vi "Main_MnE.vi"() -> ()   [LabVIEW 2019]
uses:
  Devices/NI Board/cDAQ-9269 AO/Set_AO_Wave-config.ctl
  _ctrl/DL950_config.ctl
  _ctrl/BP4610_config.ctl
  _ctrl/DSP_config.ctl
  _ctrl/Error list.ctl
  _ctrl/cDAQ-9269 Config.ctl
  Devices/NI Board/cDAQ-9221 AI/Set_NIAI.ctl
  Durability/sequence_single.ctl
  Durability/Tap_main2.ctl
  Durability/Capacitor/error_rc.ctl
  Durability/Capacitor/measure_rc.ctl
  Durability/Capacitor/cap_config.ctl
  Durability/Breakdown-Spec.ctl
  Durability/Capacitor/Judge_RC.ctl
  Durability/common/Test Mode.ctl
  Durability/Register/data_contR.ctl
  Durability/Register/measure_reg.ctl
  Durability/common/result.ctl
  _ctrl/init-r-stop.ctl
  _ctrl/create-rw-close.ctl
  SubVIs/common/cmd_tablecnt.ctl
  Durability/common/cmd_ch act.ctl
  Durability/common/def_chact.ctl
  _ctrl/rw.ctl
  Durability/common/ref_all.ctl
  SubVIs/common/ref.ctl
  Durability/common/ui_dev-operator.ctl
  SubVIs/common/_ctrl/system-status.ctl
  _ctrl/init-r-w.ctl
  Durability/common/infor_testcycle.ctl
  Durability/common/cmd_TestParaSave.ctl
  Durability/common/UI dev-operator.ctl
  SubVIs/Log-in/cmd_logInfor.ctl
  _ctrl/start.ctl
  _ctrl/DSP_action.ctl
  _ctrl/BP4610_cmd.ctl
  _ctrl/init-w-close.ctl
  Devices/NI Board/cDAQ-9476 DO/cnt_do.ctl
  Devices/NI Board/cDAQ-9476 DO/cnt_Relay.ctl
  SubVIs/common/hw-control.ctl
  Durability/common/hwsetting.ctl
  SubVIs/cmd_timer.ctl
  _ctrl/fgv_DL950.ctl
  Durability/common/log save type.ctl
  Devices/NI Board/cDAQ-9269 AO/type_signal.ctl
  _ctrl/fgv_Main_q.ctl
  SubVIs/common/Glob_Ref.vi
  SubVIs/common/Glob_setting.vi
  Durability/common/Global 1.vi
  Durability/common/Global_params.vi
panel:
  in  "\"시험모드\" 파일이름 생성 무시(Ignore)":bool
  in  "ES 규격시험 선택":T1=enum."6.3.2 저온 작동/방치 시험"
  in  "paste":bool
  in  "copy":bool
  in  "Button":bool
  in  "Disabled":T2(ring)
  out "Label.Text":string
  in  "index":i32=1
  out "사이클 회수(현재)":u32
  out "사이클 회수(세팅)":u32
  out "종료시간":string
  out "경과시간":string
  out "시작시간":string
  out "HW error":T3
  out "H/W Status":string
  in  "debug":bool caption="."
  out "캡충전전압[V]":dbl(slide)=-0.07053543199999908 scale=0.0..800.0
  in  "Status":string
  out "반복 회수(세팅)":u32=1
  in  "PinR 4":bool
  in  "PinR 5":bool
  in  "PinR 6":bool
  in  "PoutR 4":bool
  in  "PoutR 5":bool
  in  "PoutR 6":bool
  out "ch 6":bool
  out "ch 5":bool
  out "ch 4":bool
  in  "Shutdown":bool
  in  "RC setting":bool
  in  "BP4610 off":bool
  in  "AO 0v":bool
  in  "BP4610 on":bool
  in  "AO 12v":bool
  in  "relay all off":bool
  in  "Graph":bool
  in  "set_DLM5058":bool
  in  "HW config":bool
  out "Waveform":cluster{"l":dbl, "dt":dbl, "Y":dbl[][]}(graph)
  out "채널":u8=1
  out "Operation stutus 0":bool
  in  "시험 모드":T4
  in  "저항부하":bool
  in  "캐패시터부하":bool
  in  "B-수명 1":bool
  in  "B-수명 2":bool
  in  "B-수명 3":bool
  out "dt(ms)_finish":u32
  out "dt(ms)_hw":u32
  in  "file renew[Hr]":i32
  in  "Main":bool
  in  "Stop_RC":bool
  in  "RCstart":bool
  in  "Oscilloscope_Res":cluster{"Record Len":i32, "Time Div":u16}={"Record Len"=4, "Time Div"=20} {"Time Div" items=["10m"=10, "20ms"=20, "50ms"=50, "100ms"=100, "200ms"=200, "500ms"=500, "1s"=1000, "2s"=2000]; "Record Len" items=["10k", "25k", "50k", "100k", "250k", "500k", "1M", "2.5M", "5M", "10M", "25M", "50M", "100M", "250M", "500M", "1G", "2G", "4G", "5G", "10G", "20G", "50G"]}
  in  "Control Signal_Res":T5={"Freq"=1.0, "level[V]"=12.0, "duty"=10.0, "On time[ms]"=300.0}
  in  "Oscilloscope_b1":cluster{"Record Len":i32, "Time Div":u16}={"Record Len"=4, "Time Div"=20} {"Time Div" items=["10m"=10, "20ms"=20, "50ms"=50, "100ms"=100, "200ms"=200, "500ms"=500, "1s"=1000, "2s"=2000]; "Record Len" items=["10k", "25k", "50k", "100k", "250k", "500k", "1M", "2.5M", "5M", "10M", "25M", "50M", "100M", "250M", "500M", "1G", "2G", "4G", "5G", "10G", "20G", "50G"]}
  in  "Control Signal_b1":T5={"Freq"=50.0, "level[V]"=12.0, "duty"=50.0, "On time[ms]"=50.0}
  in  "Control Signal_B2":T5={"Freq"=50.0, "level[V]"=12.0, "duty"=50.0, "On time[ms]"=50.0}
  in  "Oscilloscope_B2":cluster{"Record Len":i32, "Time Div":u16}={"Record Len"=4, "Time Div"=20} {"Time Div" items=["10m"=10, "20ms"=20, "50ms"=50, "100ms"=100, "200ms"=200, "500ms"=500, "1s"=1000, "2s"=2000]; "Record Len" items=["10k", "25k", "50k", "100k", "250k", "500k", "1M", "2.5M", "5M", "10M", "25M", "50M", "100M", "250M", "500M", "1G", "2G", "4G", "5G", "10G", "20G", "50G"]}
  in  "Control Signal_B3":T5={"Freq"=50.0, "level[V]"=12.0, "duty"=50.0, "On time[ms]"=50.0}
  in  "Oscilloscope_B3":cluster{"Record Len":i32, "Time Div":u16}={"Record Len"=4, "Time Div"=20} {"Time Div" items=["10m"=10, "20ms"=20, "50ms"=50, "100ms"=100, "200ms"=200, "500ms"=500, "1s"=1000, "2s"=2000]; "Record Len" items=["10k", "25k", "50k", "100k", "250k", "500k", "1M", "2.5M", "5M", "10M", "25M", "50M", "100M", "250M", "500M", "1G", "2G", "4G", "5G", "10G", "20G", "50G"]}
  in  "exit":bool
  in  "stop":bool
  in  "B3start":bool
  in  "B2start":bool
  in  "B1start":bool
  in  "Rloadstart":bool
  in  "single start":bool
  in  "Single sequence":T6
  in  "HW check":bool
  in  "Setting":bool
  in  "Tab_menu-select":T7=enum."Test"
  in  "Tab Control_manual":T8(tab)=enum."NI AI"
  in  "Output_LV":bool
  in  "led red":bool
  in  "led yellow":bool
  in  "led green":bool
  in  "led buz":bool
  in  "led purple":bool
  out "Voltage_Charge":dbl(slide)=-0.07053543199999908 scale=0.0..800.0
  in  "AO_Level":dbl caption="Level"
  in  "AO":bool
  in  "PinR 1":bool
  in  "PinR 2":bool
  in  "PinR 3":bool
  in  "PoutR 1":bool
  in  "PoutR 2":bool
  in  "PoutR 3":bool
  in  "Input Pwr":bool
  in  "Output_HV":bool
  in  "Discharge R":bool
  in  "Clear scope graph":bool
  in  "Trigger_single":bool
  in  "ReadItem_DLM5058":bool
  in  "ResetItem_DLM5058":bool
  in  "TabControl_DLM":enum32{" TEST DL950", " SET DL950", "Test_cmd"}(tab)=enum." SET DL950"
  out "DL950 items":dbl[][](array[numeric]) format="%.2f"
  out "DL950 wfm":waveform(dbl)[](graph)
  in  "DL950_config":T9={"Timeout"=0, "Time Div"=18, "Acq Mode"=0, "Record Len"=4, "Record Num"=0, "Start Point"=0, "End Poin"=60000, "Visa"="TCPIP0::192.168.0.101::inst0::INSTR", "Config Voltage"=[{"Enable"=TRUE, "Ch"=1, "V Div"=15, "Coupling"=1, "Probe"=35, "Act.Items"=FALSE, "items"=[]}, {"Enable"=TRUE, "Ch"=2, "V Div"=23, "Coupling"=1, "Probe"=35, "Act.Items"=FALSE, "items"=[]}, {"Enable"=TRUE, "Ch"=3, "V Div"=23, "Coupling"=1, "Probe"=35, "Act.Items"=FALSE, "items"=[]}, {"Enable"=TRUE, "Ch"=4, "V Div"=23, "Coupling"=1, "Probe"=35, "Act.Items"=FALSE, "items"=[]}, {"Enable"=TRUE, "Ch"=5, "V Div"=6, "Coupling"=1, "Probe"=3, "Act.Items"=FALSE, "items"=[]}, {"Enable"=TRUE, "Ch"=6, "V Div"=15, "Coupling"=1, "Probe"=21, "Act.Items"=FALSE, "items"=[]}], "Trigger on"=TRUE, "Trigger Level"=5.0, "Reset"=FALSE, "Config Temp"=[{"Channel"=9, "Burn Out"=FALSE, " Type "=0}, {"Channel"=10, "Burn Out"=FALSE, " Type "=0}, {"Channel"=11, "Burn Out"=FALSE, " Type "=0}, {"Channel"=12, "Burn Out"=FALSE, " Type "=0}, {"Channel"=13, "Burn Out"=FALSE, " Type "=0}, {"Channel"=14, "Burn Out"=FALSE, " Type "=0}], "Trig Mode"=0, "Trig Pos"=10.0, "Trigger Slope"=0, "Trigger Source "=1, "Trig Start -5"=-5.0, "End 5"=5.0} {"End 5" format="%.2g"; "Trig Start -5" format="%.2f"; "Trigger Source" items=["", "CH1", "CH2", "CH3", "CH4", "CH5", "CH6", "CH7", "CH8", "CH9", "CH10", "CH11", "CH12", "CH13", "CH14", "CH15", "CH16", "RMATH1", "RMATH2", "RMATH3", "RMATH4", "RMATH5", "RMATH6", "RMATH7", "RMATH8", "RMATH9", "RMATH10", "RMATH11", "RMATH12", "RMATH13", "RMATH14", "RMATH15", "RMATH16"]; "Trigger Slope" items=["Rising", "Falling", "Both"]; "Trig Pos" format="%.1f"; "Trig Mode" items=["Normal", "Auto", "Auto Level", "Single", "Single(N)", "On Start", "No Set"]; "Config Temp"."Type" items=["K", "E", "J", "T", "L", "U", "N", "R", "S", "B", "W", "Au7fe"]; "Config Temp"."Channel" items=["", "CH1", "CH2", "CH3", "CH4", "CH5", "CH6", "CH7", "CH8", "CH9", "CH10", "CH11", "CH12", "CH13", "CH14", "CH15", "CH16"]; "Trigger Level" format="%.3p"; "Config Voltage"."items" items=["Peak to Peak", "Amplitude", "Max", "Min", "High", "Low", "Average", "Middle", "Rms", "Standard Deviation", "+Overshoot", "-Overshoot", "Rise", "Fall", "Frequency", "Period", "+Width", "-Width", "Duty Cycle", "Pulse Count", "Burst1 Width", "Burst2 Width", "Average Frequency", "Average Period", "Int1TY", "Int2TY"]; "Config Voltage"."Probe" items=["1:1", "2:1", "5:1", "10:1", "20:1", "50:1", "100:1", "200:1", "500:1", "1000:1", "2000:1", "5000:1", "10k:1", "20k:1", "50k:1", "0.1A:1V", "0.2A:1V", "0.5A:1V", "1A:1V", "2A:1V", "5A:1V", "10A:1V", "20A:1V", "50A:1V", "100A:1V", "200A:1V", "250A:1V", "400A:1V", "500A:1V", "1kA:1V", "2kA:1V", "5kA:1V", "10kA:1V", "20kA:1V", "50kA:1V", "NoSet"]; "Config Voltage"."Ch" items=["None", "CH1", "CH2", "CH3", "CH4", "CH5", "CH6", "CH7", "CH8", "CH9", "CH10", "CH11", "CH12", "CH13", "CH14", "CH15", "CH16", "MATH1", "MATH2", "MATH3", "MATH4", "MATH5", "MATH6", "MATH7", "MATH8", "EVENT"]; "Config Voltage"."Coupling" items=["AC", "DC", "Ground", "AC-RMS", "DC-RMS"]; "Config Voltage"."V Div" items=["0.1m", "0.2m", "0.5m", "1m", "2m", "5m", "10m", "20m", "50m", "100m", "200m", "500m", "1", "2", "4", "5", "8", "10", "20", "40", "50", "80", "100", "200", "400", "500", "800", "1k", "2k", "4k", "5k", "8k", "10k", "20k", "25k", "50k", "100k", "250k", "500k", "1000k"]; "Record Len" items=["10k", "25k", "50k", "100k", "250k", "500k", "1M", "2.5M", "5M", "10M", "25M", "50M", "100M", "250M", "500M", "1G", "2G", "4G", "5G", "10G", "20G", "50G"]; "Acq Mode" items=["Normal", "Average", "Envelope"]; "Time Div" items=["100ns", "200ns", "500ns", "1us", "2us", "5us", "10us", "20us", "50us", "100us", "200us", "500us", "1ms", "2ms", "5ms", "10ms", "20ms", "50ms", "100ms", "200ms", "500ms", "1s", "2s", "3s", "4s", "5s", "6s", "10s", "20s", "30s", "1min", "2min", "3min", "4min", "5min", "6min", "10min", "12min", "30min", "1hour", "2hour", "3hour", "4hour", "5hour", "6hour", "8hour", "10hour", "12hour", "1day", "2day", "3day", "4day", "5day"]}
  out "Array_temp":T10(array[cluster])
  in  "Query_DLM5058":bool
  out "String_dl950":string
  in  "String":string
  out "DL950 read":dbl[](array[numeric])
  in  "Read":bool
  out "Time":dbl
  in  "con_DLM5058":bool
  in  "M_Start_DLM5058":bool
  in  "M_Stop_DLM5058":bool
  in  "Read_DLM5058":bool
  in  "discon_DLM5058":bool
  in  "Apply_DLM5058":bool
  in  "Apply BP4610":bool
  in  "Close BP4610":bool
  in  "Open BP4610":bool
  in  "BP4610 Config":T11={"VISA"="USB0::0x0D4A::0x0040::9426270::INSTR", "Limit-BP"={"Set"=enum."Voltage", "Voltage+[V]"=20.0, "Current+[A]"=5.0, "Voltage-[V]"=-20.0, "Current-[A]"=-5.0}, "SET BP"={"Set"=enum."Voltage", "Operation mode"=1, "Voltage[Vp-p]"=20.0, "Current[Ap-p]"=5.0, "Voltage[V]"=12.0, "Current[A]"=5.0, "Frequency[Hz]"=100.0, "Waveform"=enum."Square"}} {"SET BP"."Frequency[Hz]" min=1.0 max=100000.0 step=0.1; "SET BP"."Current[A]" min=-20.0 max=20.0 step=0.001; "SET BP"."Voltage[V]" min=-115.0 max=115.0 step=0.01; "SET BP"."Current[Ap-p]" min=0.0 max=60.0 step=0.01; "SET BP"."Voltage[Vp-p]" min=0.0 max=120.0 step=0.1; "SET BP"."Operation mode" items=["CV-INT", "CV-EXT", "CV-ADD", "CC-INT", "CC-EXT", "CC-ADD"]; "Limit-BP"."Current-[A]" min=-20.0 max=20.0 step=0.001; "Limit-BP"."Voltage-[V]" min=-115.0 max=115.0 step=0.01; "Limit-BP"."Current+[A]" min=0.0 max=60.0 step=0.01; "Limit-BP"."Voltage+[V]" min=0.0 max=120.0 step=0.1}
  in  "DSP Selection":enum32{"DSP HV", "DSP LV"}(radio)
  in  "DSP Config LV":T12={"Port"="TCPIP0::192.168.0.102::HISLIP0::INSTR", "OVP Level"=1000.0, "OCP Level"=25.0, "Current"=10.0, "Voltage"=200.0} {"OCP Level" format="%#_13g"; "OVP Level" format="%#_13g"}
  in  "read_dsp":bool
  in  "Close DSP":bool
  in  "Open DSP":bool
  in  "Set_idrc":bool
  out "Current":dbl
  out "Volt":dbl
  in  "DSP1500 Config":T12={"Port"="TCPIP0::192.168.0.102::HISLIP0::INSTR", "OVP Level"=1000.0, "OCP Level"=25.0, "Current"=10.0, "Voltage"=200.0} {"OCP Level" format="%#_13g"; "OVP Level" format="%#_13g"}
  in  "cDAQ 9269 AO config":T13={"Ch"="cDAQ9185-213AA55Mod2/ao0", "Max V"=5.0, "Min V"=-5.0, " Rate"=10000.0, "N pts"=2000, "sample mode"=10178} {"sample mode" items=["유한 샘플"=10178, "연속 샘플"=10123, "하드웨어 타이밍에 의한 단일 포인트"=12522]}
  in  "Ouptut_NIAO":bool
  in  "Apply AO":bool
  in  "AO_Wave-config":T14={"offset"=6.0, "Samples"=10000, "duty"=50.0, "Rate"=10000.0, "wfm"={"Freq"=50.0, "Amp"=6.0, "Type"=enum."Square Wave"}}
  out "Means":dbl[](array[numeric])=[-0.07053543199999908, -0.28297513060000157, -0.30258228640000107, -0.12714499130000104, -0.3520088408000025, -0.6333380023000008, -0.2967813385000024, 0.16819898919999848] format="%.3f"
  out "AI Graph":waveform(dbl)[](graph)=[{"t0"=timestamp(3812621198.0337114 s since 1904-01-01), "dt"=9.999999999999999e-05, "Y"=array[1000 elements], "attributes"=variant("NI_ChannelName"=variant(string "cDAQ9185-213AA55Mod3/ai0"), "NI_UnitDescription"=variant(string "Volts"))}, {"t0"=timestamp(3812621198.033723 s since 1904-01-01), "dt"=9.999999999999999e-05, "Y"=array[1000 elements], "attributes"=variant("NI_ChannelName"=variant(string "cDAQ9185-213AA55Mod3/ai1"), "NI_UnitDescription"=variant(string "Volts"))}, {"t0"=timestamp(3812621198.0337343 s since 1904-01-01), "dt"=9.999999999999999e-05, "Y"=array[1000 elements], "attributes"=variant("NI_ChannelName"=variant(string "cDAQ9185-213AA55Mod3/ai2"), "NI_UnitDescription"=variant(string "Volts"))}, {"t0"=timestamp(3812621198.0337453 s since 1904-01-01), "dt"=9.999999999999999e-05, "Y"=array[1000 elements], "attributes"=variant("NI_ChannelName"=variant(string "cDAQ9185-213AA55Mod3/ai3"), "NI_UnitDescription"=variant(string "Volts"))}, {"t0"=timestamp(3812621198.0337567 s since 1904-01-01), "dt"=9.999999999999999e-05, "Y"=array[1000 elements], "attributes"=variant("NI_ChannelName"=variant(string "cDAQ9185-213AA55Mod3/ai4"), "NI_UnitDescription"=variant(string "Volts"))}, {"t0"=timestamp(3812621198.0337677 s since 1904-01-01), "dt"=9.999999999999999e-05, "Y"=array[1000 elements], "attributes"=variant("NI_ChannelName"=variant(string "cDAQ9185-213AA55Mod3/ai5"), "NI_UnitDescription"=variant(string "Volts"))}, {"t0"=timestamp(3812621198.033779 s since 1904-01-01), "dt"=9.999999999999999e-05, "Y"=array[1000 elements], "attributes"=variant("NI_ChannelName"=variant(string "cDAQ9185-213AA55Mod3/ai6"), "NI_UnitDescription"=variant(string "Volts"))}, {"t0"=timestamp(3812621198.0337906 s since 1904-01-01), "dt"=9.999999999999999e-05, "Y"=array[1000 elements], "attributes"=variant("NI_ChannelName"=variant(string "cDAQ9185-213AA55Mod3/ai7"), "NI_UnitDescription"=variant(string "Volts"))}]
  in  "Stop_AI":bool
  in  "Read_AI":bool
  in  "cDAQ 9221 Config":T15={"input terminal"=10083, "minimum value"=-60.0, "maximum value"=60.0, "number of samples"=1000, "rate"=10000.0, "sample mode"=10123, "physical channels"="cDAQ9185-213AA55Mod3/ai0:7"} {"sample mode" items=["Finite Samples"=10178, "Continuous Samples"=10123, "Hardware Timed Single Point"=12522]; "rate" format="%0.2f"; "maximum value" format="%^.2e"; "minimum value" format="%^.2e"; "input terminal" items=["default"=-1, "RSE"=10083, "NRSE"=10078, "Differential"=10106, "Pseudodifferential"=12529]}
  in  "DO Initialize":bool
  in  "cDAQ-9467 Config":tag="cDAQ9185-213AA55Mod1/port0/line0:31"
  in  "Tab Control":T16(tab)
  out "DL950_config load":T9={"Timeout"=10000, "Time Div"=17, "Acq Mode"=0, "Record Len"=4, "Record Num"=0, "Start Point"=0, "End Poin"=1000, "Visa"="", "Config Voltage"=[{"Enable"=TRUE, "Ch"=1, "V Div"=26, "Coupling"=1, "Probe"=3, "Act.Items"=FALSE, "items"=[]}, {"Enable"=TRUE, "Ch"=2, "V Div"=20, "Coupling"=1, "Probe"=3, "Act.Items"=FALSE, "items"=[]}, {"Enable"=TRUE, "Ch"=3, "V Div"=20, "Coupling"=1, "Probe"=3, "Act.Items"=FALSE, "items"=[]}, {"Enable"=TRUE, "Ch"=4, "V Div"=20, "Coupling"=1, "Probe"=3, "Act.Items"=FALSE, "items"=[]}, {"Enable"=TRUE, "Ch"=5, "V Div"=20, "Coupling"=1, "Probe"=3, "Act.Items"=FALSE, "items"=[]}, {"Enable"=TRUE, "Ch"=6, "V Div"=20, "Coupling"=1, "Probe"=3, "Act.Items"=FALSE, "items"=[]}], "Trigger on"=FALSE, "Trigger Level"=0.0, "Reset"=FALSE, "Config Temp"=[{"Channel"=1, "Burn Out"=TRUE, " Type "=0}, {"Channel"=2, "Burn Out"=TRUE, " Type "=0}, {"Channel"=3, "Burn Out"=TRUE, " Type "=0}, {"Channel"=4, "Burn Out"=TRUE, " Type "=0}, {"Channel"=5, "Burn Out"=TRUE, " Type "=0}, {"Channel"=6, "Burn Out"=TRUE, " Type "=0}], "Trig Mode"=1, "Trig Pos"=50.0, "Trigger Slope"=0, "Trigger Source "=1, "Trig Start -5"=-5.0, "End 5"=5.0} {"End 5" format="%.2g"; "Trig Start -5" format="%.2f"; "Trigger Source" items=["", "CH1", "CH2", "CH3", "CH4", "CH5", "CH6", "CH7", "CH8", "CH9", "CH10", "CH11", "CH12", "CH13", "CH14", "CH15", "CH16", "RMATH1", "RMATH2", "RMATH3", "RMATH4", "RMATH5", "RMATH6", "RMATH7", "RMATH8", "RMATH9", "RMATH10", "RMATH11", "RMATH12", "RMATH13", "RMATH14", "RMATH15", "RMATH16"]; "Trigger Slope" items=["Rising", "Falling", "Both"]; "Trig Pos" format="%.1f"; "Trig Mode" items=["Normal", "Auto", "Auto Level", "Single", "Single(N)", "On Start", "No Set"]; "Config Temp"."Type" items=["K", "E", "J", "T", "L", "U", "N", "R", "S", "B", "W", "Au7fe"]; "Config Temp"."Channel" items=["", "CH1", "CH2", "CH3", "CH4", "CH5", "CH6", "CH7", "CH8", "CH9", "CH10", "CH11", "CH12", "CH13", "CH14", "CH15", "CH16"]; "Trigger Level" format="%.3p"; "Config Voltage"."items" items=["Peak to Peak", "Amplitude", "Max", "Min", "High", "Low", "Average", "Middle", "Rms", "Standard Deviation", "+Overshoot", "-Overshoot", "Rise", "Fall", "Frequency", "Period", "+Width", "-Width", "Duty Cycle", "Pulse Count", "Burst1 Width", "Burst2 Width", "Average Frequency", "Average Period", "Int1TY", "Int2TY"]; "Config Voltage"."Probe" items=["1:1", "2:1", "5:1", "10:1", "20:1", "50:1", "100:1", "200:1", "500:1", "1000:1", "2000:1", "5000:1", "10k:1", "20k:1", "50k:1", "0.1A:1V", "0.2A:1V", "0.5A:1V", "1A:1V", "2A:1V", "5A:1V", "10A:1V", "20A:1V", "50A:1V", "100A:1V", "200A:1V", "250A:1V", "400A:1V", "500A:1V", "1kA:1V", "2kA:1V", "5kA:1V", "10kA:1V", "20kA:1V", "50kA:1V", "NoSet"]; "Config Voltage"."Ch" items=["None", "CH1", "CH2", "CH3", "CH4", "CH5", "CH6", "CH7", "CH8", "CH9", "CH10", "CH11", "CH12", "CH13", "CH14", "CH15", "CH16", "MATH1", "MATH2", "MATH3", "MATH4", "MATH5", "MATH6", "MATH7", "MATH8", "EVENT"]; "Config Voltage"."Coupling" items=["AC", "DC", "Ground", "AC-RMS", "DC-RMS"]; "Config Voltage"."V Div" items=["0.1m", "0.2m", "0.5m", "1m", "2m", "5m", "10m", "20m", "50m", "100m", "200m", "500m", "1", "2", "4", "5", "8", "10", "20", "40", "50", "80", "100", "200", "400", "500", "800", "1k", "2k", "4k", "5k", "8k", "10k", "20k", "25k", "50k", "100k", "250k", "500k", "1000k"]; "Record Len" items=["10k", "25k", "50k", "100k", "250k", "500k", "1M", "2.5M", "5M", "10M", "25M", "50M", "100M", "250M", "500M", "1G", "2G", "4G", "5G", "10G", "20G", "50G"]; "Acq Mode" items=["Normal", "Average", "Envelope"]; "Time Div" items=["100ns", "200ns", "500ns", "1us", "2us", "5us", "10us", "20us", "50us", "100us", "200us", "500us", "1ms", "2ms", "5ms", "10ms", "20ms", "50ms", "100ms", "200ms", "500ms", "1s", "2s", "3s", "4s", "5s", "6s", "10s", "20s", "30s", "1min", "2min", "3min", "4min", "5min", "6min", "10min", "12min", "30min", "1hour", "2hour", "3hour", "4hour", "5hour", "6hour", "8hour", "10hour", "12hour", "1day", "2day", "3day", "4day", "5day"]}
  out "BP4610 Config load":T11={"VISA"="", "Limit-BP"={"Set"=enum."Current", "Voltage+[V]"=20.0, "Current+[A]"=5.0, "Voltage-[V]"=-20.0, "Current-[A]"=-5.0}, "SET BP"={"Set"=enum."FREQ/WAVE", "Operation mode"=0, "Voltage[Vp-p]"=0.0, "Current[Ap-p]"=0.0, "Voltage[V]"=0.0, "Current[A]"=0.0, "Frequency[Hz]"=1.0, "Waveform"=enum."Sine"}} {"SET BP"."Frequency[Hz]" min=1.0 max=100000.0 step=0.1; "SET BP"."Current[A]" min=-20.0 max=20.0 step=0.001; "SET BP"."Voltage[V]" min=-115.0 max=115.0 step=0.01; "SET BP"."Current[Ap-p]" min=0.0 max=60.0 step=0.01; "SET BP"."Voltage[Vp-p]" min=0.0 max=120.0 step=0.1; "SET BP"."Operation mode" items=["CV-INT", "CV-EXT", "CV-ADD", "CC-INT", "CC-EXT", "CC-ADD"]; "Limit-BP"."Current-[A]" min=-20.0 max=20.0 step=0.001; "Limit-BP"."Voltage-[V]" min=-115.0 max=115.0 step=0.01; "Limit-BP"."Current+[A]" min=0.0 max=60.0 step=0.01; "Limit-BP"."Voltage+[V]" min=0.0 max=120.0 step=0.1}
  out "DSP1950 Config load":T12={"Port"="TCPIP0::192.168.0.14::HISLIP0::INSTR", "OVP Level"=0.0, "OCP Level"=0.0, "Current"=0.0, "Voltage"=0.0} {"OCP Level" format="%#_13g"; "OVP Level" format="%#_13g"}
  out "DSP1950 Config LV":T12={"Port"="TCPIP0::192.168.0.14::HISLIP0::INSTR", "OVP Level"=0.0, "OCP Level"=0.0, "Current"=0.0, "Voltage"=0.0} {"OCP Level" format="%#_13g"; "OVP Level" format="%#_13g"}
  out "cDAQ-9221 Config":T15={"input terminal"=10083, "minimum value"=-60.0, "maximum value"=60.0, "number of samples"=1000, "rate"=10000.0, "sample mode"=10123, "physical channels"=""} {"sample mode" items=["Finite Samples"=10178, "Continuous Samples"=10123, "Hardware Timed Single Point"=12522]; "rate" format="%0.2f"; "maximum value" format="%^.2e"; "minimum value" format="%^.2e"; "input terminal" items=["default"=-1, "RSE"=10083, "NRSE"=10078, "Differential"=10106, "Pseudodifferential"=12529]}
  out "cDAQ-9467 Config load":tag
  out "cDAQ-9269 AO Config":T13={"Ch"="cDAQ1Mod1/ao0", "Max V"=5.0, "Min V"=-5.0, " Rate"=1000.0, "N pts"=100, "sample mode"=10178} {"sample mode" items=["유한 샘플"=10178, "연속 샘플"=10123, "하드웨어 타이밍에 의한 단일 포인트"=12522]}
  out "config 2":T13={"Ch"="cDAQ1Mod1/ao0", "Max V"=5.0, "Min V"=-5.0, " Rate"=1000.0, "N pts"=100, "sample mode"=10178} {"sample mode" items=["유한 샘플"=10178, "연속 샘플"=10123, "하드웨어 타이밍에 의한 단일 포인트"=12522]}
  out "AO_Wave-config load":T14
  in  "Tab Control_debug":enum32{"Main", "debug"}(tab)
  out "Operation Status 2":string
  out "스위칭 경과 시간(초)":dbl
  out "미작동 경과시간(초)":dbl format="%<%H:%M:%S%1u>t"
  out "스위칭 채널 개 수[N]":i32=1
  out "전체 사이클(%)":u8(slide)=255 scale=0.0..100.0
  out "작동시간(초)":dbl format="%<%H:%M:%S%1u>t"
  out "ch 1":bool
  out "ch 2":bool
  out "ch 3":bool
  in  "Multicolumn Listbox":i32(listbox)
  out "Operation Status":string
  out "1사이클 진행률(%)":u8(slide)=255 scale=0.0..100.0
  in  "Tab Control 2":T17(tab)
  out "read_dl950":string
  out "T2":dbl
  out "T1":dbl
  out "OCP Level":dbl
  out "OVP Level":dbl
  out "출력전류[A]":dbl
  out "출력전압[V]":dbl
  out "TestType":T6
  out "N pts":i32
  out "Min V":dbl
  out "Max V":dbl
  out "sample mode":i32(ring)=10178 caption="샘플 모드" items=["유한 샘플"=10178, "연속 샘플"=10123, "하드웨어 타이밍에 의한 단일 포인트"=12522]
  out "Rate":dbl
  out "Ch":tag
  out "DSP Selection 2":enum32{"DSP HV", "DSP LV"}(radio)
  out "da950_array":dbl[](array[numeric])
  out "result":T18=enum."Completion"
  out "950Trigger":i32 format="%.0x"
  out "OFF Time out":u32
  out "OFF Time in":u32
  out "NumData_OLV":dbl
  out "Control Signal_LV":T5={"Freq"=50.0, "level[V]"=12.0, "duty"=50.0, "On time[ms]"=50.0}
  out "Time Div_Init":u16
  out "Time Div_set":u16
  out "Time Div":u32
  out "trig delay":u32=3000
  out "trig delay_ready":u32=3000
  out "Testconfig out":T19={"Test Mode"=enum."6.3.2 저온 작동/방치 시험", "ON time[ms]"=500.0, "OFF time[ms]"=10000.0, "1. 작동시간[분]"=10000.0, "2. 미작동시간[분]"=10000.0, "3. 작동시간[분]"=10000.0, "level[V]"=12.0, "duty"=20.0, "Freq"=1.0, "Voltage+[V]"=20.0, "Voltage-[V]"=-20.0, "Current+[A]"=5.0, "Current-[A]"=-5.0, "출력전압[V]"=0.0, "출력전류[A]"=0.0, "OVP Level"=0.0, "OCP Level"=0.0, "Time Div"=0, "Record Len"=4, "방전 기준[V]"=0.0, "Repeate (Each Ch)"=1, "Cycle[N]"=1, "작동간격[분]"=10000.0, "TrigPos[%]"=0.0, "시험시간[분]"=10000.0} {"시험시간[분]" min=1.0; "작동간격[분]" min=1.0; "3. 작동시간[분]" min=1.0; "2. 미작동시간[분]" min=1.0; "1. 작동시간[분]" min=1.0; "Time Div" items=["10m", "20ms", "50ms", "100ms", "200ms", "500ms", "1s", "2s", "5s", "10s", "20s", "30s", "1min", "2min", "5min"]; "OFF time[ms]" min=10000.0 max=1000000.0; "Current-[A]" min=-20.0 max=20.0 step=0.001; "Voltage-[V]" min=-115.0 max=115.0 step=0.01; "Current+[A]" min=0.0 max=60.0 step=0.01; "Voltage+[V]" min=0.0 max=120.0 step=0.1; "OCP Level" format="%#_13g"; "OVP Level" format="%#_13g"; "Record Len" items=["10k", "25k", "50k", "100k", "250k", "500k", "1M", "2.5M", "5M", "10M", "25M", "50M", "100M", "250M", "500M", "1G", "2G", "4G", "5G", "10G", "20G", "50G"]; "ON time[ms]" min=50.0 max=2000000.0}
  out "measure_LV 동작":T20
  out "measure_rc 동작":T21 {"부하전압(고장)" format="%.3f"; "출력전류 평균 63%" format="%.3f"; "출력전압 - 평균 63%" format="%.3f"; "Failing Time 37%" format="%.3f"; "Rising Time 98%" format="%.3f"; "Rising Time 63%" format="%.3f"; "접촉저항" format="%.1f"; "출력전류 RMS" format="%.3f"; "출력전압 + 평균 63%" format="%.3f"; "입력전류 RMS" format="%.3f"; "온도" format="%.3f"; "방전전압" format="%.3f"; "충전전류 37초" format="%.3f"; "충전전압 63초" format="%.3f"; "충전전압 98초" format="%.3f"; "출력카운트" format="%.3f"; "입력카운트" format="%.3f"}
  out "measure_ContR Out":T22
  out "Error":T23
  out "AO Waveform Graph":waveform(dbl)(graph)
  out "error out":errorcluster
  out "error out wait Ao":errorcluster
  out "error out task stop":errorcluster
  out "data_relay":bool[](array[boolean])
  in  "시험환경세팅":bool
  in  "시험규격":bool
  in  "Apply":bool
  in  "Password":string
  in  "logout":bool
  in  "login":bool
  in  "Log path":path=path "C:/test_cfg"
  in  "시험명":string="relay"
  in  "Breakdown-Spec":T24={"제어단 단선 Irms[mA](이하)"=5.0, "제어단 특성 전류 Irms[mA] Max"=50.0, "제어단 특성 전류 Irms[mA] Min"=10.0, "출력단 단선 Irms[mA](이하)"=5.0, "출력단 특성 전류 Irms[mA]  Max"=3700.0, "출력단 특성전류 Irms[mA]  Min"=1000.0, "온도[degree]"=0.0} {"출력단 특성전류 Irms[mA]  Min" format="%#.2f"; "출력단 특성 전류 Irms[mA]  Max" format="%#.2f"; "출력단 단선 Irms[mA](이하)" format="%#.2f"; "제어단 특성 전류 Irms[mA] Min" format="%#.2f"; "제어단 특성 전류 Irms[mA] Max" format="%#.2f"; "제어단 단선 Irms[mA](이하)" format="%#.2f"}
  in  "Testconfig":T19={"Test Mode"=enum."6.3.2 저온 작동/방치 시험", "ON time[ms]"=200.0, "OFF time[ms]"=500.0, "1. 작동시간[분]"=10000.0, "2. 미작동시간[분]"=10000.0, "3. 작동시간[분]"=10000.0, "level[V]"=12.0, "duty"=20.0, "Freq"=1.0, "Voltage+[V]"=20.0, "Voltage-[V]"=-20.0, "Current+[A]"=5.0, "Current-[A]"=-5.0, "출력전압[V]"=200.0, "출력전류[A]"=10.0, "OVP Level"=0.0, "OCP Level"=0.0, "Time Div"=2, "Record Len"=5, "방전 기준[V]"=0.0, "Repeate (Each Ch)"=3, "Cycle[N]"=1, "작동간격[분]"=10000.0, "TrigPos[%]"=0.0, "시험시간[분]"=1.0} {"시험시간[분]" min=1.0; "작동간격[분]" min=1.0; "3. 작동시간[분]" min=1.0; "2. 미작동시간[분]" min=1.0; "1. 작동시간[분]" min=1.0; "Time Div" items=["10m", "20ms", "50ms", "100ms", "200ms", "500ms", "1s", "2s", "5s", "10s", "20s", "30s", "1min", "2min", "5min"]; "OFF time[ms]" min=10000.0 max=1000000.0; "Current-[A]" min=-20.0 max=20.0 step=0.001; "Voltage-[V]" min=-115.0 max=115.0 step=0.01; "Current+[A]" min=0.0 max=60.0 step=0.01; "Voltage+[V]" min=0.0 max=120.0 step=0.1; "OCP Level" format="%#_13g"; "OVP Level" format="%#_13g"; "Record Len" items=["10k", "25k", "50k", "100k", "250k", "500k", "1M", "2.5M", "5M", "10M", "25M", "50M", "100M", "250M", "500M", "1G", "2G", "4G", "5G", "10G", "20G", "50G"]; "ON time[ms]" min=50.0 max=2000000.0}
  in  "Test Judgement":T25={"전압 63%[mS] Min"=25.5, "전압 98%[mS] Min"=140.0, "전류 37%[mS] Min"=25.5, "접촉저항[mOhm] Min"=1.0, "출력전류 Irms[mA] Min"=1500.0, "전압 63%[mS] Max"=5.0, "전압 98%[mS] Max"=5.0, "전류 37%[mS] Max"=5.0, "접촉저항[mOhm] Max"=0.5, "출력전류 Irms[mA] Max"=500.0}
  in  "채널선택":T26={"Ch 1"=TRUE, "Ch 2"=TRUE, "Ch 3"=TRUE, "Ch 4"=TRUE, "Ch 5"=TRUE, "Ch 6"=TRUE}
  in  "Manual":bool
  # "운영 상태"
  # "Pre Charge Relay 메카환경 신뢰성"
  # "ver.02"
  # "캡 충전 상태"
  # "시스템 로그"
  # "시간 정보"
  # "ES 규격 시험 정보"
  # "Relay4"
  # "Relay5"
  # "Relay6"
  # "디바이스 상태"
  # "C 전압1"
  # "C 전압2"
  # "출력전압(+)"
  # "출력전압(-)"
  # "입력전류"
  # "출력전류"
  # "Limit-BP\nV+ 20 C 5\nV- -20 C- -5\n\nSET BP\nVp 20, C 5, Square\nV 12, C5, 100"
  # "102::HISLIP0::INSTR\n\nOVP 1000, OCP 25\nV 400, C 20"
  # "102::HISLIP0::INSTR\n\nOVP 1000, OCP 25\nV 400, C 20"
  # "a0\n5\n-5\n10000\n5000\n유한샘플"
  # "10000, W freq 50\n10000, Amp 6\n6, Square\n50"
  # "RSE\n-60\n60\n1000\n10000\nCont"
  # "C 전압1"
  # "C 전압2"
  # "출력전압(+)"
  # "출력전압(-)"
  # "입력전류"
  # "출력전류"
  # "채널 스위칭 정보"
  # "작동/미작동 시간(초)"
  # "시험 진행률"
  # "제어단 전압"
  # "출력단 전원"
  # "DL950"
  # "Discharge"
  # "Test Cycle"
  # "작동 설정"
  # "R Laoad"
  # "R out1"
  # "R out2"
  # "R out3"
  # "R out4"
  # "R out5"
  # "R out6"
  # "R in1"
  # "R in2"
  # "R in3"
  # "R in4"
  # "R in5"
  # "R in6"
  # "Red"
  # "Yellow"
  # "Green"
  # "Buz"
  # "Purple"
  # "관리자 기능"
  # "데이터 저장"
  # "고장진단 기준"
  # "테스트 환경"
  # "테스트 체널"
  # "테스트 기준"
  # "제어단"
  # "출력단"
  # "온도기준"
  # "제어단 전압"
  # "출력단 전원"
  # "DL950"
  # "Discharge"
  # "Test Cycle"
  # "작동 설정"
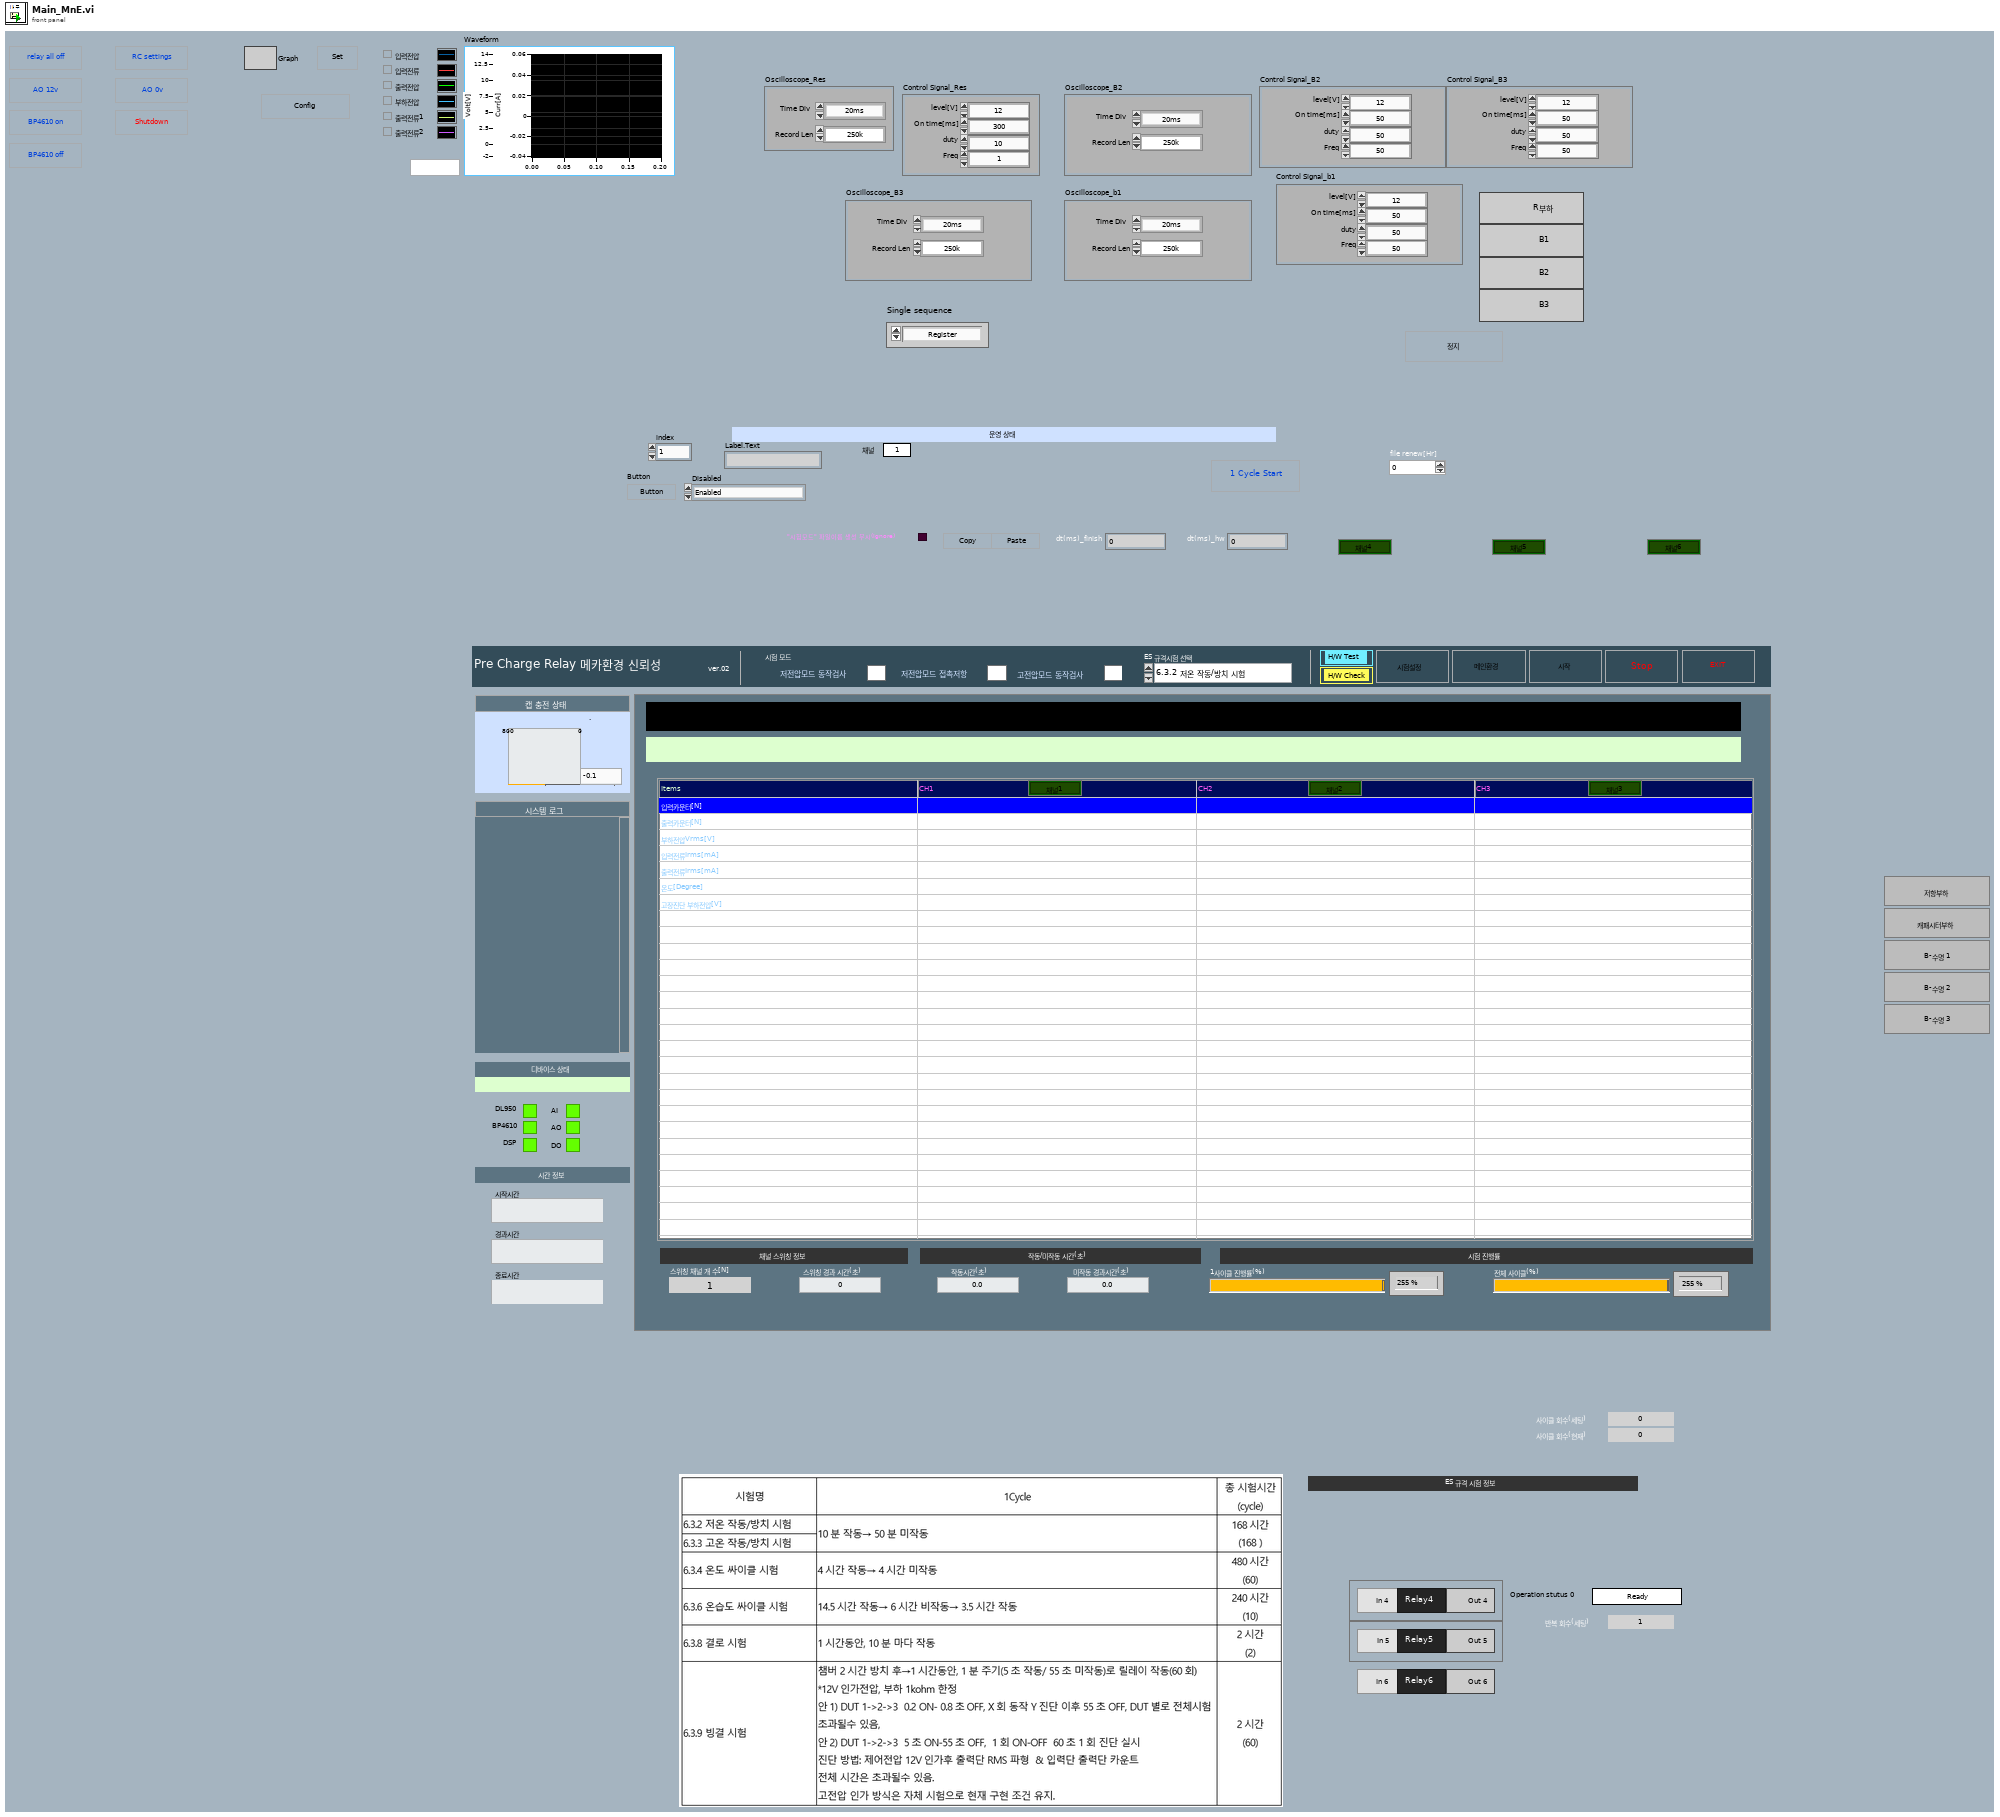
[diagram p1: front panel]
types:
  T1 = typedef "시험모드선택.ctl" = enum16{"6.3.1 온도방치 시험", "6.3.2 저온 작동/방치 시험", "6.3.3 고온 작동/방치 시험", "6.3.4 온도 싸이클 시험", "6.3.6 온습도 싸이클 시험", "6.3.7 고온고습 방치", "6.3.8 결로 시험", "6.3.9 빙결시험", "6.3.10 공진", "6.3.11.1 작동가진", "6.3.11.2 비작동 가진 ", "6.3.12 충격시험"}
  T2 = enum8{"Enabled", "Disabled", "Disabled and Grayed Out"}
  T3 = typedef "Error list.ctl" = cluster{"DL950":bool, "BP4610":bool, "DSP":bool, "AI":bool, "AO":bool, "DO":bool}
  T4 = typedef "Test Mode.ctl" = enum32{"저항부하", "캐패시터부하", "B수명 - 1", "B수명 - 2", "B수명 - 3", "저전압모드 동작검사", "저전압모드 접촉저항", "고전압모드 동작검사"}
  T5 = cluster{"Freq":dbl, "level[V]":dbl, "duty":dbl, "On time[ms]":dbl}
  T6 = typedef "sequence_single.ctl" = enum16{"Register", "RC", "B1", "B2", "B3", "Oper_LV", "Oper_HV", "ContR_LV"}
  T7 = typedef "Tap_main2.ctl" = enum32{"Manual", "Test", "Setting"}
  T8 = enum32{"System Config", "OSCILL", "INPUT", "OUTPUT", "NI AO ", "NI AI", "NI DO", "Load Config"}
  T9 = typedef "DL950_config.ctl" = cluster{"Timeout":u32, "Time Div":i32, "Acq Mode":i32, "Record Len":i32, "Record Num":i32, "Start Point":i64, "End Poin":i64, "Visa":refnum<visa-resource-name>, "Config Voltage":cluster{"Enable":bool, "Ch":u16, "V Div":i32, "Coupling":i32, "Probe":i32, "Act.Items":bool, "items":i32[]}[], "Trigger on":bool, "Trigger Level":dbl, "Reset":bool, "Config Temp":cluster{"Channel":u16, "Burn Out":bool, " Type ":i32}[], "Trig Mode":i32, "Trig Pos":dbl, "Trigger Slope":i32, "Trigger Source ":i32, "Trig Start -5":dbl, "End 5":dbl}
  T10 = cluster{"Channel":u16, "Burn Out":bool, " Type ":i32}[]
  T11 = typedef "BP4610_config.ctl" = cluster{"VISA":refnum<visa-resource-name>, "Limit-BP":cluster{"Set":enum16{"Current", "Voltage"}, "Voltage+[V]":dbl, "Current+[A]":dbl, "Voltage-[V]":dbl, "Current-[A]":dbl}, "SET BP":cluster{"Set":enum16{"Current", "Voltage", "FREQ/WAVE"}, "Operation mode":u16, "Voltage[Vp-p]":dbl, "Current[Ap-p]":dbl, "Voltage[V]":dbl, "Current[A]":dbl, "Frequency[Hz]":dbl, "Waveform":enum16{"Sine", "Square", "ARB 1", "ARB 2", "ARB 3", "ARB 4", "ARB 5", "ARB 6", "ARB 7", "ARB 8", "ARB 9", "ARB 10", "ARB 11", "ARB 12", "ARB 13", "ARB 14", "ARB 15", "ARB 16"}}}
  T12 = typedef "DSP_config.ctl" = cluster{"Port":refnum<visa-resource-name>, "OVP Level":dbl, "OCP Level":dbl, "Current":dbl, "Voltage":dbl}
  T13 = typedef "cDAQ-9269 Config.ctl" = cluster{"Ch":tag, "Max V":dbl, "Min V":dbl, " Rate":dbl, "N pts":i32, "sample mode":i32}
  T14 = typedef "Set_AO_Wave-config.ctl" = cluster{"offset":dbl, "Samples":i32, "duty":dbl, "Rate":dbl, "wfm":cluster{"Freq":dbl, "Amp":dbl, "Type":enum16{"Sine Wave", "Triangle Wave", "Square Wave", "Sawtooth Wave"}}}
  T15 = typedef "Set_NIAI.ctl" = cluster{"input terminal":i32, "minimum value":dbl, "maximum value":dbl, "number of samples":i32, "rate":dbl, "sample mode":i32, "physical channels":tag}
  T16 = enum32{"dl950", "BP4610", "DSP", "cDAQ-9221 ", "cDAQ-9467", "cDAQ-9269", "AO_Wave-config"}
  T17 = enum32{"debug", "conditions", "data gethering", "NI "}
  T18 = typedef "result.ctl" = enum16{"Init", "OK", "NG", "Shutdown", "Testing", "Completion", "Device Error", "Start", "작동", "미작동", "작동 대기", "작동 1"}
  T19 = typedef "cap_config.ctl" = cluster{"Test Mode":T1, "ON time[ms]":dbl, "OFF time[ms]":dbl, "1. 작동시간[분]":dbl, "2. 미작동시간[분]":dbl, "3. 작동시간[분]":dbl, "level[V]":dbl, "duty":dbl, "Freq":dbl, "Voltage+[V]":dbl, "Voltage-[V]":dbl, "Current+[A]":dbl, "Current-[A]":dbl, "출력전압[V]":dbl, "출력전류[A]":dbl, "OVP Level":dbl, "OCP Level":dbl, "Time Div":u16, "Record Len":i32, "방전 기준[V]":dbl, "Repeate (Each Ch)":u32, "Cycle[N]":u32, "작동간격[분]":dbl, "TrigPos[%]":dbl, "시험시간[분]":dbl}
  T20 = typedef "measure_reg.ctl" = cluster{"입력카운트":dbl, "출력카운트":dbl, "부하전압 RMS":dbl, "입력전류 RMS":dbl, "출력전류 RMS":dbl, "온도":dbl, "부하전압(고장)":dbl}
  T21 = typedef "measure_rc.ctl" = cluster{"입력카운트":dbl, "출력카운트":dbl, "Rising Time 63%":dbl, "Rising Time 98%":dbl, "Failing Time 37%":dbl, "입력전류 RMS":dbl, "출력전류 RMS":dbl, "출력전압 + 평균 63%":dbl, "출력전압 - 평균 63%":dbl, "출력전류 평균 63%":dbl, "접촉저항":dbl, "온도":dbl, "방전전압":dbl, "부하전압(고장)":dbl, "충전전압 63초":dbl, "충전전압 98초":dbl, "충전전류 37초":dbl, "전압강하":dbl}
  T22 = typedef "data_contR.ctl" = cluster{"입력카운트":dbl, "출력카운트":dbl, "입력전류 RMS":dbl, "출력전류 RMS":dbl, "출력전압(+)_Avg":dbl, "출력전압(-)_Avg":dbl, "출력전류_Avg":dbl, "접촉저항":dbl, "온도":dbl, "부하전압":dbl}
  T23 = typedef "error_rc.ctl" = cluster{"제어단 단선":bool, "제어단 단락":bool, "제어단 특성변화":bool, "출력단 단선":bool, "출력단 단락":bool, "출력단 특성변화":bool, "출력전압":bool, "카운트 일치":bool, "전압 98%":bool, "전압 63%":bool, "전류 37%":bool, "방전전압":bool, "온도":bool}
  T24 = typedef "Breakdown-Spec.ctl" = cluster{"제어단 단선 Irms[mA](이하)":dbl, "제어단 특성 전류 Irms[mA] Max":dbl, "제어단 특성 전류 Irms[mA] Min":dbl, "출력단 단선 Irms[mA](이하)":dbl, "출력단 특성 전류 Irms[mA]  Max":dbl, "출력단 특성전류 Irms[mA]  Min":dbl, "온도[degree]":dbl}
  T25 = typedef "Judge_RC.ctl" = cluster{"전압 63%[mS] Min":dbl, "전압 98%[mS] Min":dbl, "전류 37%[mS] Min":dbl, "접촉저항[mOhm] Min":dbl, "출력전류 Irms[mA] Min":dbl, "전압 63%[mS] Max":dbl, "전압 98%[mS] Max":dbl, "전류 37%[mS] Max":dbl, "접촉저항[mOhm] Max":dbl, "출력전류 Irms[mA] Max":dbl}
  T26 = cluster{"Ch 1":bool, "Ch 2":bool, "Ch 3":bool, "Ch 4":bool, "Ch 5":bool, "Ch 6":bool}
  T27 = typedef "create-rw-close.ctl" = enum16{"create", "write", "read", "delete", "close"}
  T28 = enum16{"yellow", "red", "green", "buzz1", "buzz2"}
  T29 = typedef "init-r-stop.ctl" = enum16{"ini", "read", "stop"}
  T30 = typedef "cmd_tablecnt.ctl" = enum16{"Create", "Inital", "Write", "Default"}
  T31 = typedef "cmd_ch act.ctl" = enum16{"open", "initial", "update"}
  T32 = typedef "def_chact.ctl" = cluster{"ch 1":refnum<vi>, "ch 2":refnum<vi>, "ch 3":refnum<vi>, "ch 4":refnum<vi>, "ch 5":refnum<vi>, "ch 6":refnum<vi>}
  T33 = typedef "ref_all.ctl" = cluster{"BP4610 Config":refnum<vi>, "DSP1950 Config":refnum<vi>, "2470-config":refnum<vi>, "cDAQ 9269 AO config":refnum<vi>, "cDAQ 9221 Config":refnum<vi>, "cDAQ-9467 Config":refnum<vi>, "Waveform":refnum<vi>, "DL950 wfm":refnum<vi>, "AI Graph":refnum<vi>, "AO_Wave-config":refnum<vi>, "DL950 items":refnum<vi>, "Volt":refnum<vi>, "Current":refnum<vi>, "AO_Level":refnum<vi>, "RC-Test Judgement ":refnum<vi>, "Log path":refnum<vi>, "시험명":refnum<vi>, "file renew[Hr]":refnum<vi>, "Breakdown-Spec":refnum<vi>, "paste":refnum<vi>, "copy":refnum<vi>, "DL950_config":refnum<vi>, "종료시간":refnum<vi>, "경과시간":refnum<vi>, "Apply":refnum<vi>, "DSP Config LV ":refnum<vi>, "Testconfig":refnum<vi>}
  T34 = typedef "rw.ctl" = enum16{"read", "write"}
  T35 = typedef "ref.ctl" = cluster{"relay 1":refnum<vi>, "relay 2":refnum<vi>, "relay 3":refnum<vi>, "relay 4":refnum<vi>, "relay 5":refnum<vi>, "relay 6":refnum<vi>, "PoutR 1":refnum<vi>, "PoutR 2":refnum<vi>, "PoutR 3":refnum<vi>, "PoutR 4":refnum<vi>, "PoutR 5":refnum<vi>, "PoutR 6":refnum<vi>, "Discharge":refnum<vi>, "Input Pwr":refnum<vi>, "Output_HV":refnum<vi>, "AO onoff":refnum<vi>}
  T36 = typedef "ui_dev-operator.ctl" = cluster{"Operation stutus":refnum<vi>, "Test Status":refnum<vi>, "Setting":refnum<vi>, "Manual":refnum<vi>, "Main":refnum<vi>, "RCstart":refnum<vi>, "채널선택":refnum<vi>, "시험명":refnum<vi>, "Tab Control_manual":refnum<vi>, "시험 모드":refnum<vi>, "HW check":refnum<vi>, "login":refnum<vi>, "logout":refnum<vi>}
  T37 = enum16{"Config Save", "Config Load", "LastRUN Save", "LastRUN Load"}
  T38 = typedef "system-status.ctl" = enum16{"Initial", "Update", "Clear", "Read"}
  T39 = typedef "init-r-w.ctl" = enum16{"init", "read", "write"}
  T40 = typedef "cmd_TestParaSave.ctl" = enum16{"Save", "Read", "Idle"}
  T41 = typedef "infor_testcycle.ctl" = cluster{"Channel selection":cluster{"1ch":bool, "2ch":bool, "3ch":bool, "4ch":bool, "5ch":bool, "6ch":bool}, "Test Cycle":u32, "Repeate":u32}
  T42 = typedef "cmd_logInfor.ctl" = enum16{"ADMIN", "OPER", "DEFAULT"}
  T43 = typedef "UI dev-operator.ctl" = enum16{"Testing", "Admin", "Operator", "Finish", "Ready"}
  T44 = typedef "start.ctl" = enum16{"init", "open", "set", "start", "stop", "read", "read_items", "query", "close", "T_single", "reset", "exit"}
  T45 = typedef "DSP_action.ctl" = enum16{"False", "cont", "on", "off", "discont", "protection", "protection_seq", "preread", "level_seq", "level_m", "read", "stop", "exit"}
  T46 = typedef "BP4610_cmd.ctl" = enum16{"open", "read", "set", "set_seq", "limit", "limit_seq", "output on", "output off", "close"}
  T47 = typedef "init-w-close.ctl" = enum16{"open", "init", "write", "close"}
  T48 = typedef "cnt_do.ctl" = enum16{"open", "initial", "update", "run", "close"}
  T49 = typedef "cnt_Relay.ctl" = enum32{"R_Load", "R_out1", "R_out2", "R_out3", "R_out4", "R_out5", "R_out6", "R8", "R9", "R10", "R11", "R12", "R13", "R14", "R15", "R16", "R_in1", "R_in2", "R_in3", "R_in4", "R_in5", "R_in6", "R23", "R24", "R25", "R26", "R27", "R_red", "R_yellow", "R_green", "R_buz", "R_purple"}
  T50 = typedef "hw-control.ctl" = enum16{"DL950 ready", "DL950 clear", "DL950 trigger", "DL950 read", "DL950 read seq", "DL950 Tsingle query", "AO 12v", "AO wave", "AO 0v", "relay all-off", "Discharge check", "Discharge", "Relay1", "Relay2", "Relay3", "Relay4", "Relay5", "Relay6", "BP4610 onoff", "BP4610 set", "DSP1500 set", "DSP1500 onoff"}
  T51 = typedef "hwsetting.ctl" = enum16{"BP4610 RC", "DSP1500 RC", "AO"}
  T52 = typedef "cmd_timer.ctl" = enum16{"init", "init_update", "run", "default", "update"}
  T53 = enum32{"6.3.2 저온 작동/방치 시험", "6.3.3 고온 작동/방치 시험", "6.3.4 온도 싸이클 시험", "6.3.6 온습도 싸이클 시험", "6.3.8 결로 시험", "6.3.9 빙결 시험"}
  T54 = typedef "fgv_DL950.ctl" = enum16{"init", "config", "Set-NCh", "setapply", "trigger", "history_clear", "read", "time-div", "wave-aquis", "start", "query", "abort", "set_items", "reset_items", "read_items", "percent_rise", "trigger_single", "stop", "offset cancel", "close"}
  T55 = typedef "log save type.ctl" = enum16{"header", "data"}
  T56 = typedef "type_signal.ctl" = enum16{"wave", "level"}
  T57 = typedef "fgv_Main_q.ctl" = enum16{"init", "wait", "R", "RC", "RC_M", "B1", "B2", "B3", "exit"}
  T58 = enum32{"Invalid", "Standard", "Closed", "Hidden", "Minimized", "Maximized"}
  T59 = typedef "Tpye_ParaAll.ctl" = cluster{"DL950_config":T9, "BP4610 Config":T11, "DSP1950 Config":T12, "DMM 2470 Config":cluster{"Source Mode":enum16{"Voltage", "Current"}, "Source Limit Level":dbl, "Source Level":dbl, "Output_2470":bool}, "cDAQ-9221 Config":T15, "cDAQ-9467 Config":tag, "cDAQ-9269 AO Config":T13, "AO_Wave-config":T14, "DSP1950 Config LV":T12}
  T60 = typedef "config_aging.ctl" = cluster{"Setting":T61, "TestName":string, "Result path":path, "파일 생성 주기[N]":u8, "Test Specs":T24}
  T61 = typedef "Setting_reg.ctl" = cluster{"제어 전압[V]":dbl, "출력전압[V]":dbl, "전류[A]":dbl, "출력전류[A]":dbl, "ON[초]":dbl, "OFF[초]":dbl, "Irms 허용치 from ":dbl, "Irms 허용치 to":dbl, "AO Delay ms":u32, "Log":path, "result":path}
  T62 = typedef "Testing-info.ctl" = cluster{"전체채널수":u8, "현재채널번호":u8, "Irms":dbl, "입력전압":dbl, "입력전류":dbl, "출력전압":dbl, "출력전류":dbl, "온도":dbl, "제어단 단선":bool, "제어단 단락":bool, "제어단 특성변화":bool, "출력단 단선":bool, "출력단 단락":bool, "출력단 특성변화":bool, "출력단 전압":bool, "카운트 일치":bool, "Irms 판정":bool, "온도":bool, "테스트 회수":u32, "TestType":T6, "현재회수":u32, "Ch selection":cluster{"1ch":bool, "2ch":bool, "3ch":bool, "4ch":bool, "5ch":bool, "6ch":bool}, "반복":u32, "Path":path, "파일생성주기":u32, "start time":dbl, "stop time":dbl, "현재반복회수":u32, "NG":cluster{"입출력 카운트":bool, "출력전류RMS":bool}}
  T63 = cluster{"1ch":bool, "2ch":bool, "3ch":bool, "4ch":bool, "5ch":bool, "6ch":bool}
  T64 = enum32{"Bad", "Idle", "Run top level", "Running"}
  T65 = typedef "DL950_wfms.ctl" = cluster{"wfms":waveform(dbl)[], "Waveform_2":cluster{"t0":dbl, "dt":dbl, "Y":dbl[][]}, "items":dbl[][], "da950_array":dbl[]}
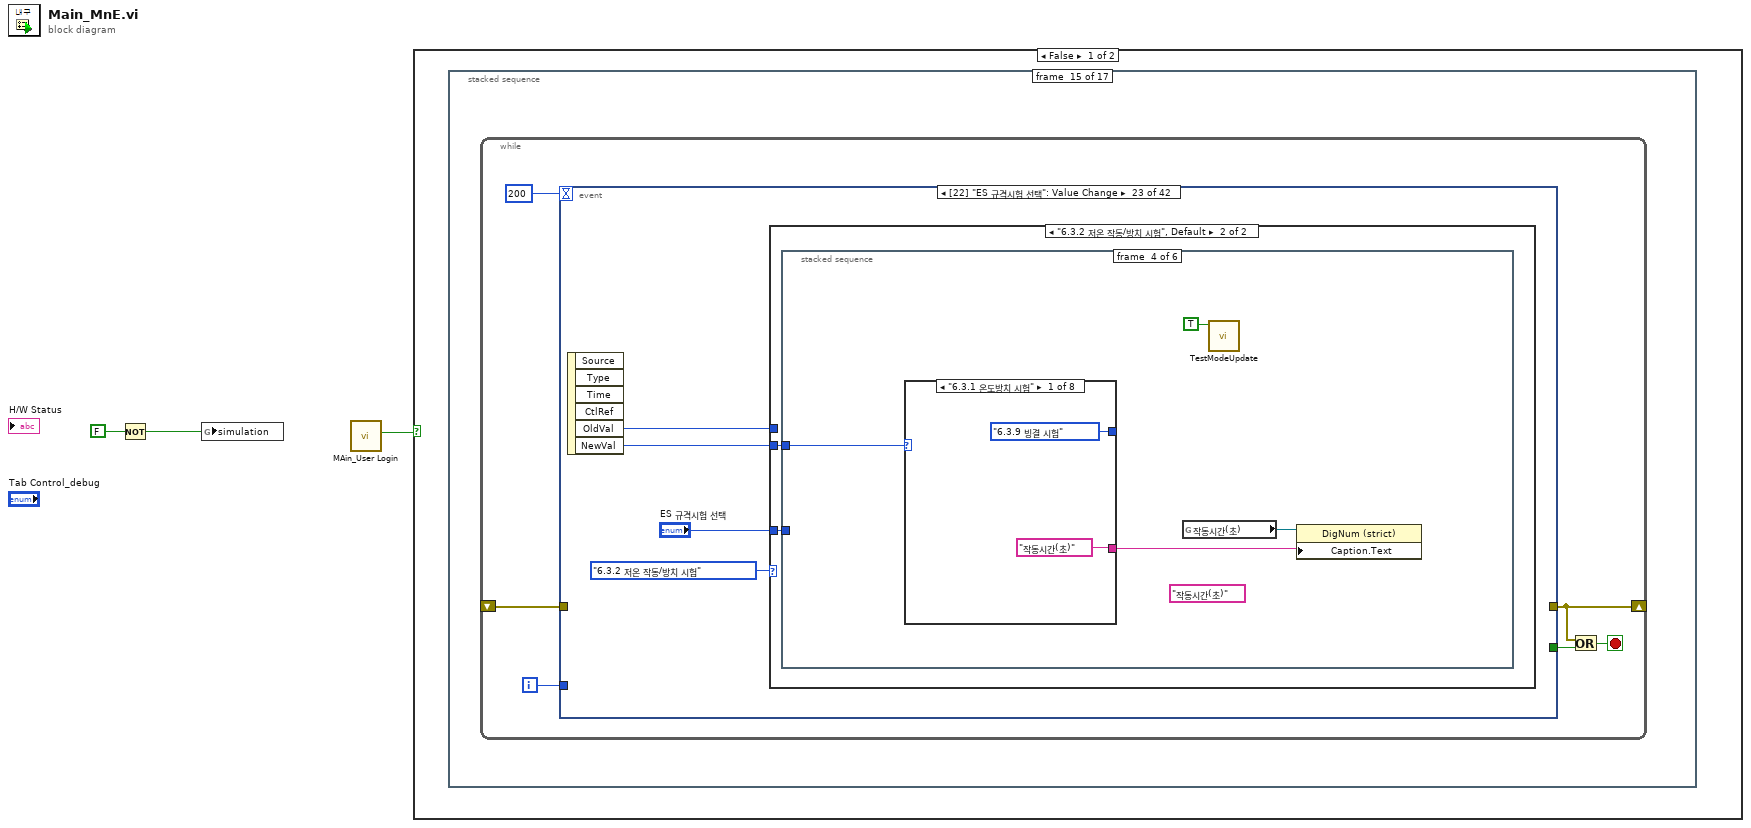
[diagram p0: block diagram]
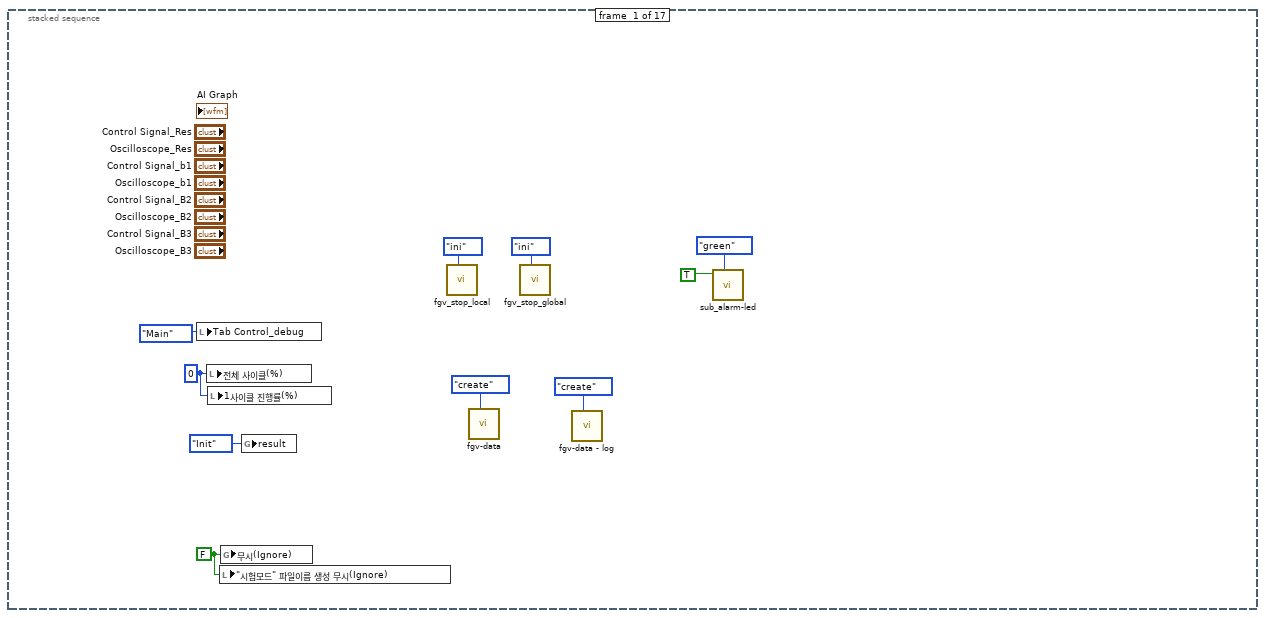
[diagram p2: hidden frame]
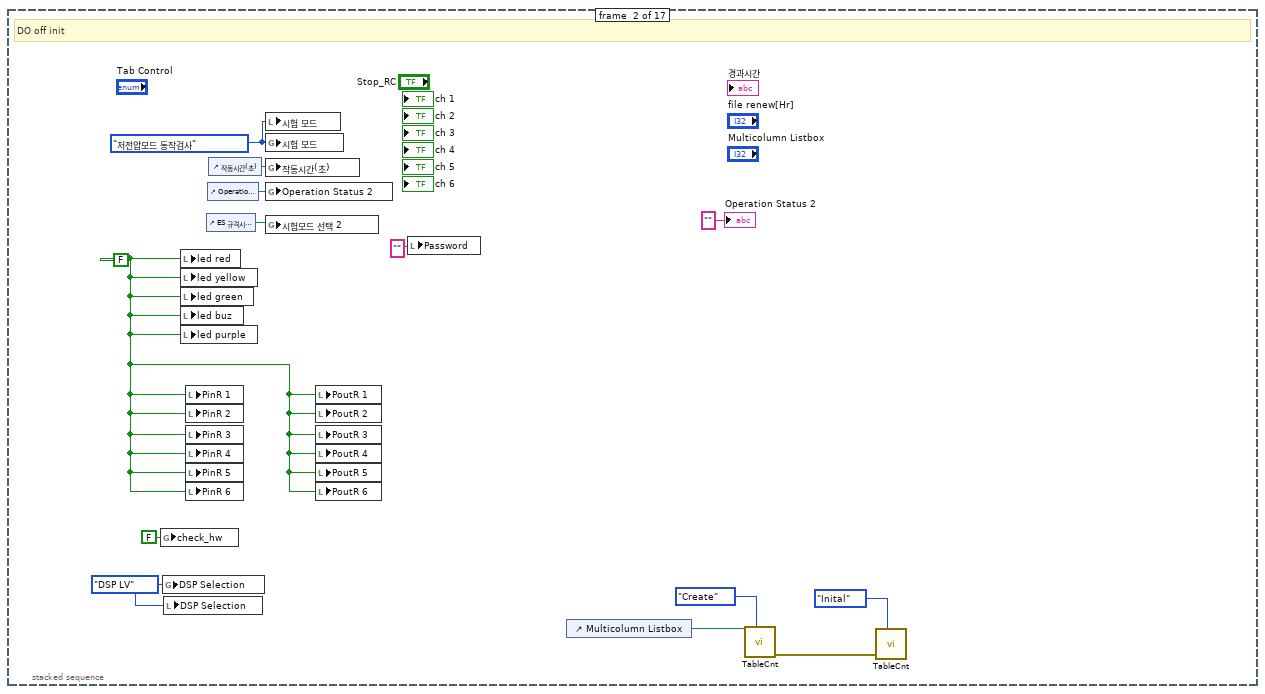
[diagram p3: hidden frame]
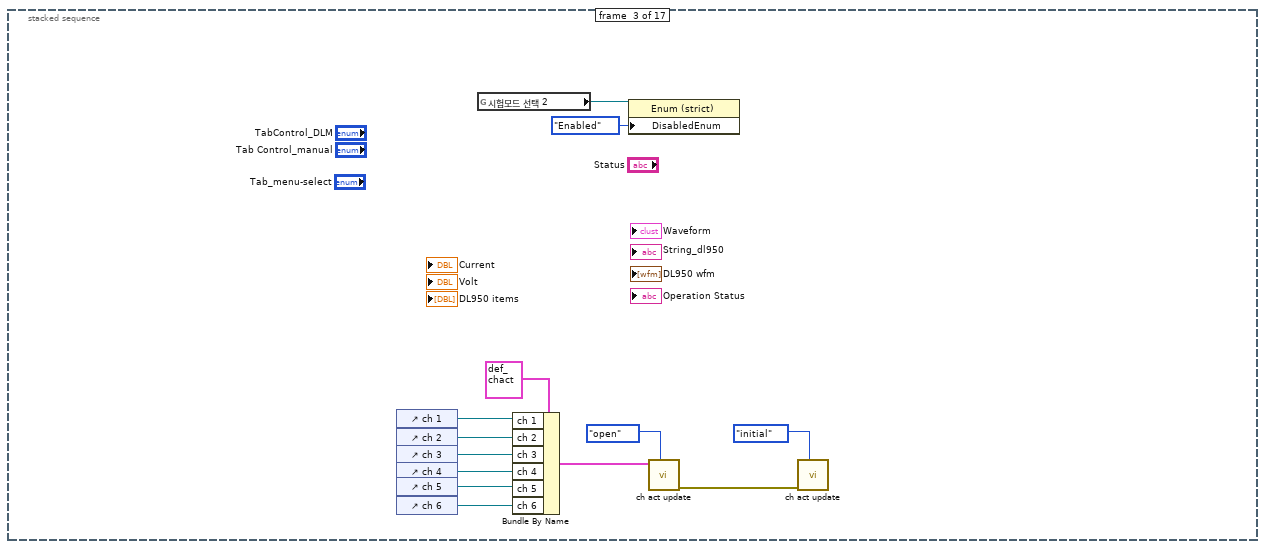
[diagram p4: hidden frame]
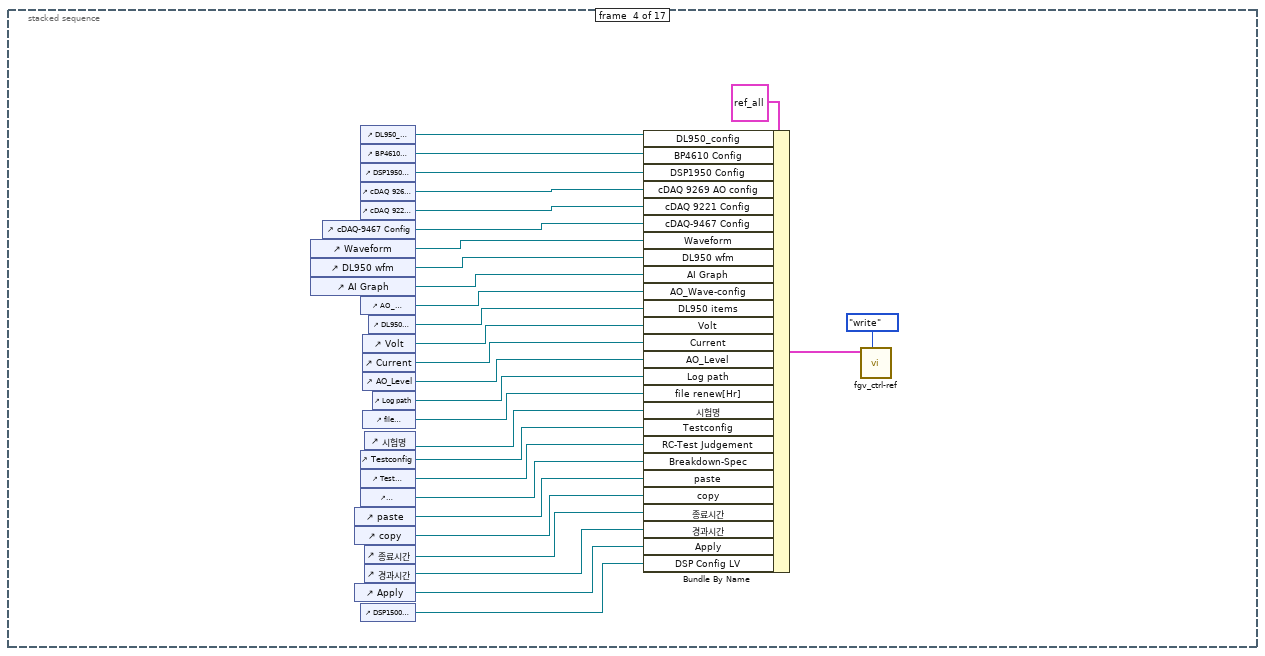
[diagram p5: hidden frame]
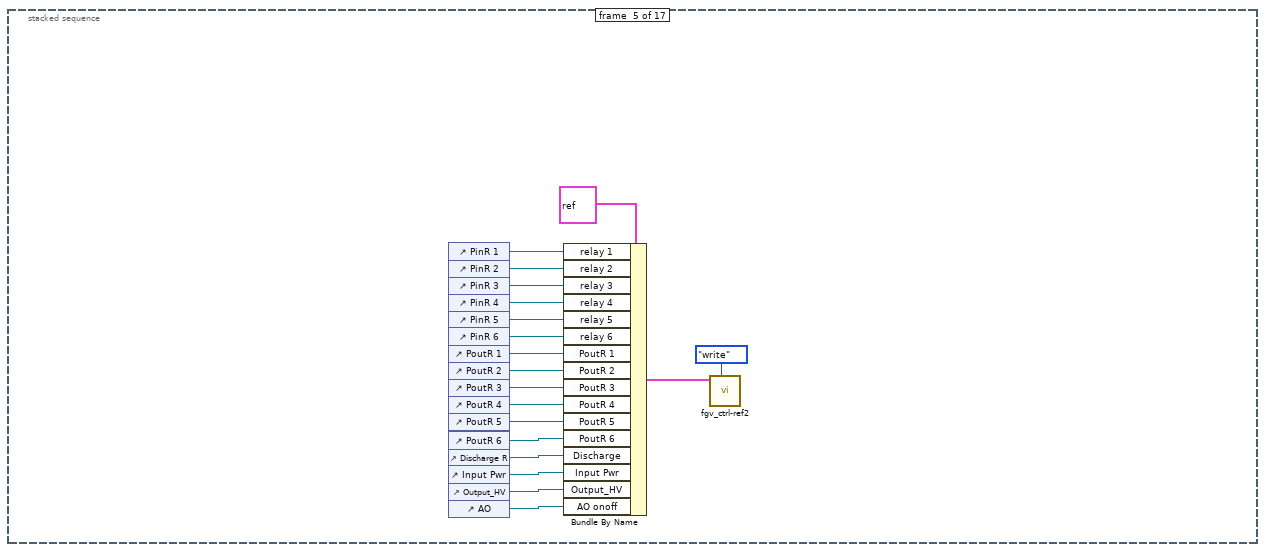
[diagram p6: hidden frame]
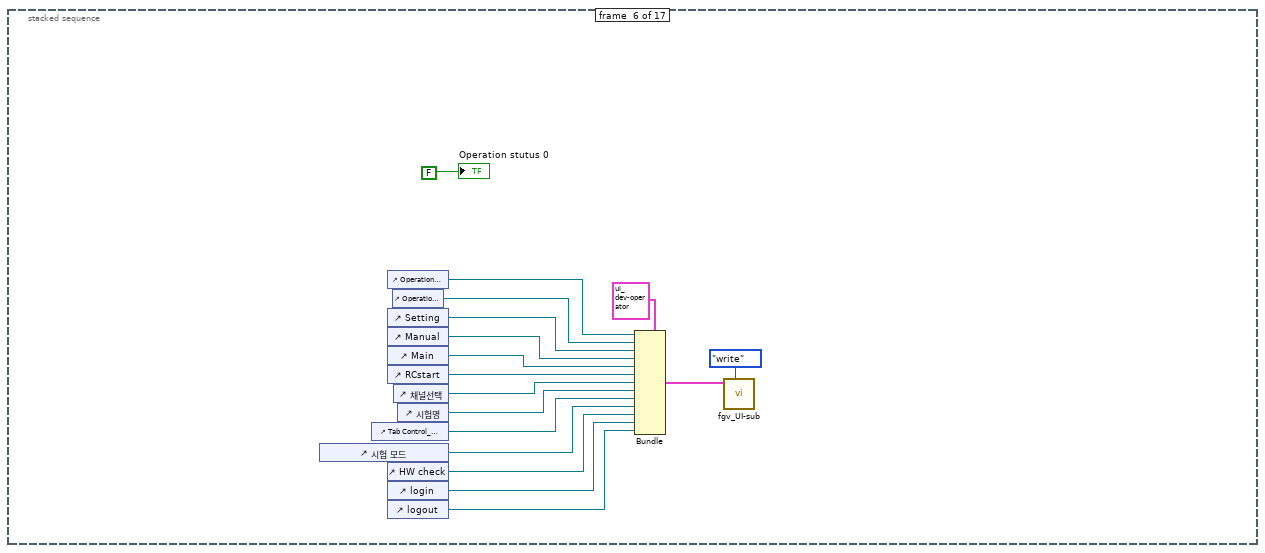
[diagram p7: hidden frame]
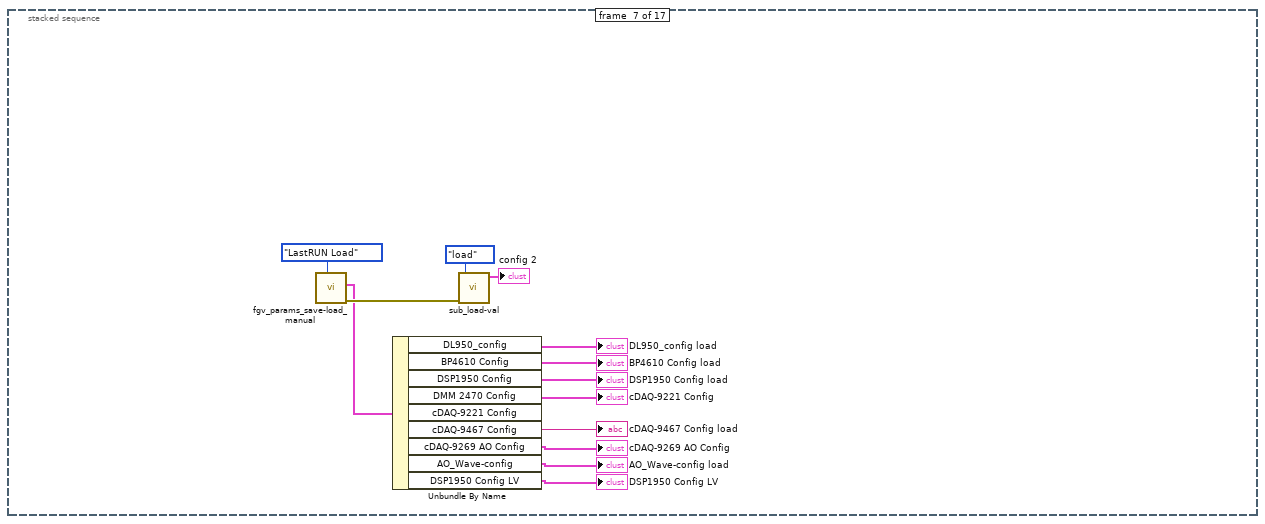
[diagram p8: hidden frame]
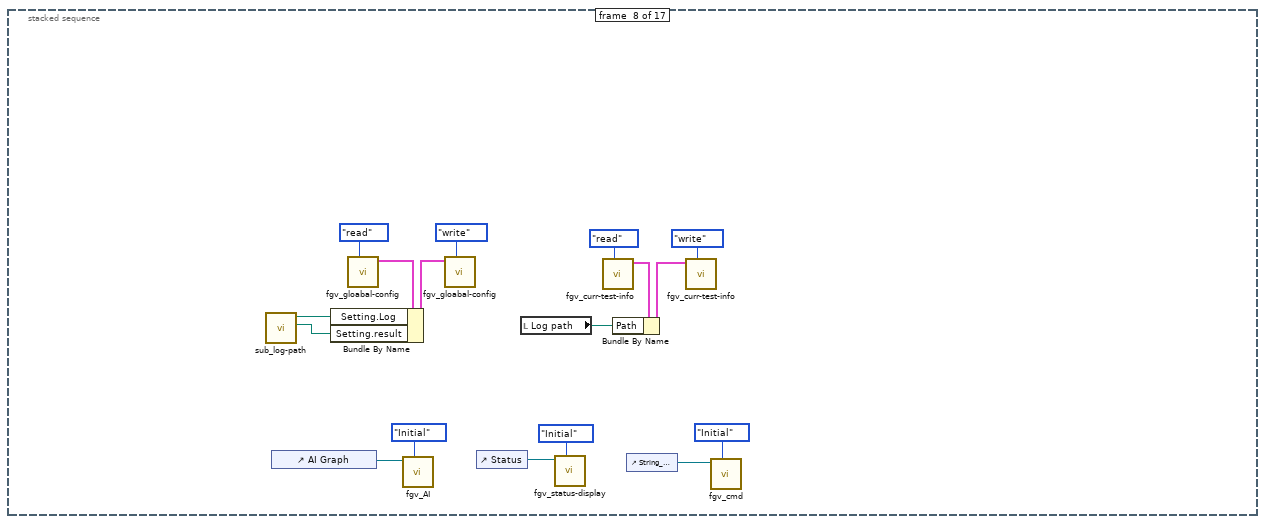
[diagram p9: hidden frame]
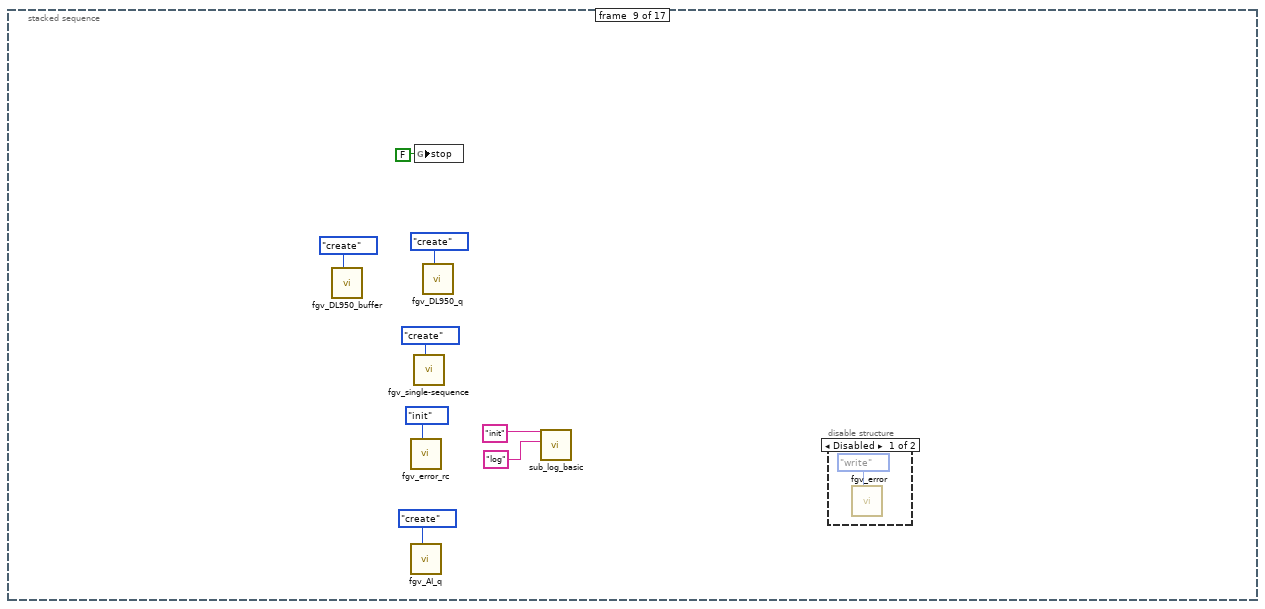
[diagram p10: hidden frame]
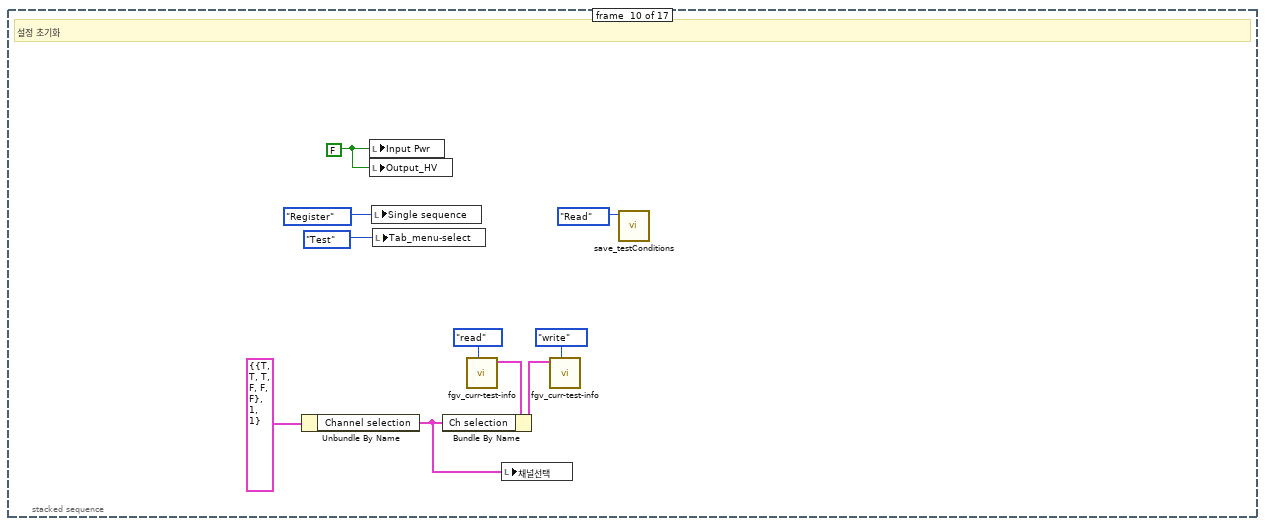
[diagram p12: hidden frame]
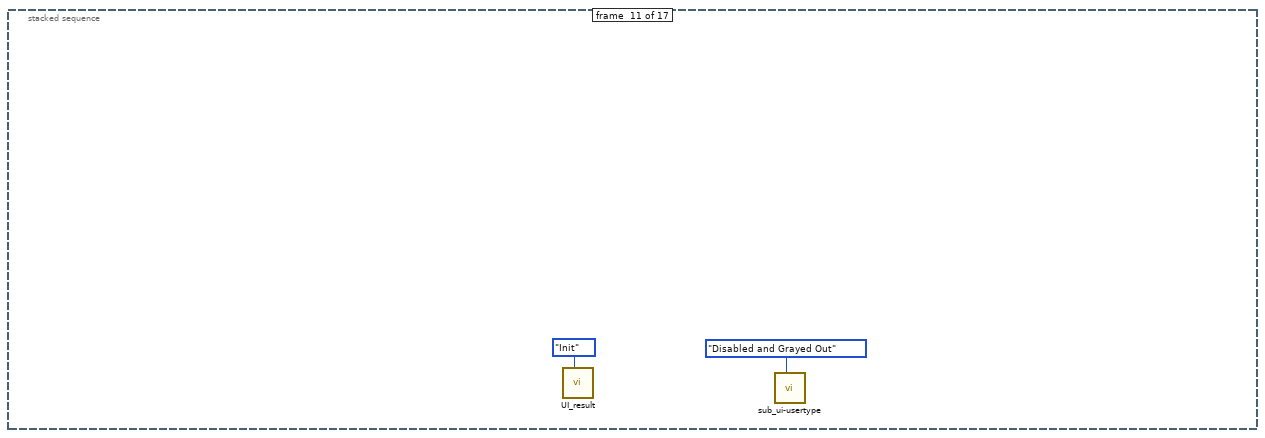
[diagram p13: hidden frame]
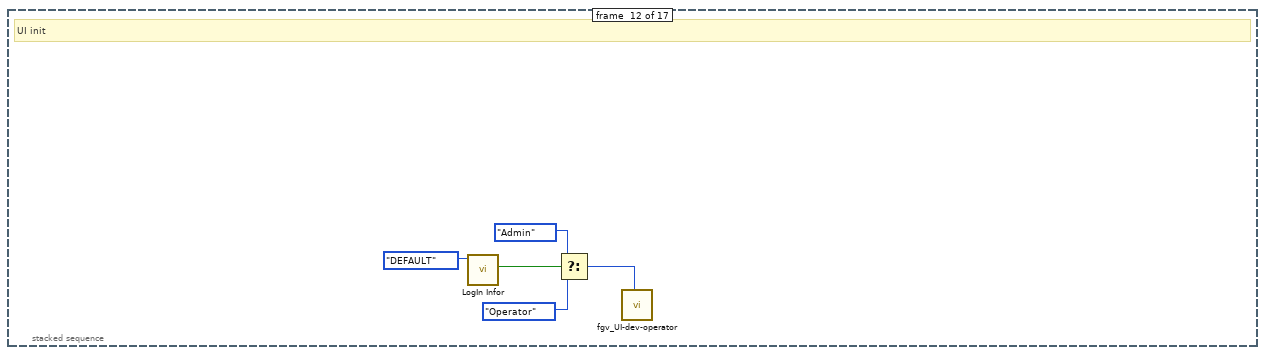
[diagram p14: hidden frame]
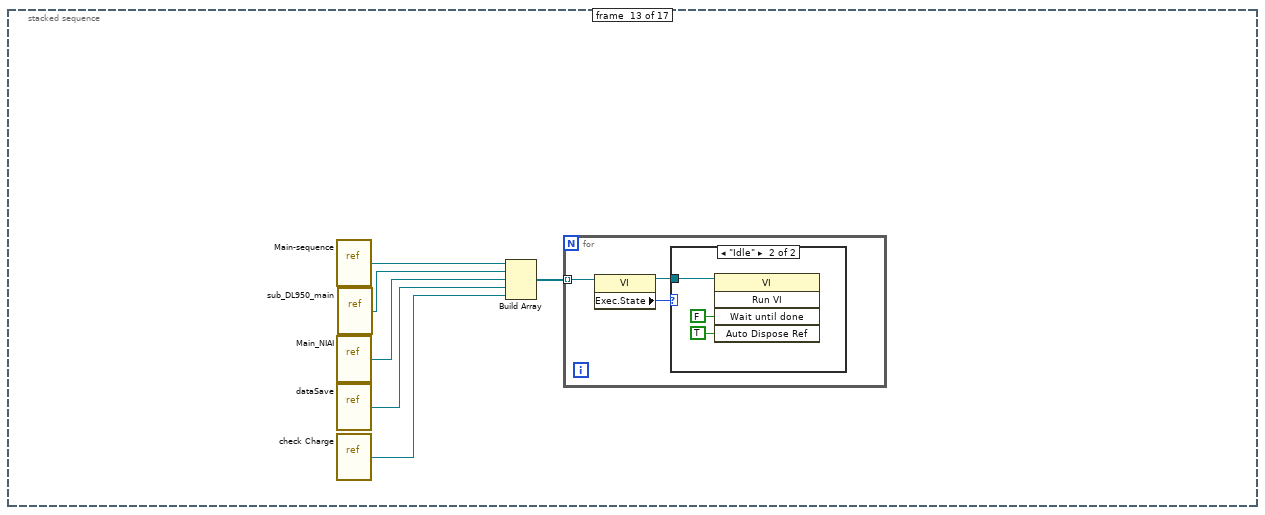
[diagram p15: hidden frame]
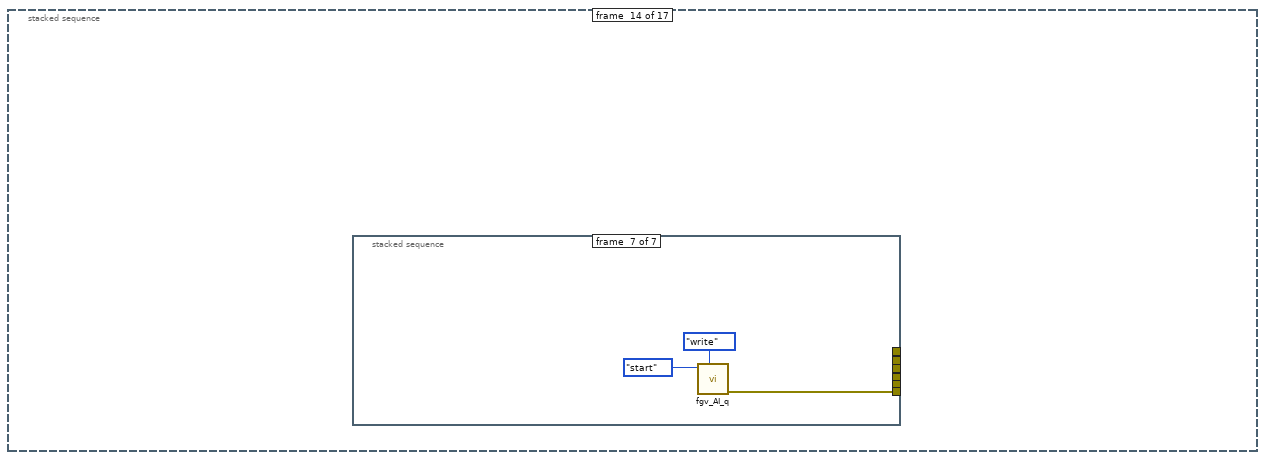
[diagram p17: hidden frame]
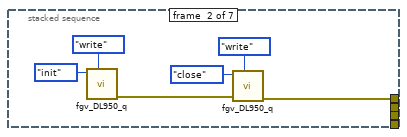
[diagram p19: hidden frame]
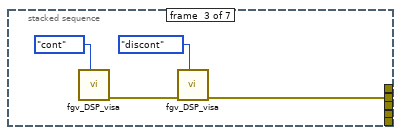
[diagram p20: hidden frame]
diagram:
  n1 = Not(x=FALSE ("simulation")) -> (.not. x?=w1:bool)
  n2 = global write "Glob_Ref.vi" "simulation"(w1) -> ()
  n3 = call "MAin_User Login.vi"() -> ("취소"=w3:bool)  [unwired: 7 in, 3 out]
  n4 = case shown="False" w3 {
    frame False {
      n5 = stacked-sequence {
        frame #0 {
          w4 = FALSE ("무시(Ignore)")
          w6 = u8 0 ("전체 사이클(%)")
          n6 = local write "Tab Control_debug"(enum32{"Main", "debug"}."Main" ("Tab Control_debug")) -> ()
          n7 = local write "전체 사이클(%)"(w6) -> ()
          n8 = local write "1사이클 진행률(%)"(w6) -> ()
          n9 = local write "\"시험모드\" 파일이름 생성 무시(Ignore)"(w4) -> ()
          n10 = global write "Glob_setting.vi" "무시(Ignore)"(w4) -> ()
          n11 = global write "Glob_setting.vi" "result"(result."Init" ("result")) -> ()
          n12 = call "fgv_stop_local.vi"("cmd"=init-r-stop."ini") -> ()  [unwired: 9 in, 2 out]
          n13 = call "fgv-data.vi"("cmd"=create-rw-close."create") -> ()  [unwired: 9 in, 2 out]
          n14 = call "fgv_stop_global.vi"("cmd"=init-r-stop."ini") -> ()  [unwired: 10 in, 1 out]
          n15 = call "fgv-data - log.vi"("cmd"=create-rw-close."create") -> ()  [unwired: 9 in, 2 out]
          n16 = call "sub_alarm-led.vi"("alarm"=T28."green", "onoff"=TRUE) -> ()  [unwired: 9 in, 1 out]
        }
        frame #1 {
          w18 = enum32{"DSP HV", "DSP LV"}."DSP LV" ("DSP Selection")
          w19 = Test_Mode."저전압모드 동작검사" ("시험 모드")
          w26 = FALSE ("led red")
          # "DO off init"
          n17 = global write "Glob_Ref.vi" "check_hw"(FALSE ("check_hw")) -> ()
          n18 = global write "Glob_Ref.vi" "DSP Selection"(w18) -> ()
          n19 = local write "DSP Selection"(w18) -> ()
          n20 = local write "led red"(w26) -> ()
          n21 = local write "led yellow"(w26) -> ()
          n22 = local write "led green"(w26) -> ()
          n23 = local write "led buz"(w26) -> ()
          n24 = local write "led purple"(w26) -> ()
          n25 = local write "PinR 1"(w26) -> ()
          n26 = local write "PinR 2"(w26) -> ()
          n27 = local write "PinR 3"(w26) -> ()
          n28 = local write "PinR 4"(w26) -> ()
          n29 = local write "PinR 5"(w26) -> ()
          n30 = local write "PinR 6"(w26) -> ()
          n31 = control-ref of="ES 규격시험 선택"() -> (w14:refnum<vi>)
          n32 = control-ref of="Operation Status 2"() -> (w16:refnum<vi>)
          n33 = control-ref of="작동시간(초)"() -> (w17:refnum<vi>)
          n34 = local write "시험 모드"(w19) -> ()
          n35 = global write "Global 1.vi" "시험 모드"(w19) -> ()
          n36 = global write "Global 1.vi" "작동시간(초)"(w17) -> ()
          n37 = global write "Global 1.vi" "Operation Status 2"(w16) -> ()
          n38 = global write "Global 1.vi" "시험모드 선택 2"(w14) -> ()
          n39 = local write "PoutR 1"(w26) -> ()
          n40 = local write "PoutR 2"(w26) -> ()
          n41 = local write "PoutR 3"(w26) -> ()
          n42 = local write "PoutR 4"(w26) -> ()
          n43 = local write "PoutR 5"(w26) -> ()
          n44 = local write "PoutR 6"(w26) -> ()
          n45 = local write "Password"("" ("PW")) -> ()
          n46 = control-ref of="Multicolumn Listbox"() -> (w24:refnum<vi>)
          n47 = call "TableCnt.vi"("cnt"=cmd_tablecnt."Create", "table_result"=w24) -> ("error out"=w22:errorcluster)  [unwired: 8 in, 1 out]
          n48 = call "TableCnt.vi"("cnt"=cmd_tablecnt."Inital", "error in"=w22) -> ()  [unwired: 8 in, 2 out]
          "Operation Status 2" <- "" ("Operation Status 2")
        }
        frame #2 {
          n49 = control-ref of="ch 1"() -> (w37:refnum<vi>)
          n50 = control-ref of="ch 2"() -> (w36:refnum<vi>)
          n51 = control-ref of="ch 3"() -> (w32:refnum<vi>)
          n52 = control-ref of="ch 4"() -> (w31:refnum<vi>)
          n53 = control-ref of="ch 5"() -> (w30:refnum<vi>)
          n54 = control-ref of="ch 6"() -> (w29:refnum<vi>)
          n55 = global read "Global 1.vi" "시험모드 선택 2"() -> (w28:refnum<vi>)
          n56 = Bundle By Name(cluster=T32 {"ch 1"=refnum, "ch 2"=refnum, "ch 3"=refnum, "ch 4"=refnum, "ch 5"=refnum, "ch 6"=refnum} ("Cluster"), "ch 1"=w37, "ch 2"=w36, "ch 3"=w32, "ch 4"=w31, "ch 5"=w30, "ch 6"=w29) -> (w35:T32)
          n57 = property class="Enum (strict)"(reference=w28, "DisabledEnum"=T2."Enabled" ("Disabled")) -> ()  [unwired: 1 in, 2 out]
          n58 = call "ch act update.vi"("cmd"=cmd_ch_act."open", "Cluster"=w35) -> ("error out"=w33:errorcluster)  [unwired: 9 in]
          n59 = call "ch act update.vi"("cmd"=cmd_ch_act."initial", "error in (no error)"=w33) -> ()  [unwired: 9 in, 1 out]
        }
        frame #3 {
          n60 = control-ref of="Waveform"() -> (w62:refnum<vi>)
          n61 = control-ref of="DL950 wfm"() -> (w61:refnum<vi>)
          n62 = control-ref of="AI Graph"() -> (w60:refnum<vi>)
          n63 = control-ref of="cDAQ-9467 Config"() -> (w63:refnum<vi>)
          n64 = control-ref of="paste"() -> (w47:refnum<vi>)
          n65 = control-ref of="copy"() -> (w46:refnum<vi>)
          n66 = control-ref of="Apply"() -> (w42:refnum<vi>)
          n67 = control-ref of="DL950_config"() -> (w45:refnum<vi>)
          n68 = control-ref of="BP4610 Config"() -> (w67:refnum<vi>)
          n69 = control-ref of="DSP1950 Config"() -> (w66:refnum<vi>)
          n70 = control-ref of="cDAQ 9269 AO config"() -> (w65:refnum<vi>)
          n71 = control-ref of="cDAQ 9221 Config"() -> (w64:refnum<vi>)
          n72 = control-ref of="AO_Wave-config"() -> (w59:refnum<vi>)
          n73 = control-ref of="Testconfig"() -> (w40:refnum<vi>)
          n74 = control-ref of="Test Judgement"() -> (w49:refnum<vi>)
          n75 = control-ref of="Breakdown-Spec"() -> (w48:refnum<vi>)
          n76 = control-ref of="DSP1500 Config LV"() -> (w41:refnum<vi>)
          n77 = control-ref of="Volt"() -> (w57:refnum<vi>)
          n78 = control-ref of="Current"() -> (w56:refnum<vi>)
          n79 = control-ref of="AO_Level"() -> (w55:refnum<vi>)
          n80 = control-ref of="file renew[Hr]"() -> (w51:refnum<vi>)
          n81 = control-ref of="시험명"() -> (w50:refnum<vi>)
          n82 = control-ref of="종료시간"() -> (w44:refnum<vi>)
          n83 = control-ref of="경과시간"() -> (w43:refnum<vi>)
          n84 = control-ref of="DL950 items"() -> (w58:refnum<vi>)
          n85 = control-ref of="Log path"() -> (w52:refnum<vi>)
          n86 = Bundle By Name(cluster=T33 {"BP4610 Config"=refnum, "DSP1950 Config"=refnum, "2470-config"=refnum, "cDAQ 9269 AO config"=refnum, "cDAQ 9221 Config"=refnum, "cDAQ-9467 Config"=refnum, "Waveform"=refnum, "DL950 wfm"=refnum, "AI Graph"=refnum, "AO_Wave-config"=refnum, "DL950 items"=refnum, "Volt"=refnum, "Current"=refnum, "AO_Level"=refnum, "RC-Test Judgement "=refnum, "Log path"=refnum, "시험명"=refnum, "file renew[Hr]"=refnum, "Breakdown-Spec"=refnum, "paste"=refnum, "copy"=refnum, "DL950_config"=refnum, "종료시간"=refnum, "경과시간"=refnum, "Apply"=refnum, "DSP Config LV "=refnum, "Testconfig"=refnum} ("output cluster"), "DL950_config"=w45, "BP4610 Config"=w67, "DSP1950 Config"=w66, "cDAQ 9269 AO config"=w65, "cDAQ 9221 Config"=w64, "cDAQ-9467 Config"=w63, "Waveform"=w62, "DL950 wfm"=w61, "AI Graph"=w60, "AO_Wave-config"=w59, "DL950 items"=w58, "Volt"=w57, "Current"=w56, "AO_Level"=w55, "Log path"=w52, "file renew[Hr]"=w51, "시험명"=w50, "Testconfig"=w40, "RC-Test Judgement"=w49, "Breakdown-Spec"=w48, "paste"=w47, "copy"=w46, "종료시간"=w44, "경과시간"=w43, "Apply"=w42, "DSP Config LV"=w41) -> (w53:T33)
          n87 = call "fgv_ctrl-ref.vi"("cmd"=rw."write", "output cluster"=w53) -> ()  [unwired: 8 in, 2 out]
        }
        frame #4 {
          n88 = control-ref of="PinR 1"() -> (w86:refnum<vi>)
          n89 = control-ref of="PinR 2"() -> (w85:refnum<vi>)
          n90 = control-ref of="PinR 3"() -> (w83:refnum<vi>)
          n91 = control-ref of="PinR 4"() -> (w82:refnum<vi>)
          n92 = control-ref of="PinR 5"() -> (w81:refnum<vi>)
          n93 = control-ref of="PinR 6"() -> (w80:refnum<vi>)
          n94 = control-ref of="PoutR 1"() -> (w79:refnum<vi>)
          n95 = control-ref of="PoutR 2"() -> (w78:refnum<vi>)
          n96 = control-ref of="PoutR 3"() -> (w77:refnum<vi>)
          n97 = control-ref of="PoutR 4"() -> (w76:refnum<vi>)
          n98 = control-ref of="PoutR 5"() -> (w75:refnum<vi>)
          n99 = control-ref of="PoutR 6"() -> (w74:refnum<vi>)
          n100 = control-ref of="Discharge R"() -> (w84:refnum<vi>)
          n101 = control-ref of="Input Pwr"() -> (w73:refnum<vi>)
          n102 = control-ref of="Output_HV"() -> (w72:refnum<vi>)
          n103 = control-ref of="AO"() -> (w71:refnum<vi>)
          n104 = Bundle By Name(cluster=T35 {"relay 1"=refnum, "relay 2"=refnum, "relay 3"=refnum, "relay 4"=refnum, "relay 5"=refnum, "relay 6"=refnum, "PoutR 1"=refnum, "PoutR 2"=refnum, "PoutR 3"=refnum, "PoutR 4"=refnum, "PoutR 5"=refnum, "PoutR 6"=refnum, "Discharge"=refnum, "Input Pwr"=refnum, "Output_HV"=refnum, "AO onoff"=refnum} ("input cluster"), "relay 1"=w86, "relay 2"=w85, "relay 3"=w83, "relay 4"=w82, "relay 5"=w81, "relay 6"=w80, "PoutR 1"=w79, "PoutR 2"=w78, "PoutR 3"=w77, "PoutR 4"=w76, "PoutR 5"=w75, "PoutR 6"=w74, "Discharge"=w84, "Input Pwr"=w73, "Output_HV"=w72, "AO onoff"=w71) -> (w69:T35)
          n105 = call "fgv_ctrl-ref2.vi"("cmd"=rw."write", "input cluster"=w69) -> ()  [unwired: 9 in, 1 out]
        }
        frame #5 {
          n106 = control-ref of="시험 모드"() -> (w94:refnum<vi>)
          n107 = control-ref of="Tab Control_manual"() -> (w93:refnum<vi>)
          n108 = control-ref of="Operation stutus 0"() -> (w103:refnum<vi>)
          n109 = control-ref of="Setting"() -> (w100:refnum<vi>)
          n110 = control-ref of="Manual"() -> (w99:refnum<vi>)
          n111 = control-ref of="Main"() -> (w98:refnum<vi>)
          n112 = control-ref of="RCstart"() -> (w97:refnum<vi>)
          n113 = control-ref of="HW check"() -> (w90:refnum<vi>)
          n114 = control-ref of="login"() -> (w89:refnum<vi>)
          n115 = control-ref of="logout"() -> (w88:refnum<vi>)
          n116 = control-ref of="Operation Status"() -> (w102:refnum<vi>)
          n117 = control-ref of="채널선택"() -> (w96:refnum<vi>)
          n118 = control-ref of="시험명"() -> (w95:refnum<vi>)
          n119 = Bundle(cluster=T36 {"Operation stutus"=refnum, "Test Status"=refnum, "Setting"=refnum, "Manual"=refnum, "Main"=refnum, "RCstart"=refnum, "채널선택"=refnum, "시험명"=refnum, "Tab Control_manual"=refnum, "시험 모드"=refnum, "HW check"=refnum, "login"=refnum, "logout"=refnum} ("output cluster"), "Operation stutus"=w103, "Test Status"=w102, "Setting"=w100, "Manual"=w99, "Main"=w98, "RCstart"=w97, "채널선택"=w96, "시험명"=w95, "Tab Control_manual"=w93, "시험 모드"=w94, "HW check"=w90, "login"=w89, "logout"=w88) -> (w91:T36)
          n120 = call "fgv_UI-sub.vi"("cmd"=rw."write", "output cluster"=w91) -> ()  [unwired: 8 in, 2 out]
          "Operation stutus 0" <- FALSE ("Operation stutus")
        }
        frame #6 {
          n121 = call "fgv_params_save-load_manual.vi"("cmd"=T37."LastRUN Load") -> ("error out"=w117:errorcluster, "Params_all"=w116:T59)  [unwired: 8 in, 1 out]
          n122 = Unbundle By Name(w116) -> ("DL950_config"=→"DL950_config load":T9, "BP4610 Config"=→"BP4610 Config load":T11, "DSP1950 Config"=→"DSP1950 Config load":T12, "cDAQ-9221 Config"=→"cDAQ-9221 Config":T15, "cDAQ-9467 Config"=→"cDAQ-9467 Config load":tag, "cDAQ-9269 AO Config"=→"cDAQ-9269 AO Config":T13, "AO_Wave-config"=→"AO_Wave-config load":T14, "DSP1950 Config LV"=→"DSP1950 Config LV":T12)  [unwired: 1 out]
          n123 = call "sub_load-val.vi"("cmd"=enum16{"load", "save"}."load", "Error in"=w117) -> ("config 2"=→"config 2":T13)  [unwired: 8 in, 1 out]
        }
        frame #7 {
          n124 = call "sub_log-path.vi"() -> ("result path"=w123:path, "log path"=w124:path)  [unwired: 10 in]
          n125 = control-ref of="AI Graph"() -> (w131:refnum<vi>)
          n126 = call "fgv_gloabal-config.vi"("cmd"=rw."read") -> ("config_aging 2"=w128:T60)  [unwired: 10 in]
          n127 = Bundle By Name(cluster=w128, "Setting.Log"=w124, "Setting.result"=w123) -> (w127:T60)
          n128 = call "fgv_AI.vi"("Mode"=system-status."Initial", "Waveform Graph"=w131) -> ()  [unwired: 7 in, 3 out]
          n129 = call "fgv_gloabal-config.vi"("cmd"=rw."write", "config_aging"=w127) -> ()  [unwired: 9 in, 1 out]
          n130 = control-ref of="Status"() -> (w133:refnum<vi>)
          n131 = local read "Log path"() -> (w118:path)
          n132 = call "fgv_status-display.vi"("Mode"=system-status."Initial", "System Log"=w133) -> ()  [unwired: 9 in, 1 out]
          n133 = call "fgv_curr-test-info.vi"("cmd"=rw."read") -> ("현재테스트 정보 2"=w121:T62)  [unwired: 10 in]
          n134 = Bundle By Name(cluster=w121, "Path"=w118) -> (w122:T62)
          n135 = control-ref of="String_dl950"() -> (w129:refnum<vi>)
          n136 = call "fgv_curr-test-info.vi"("cmd"=rw."write", "현재테스트 정보"=w122) -> ()  [unwired: 9 in, 1 out]
          n137 = call "fgv_cmd.vi"("Mode"=system-status."Initial", "System Log"=w129) -> ()  [unwired: 9 in, 1 out]
        }
        frame #8 {
          n138 = call "fgv_DL950_buffer.vi"("cmd"=create-rw-close."create") -> ()  [unwired: 9 in, 2 out]
          n139 = call "fgv_error_rc.vi"("cmd"=init-r-w."init") -> ()  [unwired: 10 in, 1 out]
          n140 = call "fgv_AI_q.vi"("cmd"=create-rw-close."create") -> ()  [unwired: 9 in, 2 out]
          n141 = call "fgv_single-sequence.vi"("cmd"=create-rw-close."create") -> ()  [unwired: 9 in, 2 out]
          n142 = global write "Glob_Ref.vi" "stop"(FALSE ("stop")) -> ()
          n143 = call "fgv_DL950_q.vi"("cmd"=create-rw-close."create") -> ()  [unwired: 9 in, 2 out]
          n144 = call "sub_log_basic.vi"("desc"="log", "Title"="init") -> ()  [unwired: 9 in, 1 out]
          n145 = disable-structure shown="Disabled" {
            frame Disabled {
              n146 = call "fgv_error.vi"("cmd"=rw."write") -> ()  [unwired: 9 in, 2 out]
            }
            frame Enabled {
            }
          }
        }
        frame #9 {
          w153 = FALSE ("Output_Cnt")
          # "설정 초기화"
          n147 = Unbundle By Name(T41 {"Channel selection"={"1ch"=TRUE, "2ch"=TRUE, "3ch"=TRUE, "4ch"=FALSE, "5ch"=FALSE, "6ch"=FALSE}, "Test Cycle"=1, "Repeate"=1} ("Test Config Common")) -> ("Channel selection"=w145:T63)
          n148 = local write "Input Pwr"(w153) -> ()
          n149 = local write "Output_HV"(w153) -> ()
          n150 = local write "Single sequence"(sequence_single."Register" ("Single sequence")) -> ()
          n151 = local write "Tab_menu-select"(Tap_main2."Test" ("Tab_menu-select")) -> ()
          n152 = call "fgv_curr-test-info.vi"("cmd"=rw."read") -> ("현재테스트 정보 2"=w151:T62)  [unwired: 10 in]
          n153 = Bundle By Name(cluster=w151, "Ch selection"=w145) -> (w152:T62)
          n154 = local write "채널선택"(w145) -> ()
          n155 = call "fgv_curr-test-info.vi"("cmd"=rw."write", "현재테스트 정보"=w152) -> ()  [unwired: 9 in, 1 out]
          n156 = call "save_testConditions.vi"("cmd"=cmd_TestParaSave."Read") -> ()  [unwired: 10 in, 1 out]
        }
        frame #10 {
          n157 = call "UI_result.vi"("result"=result."Init") -> ()  [unwired: 10 in, 1 out]
          n158 = call "sub_ui-usertype.vi"("Disabled"=T2."Disabled and Grayed Out") -> ()  [unwired: 11 in]
        }
        frame #11 {
          # "UI init"
          n159 = call "LogIn Infor.vi"("USER IN"=cmd_logInfor."DEFAULT") -> ("Admin?"=w160:bool)  [unwired: 8 in, 2 out]
          n160 = Select(t=UI_dev-operator."Admin" ("cmd"), s=w160, f=UI_dev-operator."Operator" ("cmd")) -> (s? t:f=w158:T43)
          n161 = call "fgv_UI-dev-operator.vi"("cmd"=w158) -> ()  [unwired: 10 in, 1 out]
        }
        frame #12 {
          n162 = vi-ref "Main-sequence.vi"() -> (w161:refnum<vi>)
          n163 = vi-ref "Main_NIAI.vi"() -> (w163:refnum<vi>)
          n164 = vi-ref "dataSave.vi"() -> (w164:refnum<vi>)
          n165 = vi-ref "check Charge.vi"() -> (w165:refnum<vi>)
          n166 = vi-ref "sub_DL950_main.vi"() -> (w162:refnum<vi>)
          n167 = Build Array(w161, w162, w163, w164, w165) -> (w166:refnum<vi>[])
          n168 = for {
            tunnel: w166 -> [w169] mode=indexing
            n169 = property class="VI"(reference=w169) -> (reference out=w167:refnum<vi>, "Exec.State"=w168:T64)  [unwired: 1 in, 1 out]
            n170 = case shown="\"Idle\"" w168 {
              tunnel: w167 -> [_ w172]
              frame "Bad", Default {
              }
              frame "Idle" {
                n171 = invoke class="VI" method="Run VI"(reference=w172, "Wait until done"=FALSE ("Wait Until Done"), "Auto Dispose Ref"=TRUE ("Auto Dispose Reference")) -> ()  [unwired: 2 in, 5 out]
              }
            }
          }
        }
        frame #13 {
          n172 = stacked-sequence {
            tunnel: [_ _ w179 _ _ _ _] -> _
            tunnel: [_ _ _ w183 _ _ _] -> _
            tunnel: [_ _ _ _ w187 _ _] -> _
            tunnel: [_ _ _ _ _ w191 _] -> _
            tunnel: [_ _ _ _ _ _ w201] -> _
            tunnel: [_ w173 _ _ _ _ _] -> _
            frame #0 {
            }
            frame #1 {
              n173 = call "fgv_DL950_q.vi"("cmd"=create-rw-close."write", "data"=start."init") -> ("error out"=w178:errorcluster)  [unwired: 8 in, 1 out]
              n174 = call "fgv_DL950_q.vi"("cmd"=create-rw-close."write", "error in"=w178, "data"=start."close") -> ("error out"=w173:errorcluster)  [unwired: 7 in, 1 out]
            }
            frame #2 {
              n175 = call "fgv_DSP_visa.vi"("action"=DSP_action."cont") -> ("error out"=w182:errorcluster)  [unwired: 10 in]
              n176 = call "fgv_DSP_visa.vi"("action"=DSP_action."discont", "error in"=w182) -> ("error out"=w179:errorcluster)  [unwired: 9 in]
            }
            frame #3 {
              n177 = call "fgv_4610_visa.vi"("cmd"=BP4610_cmd."open") -> ("error out"=w186:errorcluster)  [unwired: 10 in]
              n178 = call "fgv_4610_visa.vi"("cmd"=BP4610_cmd."close", "error in"=w186) -> ("error out"=w183:errorcluster)  [unwired: 9 in]
            }
            frame #4 {
              n179 = call "fgv_AO_daqmx.vi"("cmd"=init-w-close."open") -> ("error out"=w190:errorcluster)  [unwired: 10 in]
              n180 = call "fgv_AO_daqmx.vi"("cmd"=init-w-close."close", "error in"=w190) -> ("error out"=w187:errorcluster)  [unwired: 9 in]
            }
            frame #5 {
              n181 = call "fgv_DO-daqmx.vi"("cnt"=cnt_do."open") -> ("error out"=w196:errorcluster)  [unwired: 10 in]
              n182 = for {
                tunnel: cluster{"Relay":T49, "Boolean":bool}[] [{"Relay"=enum."R_in1", "Boolean"=FALSE}, {"Relay"=enum."R_in2", "Boolean"=FALSE}, {"Relay"=enum."R_in3", "Boolean"=FALSE}, {"Relay"=enum."R_in4", "Boolean"=FALSE}, {"Relay"=enum."R_in5", "Boolean"=FALSE}, {"Relay"=enum."R_in6", "Boolean"=FALSE}, {"Relay"=enum."R_out1", "Boolean"=FALSE}, {"Relay"=enum."R_out2", "Boolean"=FALSE}, {"Relay"=enum."R_out3", "Boolean"=FALSE}, {"Relay"=enum."R_out4", "Boolean"=FALSE}, {"Relay"=enum."R_out5", "Boolean"=FALSE}, {"Relay"=enum."R_out6", "Boolean"=FALSE}] -> [w200] mode=indexing
                tunnel: [w198] -> w195
                tunnel: w196 -> [w197]
                n183 = call "fgv_DO-daqmx.vi"("cnt"=cnt_do."update", "error in"=w197, "Relay"=w200) -> ("error out"=w198:errorcluster)  [unwired: 8 in]
              }
              n184 = call "fgv_DO-daqmx.vi"("cnt"=cnt_do."run", "error in"=w195) -> ("error out"=w191:errorcluster)  [unwired: 9 in]
            }
            frame #6 {
              n185 = call "fgv_AI_q.vi"("cmd"=create-rw-close."write", "data"=start."start") -> ("error out"=w201:errorcluster)  [unwired: 8 in, 1 out]
            }
          }
        }
        frame #14 {
          n186 = while {
            shift-right: [w206] -> _
            shift-left: _ -> [w209]
            i -> [w204]
            stop <- w207 stop-if-true
            n187 = event shown="[22] \"ES 규격시험 선택\": Value Change" {
              selector: _ -> [_ _ _ _ _ _ _ _ _ _ _ _ _ _ _ _ _ _ _ _ _ _ _ _ _ _ _ _ _ _ _ _ _ _ _ _ _ _ _ _ _ _]
              dyn-events: _ -> [_ _ _ _ _ _ _ _ _ _ _ _ _ _ _ _ _ _ _ _ _ _ _ _ _ _ _ _ _ _ _ _ _ _ _ _ _ _ _ _ _ _]
              timeout: 200 -> [_ _ _ _ _ _ _ _ _ _ _ _ _ _ _ _ _ _ _ _ _ _ _ _ _ _ _ _ _ _ _ _ _ _ _ _ _ _ _ _ _ _]
              tunnel: w209 -> [_ _ w252 _ _ _ _ _ _ _ _ _ _ _ _ _ _ _ _ _ w563 _ _ _ _ _ _ _ _ _ _ _ _ _ _ _ _ _ _ _ _ _]
              tunnel: [_ _ w257 _ _ _ _ _ _ _ _ _ _ _ _ _ _ _ _ _ _ _ _ _ _ _ _ _ _ _ _ _ _ _ _ _ _ _ _ _ _ _] -> w206
              tunnel: [w214 _ _ _ _ _ _ _ _ _ _ _ _ _ _ _ _ _ _ _ _ _ _ _ _ _ _ _ _ _ _ _ _ _ _ _ _ _ _ _ _ _] -> w208
              tunnel: w204 -> [_ _ _ _ _ _ _ _ _ _ _ _ _ _ _ _ _ _ _ _ _ _ _ _ _ _ _ _ _ _ _ _ _ _ _ _ _ _ _ _ _ _]
              event "exit": Value Change {
                n188 = event-data() -> ()  [unwired: 1 in, 1 out]
                n189 = Two Button Dialog(message="프로그램을 종료합니다.", 1:"아니요" ("F button name (\"Cancel\")"), 2:"예" ("T button name (\"OK\")")) -> (T button?=w210:bool)
                n190 = case shown="True" w210 {
                  tunnel: [FALSE ("stop") w216] -> w214
                  frame False {
                  }
                  frame True {
                    n191 = stacked-sequence {
                      tunnel: [_ w221 _ _] -> _
                      tunnel: [_ w220 _ _] -> _
                      frame #0 {
                        n192 = call "sub_log_basic.vi"("desc"="click", "Title"="Exit button") -> ()  [unwired: 9 in, 1 out]
                      }
                      frame #1 {
                        n193 = call "fgv_DO-daqmx.vi"("cnt"=cnt_do."initial") -> ("error out"=w225:errorcluster)  [unwired: 10 in]
                        n194 = call "fgv_DO-daqmx.vi"("cnt"=cnt_do."update", "error in"=w225, "Relay"=cluster{"Relay":T49, "Boolean":bool} {"Relay"=enum."R_green", "Boolean"=TRUE}) -> ("error out"=w222:errorcluster)  [unwired: 8 in]
                        n195 = call "fgv_DO-daqmx.vi"("cnt"=cnt_do."run", "error in"=w222) -> ("error out"=w221:errorcluster)  [unwired: 9 in]
                        n196 = Wait (ms)(milliseconds to wait=u32 1000) -> ()  [unwired: 1 out]
                        n197 = call "sub_hw-set.vi"("cmd"=hw-control."relay all-off") -> ("error out"=w220:errorcluster)  [unwired: 10 in]
                      }
                      frame #2 {
                        n198 = call "fgv_DL950_q.vi"("cmd"=create-rw-close."write", "data"=start."exit") -> ()  [unwired: 8 in, 2 out]
                      }
                      frame #3 {
                        n199 = call "fgv_AI_q.vi"("cmd"=create-rw-close."close") -> ()  [unwired: 9 in, 2 out]
                        n200 = call "fgv_single-sequence.vi"("cmd"=create-rw-close."close") -> ()  [unwired: 9 in, 2 out]
                        n201 = call "fgv_DL950_buffer.vi"("cmd"=create-rw-close."close") -> ()  [unwired: 9 in, 2 out]
                        n202 = call "fgv_DL950_q.vi"("cmd"=create-rw-close."close") -> ()  [unwired: 9 in, 2 out]
                      }
                    }
                    n203 = call "fgv_stop_global.vi"("cmd"=init-r-stop."stop") -> ("stop"=w216:bool)  [unwired: 10 in]
                  }
                }
              }
              event "stop": Value Change {
                n204 = event-data() -> ()  [unwired: 1 in, 1 out]
                n205 = Two Button Dialog(message="시험을 종료합니다.", 1:"아니오" ("T button name (\"OK\")"), 2:"예" ("T button name (\"OK\")")) -> (T button?=w236:bool)
                n206 = case shown="True" w236 {
                  frame False {
                  }
                  frame True {
                    n207 = call "fgv_DL950_q.vi"("cmd"=create-rw-close."write", "data"=start."stop") -> ()  [unwired: 8 in, 2 out]
                    n208 = call "UI_result.vi"("result"=result."Shutdown") -> ()  [unwired: 10 in, 1 out]
                    n209 = global write "Glob_Ref.vi" "stop"(TRUE ("stop")) -> ()
                    n210 = call "sub_log_basic.vi"("desc"="click", "Title"="Stop Button") -> ()  [unwired: 9 in, 1 out]
                    n211 = call "task stop.vi"() -> ()  [unwired: 11 in, 1 out]
                    n212 = call "fgv_stop_local.vi"("cmd"=init-r-stop."stop") -> ()  [unwired: 9 in, 2 out]
                    n213 = call "sub_alarm-led.vi"("alarm"=T28."yellow", "onoff"=FALSE) -> ()  [unwired: 9 in, 1 out]
                  }
                }
              }
              event "Read_DLM5058", "con_DLM5058", "discon_DLM5058", "M_Stop_DLM5058", "M_Start_DLM5058", "Apply_DLM5058", "Query_DLM5058", "ResetItem_DLM5058", "ReadItem_DLM5058", "Trigger_single": Value Change {
                n214 = event-data() -> ("CtlRef"=w256:refnum<vi>)  [unwired: 1 in]
                n215 = property class="Bool"(reference=w256) -> ("Label.Text"=w255:string)  [unwired: 1 in, 2 out]
                n216 = local read "DL950_config"() -> (w254:T9)
                n217 = call "fgv_DL950_config.vi"("cmd"=rw."write", "error in"=w252, "config"=w254) -> ("error out"=w251:errorcluster)  [unwired: 7 in, 1 out]
                n218 = call "fgv_status-display.vi"("Mode"=system-status."Clear") -> ("error out"=w249:errorcluster)  [unwired: 10 in]
                n219 = case shown="\"Apply_DLM5058\"" w255 {
                  tunnel: w251 -> [w258 w259 w263 w267 w271 w276 w280 w284 w288 w292 w296 w301]
                  tunnel: [w258 w260 w264 w268 w272 w275 w279 w283 w287 w291 w295 w300] -> w257
                  tunnel: w249 -> [_ _ _ _ _ _ _ _ _ _ _ _]
                  frame "False", Default {
                  }
                  frame "Apply_DLM5058" {
                    n220 = call "fgv_DL950_q.vi"("cmd"=create-rw-close."write", "error in"=w259, "data"=start."set") -> ("error out"=w260:errorcluster)  [unwired: 7 in, 1 out]
                  }
                  frame "ResetItem_DLM5058" {
                    n221 = call "fgv_DL950_q.vi"("cmd"=create-rw-close."write", "error in"=w263, "data"=start."reset") -> ("error out"=w264:errorcluster)  [unwired: 7 in, 1 out]
                  }
                  frame "con_DLM5058" {
                    n222 = call "fgv_DL950_q.vi"("cmd"=create-rw-close."write", "error in"=w267, "data"=start."init") -> ("error out"=w268:errorcluster)  [unwired: 7 in, 1 out]
                  }
                  frame "set_DLM5058" {
                    n223 = call "fgv_DL950_q.vi"("cmd"=create-rw-close."write", "error in"=w271, "data"=start."set") -> ("error out"=w272:errorcluster)  [unwired: 7 in, 1 out]
                  }
                  frame "discon_DLM5058" {
                    n224 = call "fgv_DL950_q.vi"("cmd"=create-rw-close."write", "error in"=w276, "data"=start."close") -> ("error out"=w275:errorcluster)  [unwired: 7 in, 1 out]
                  }
                  frame "M_Start_DLM5058" {
                    n225 = call "fgv_DL950_q.vi"("cmd"=create-rw-close."write", "error in"=w280, "data"=start."start") -> ("error out"=w279:errorcluster)  [unwired: 7 in, 1 out]
                  }
                  frame "M_Stop_DLM5058" {
                    n226 = call "fgv_DL950_q.vi"("cmd"=create-rw-close."write", "error in"=w284, "data"=start."stop") -> ("error out"=w283:errorcluster)  [unwired: 7 in, 1 out]
                  }
                  frame "Read_DLM5058" {
                    n227 = call "fgv_DL950_q.vi"("cmd"=create-rw-close."write", "error in"=w288, "data"=start."read") -> ("error out"=w287:errorcluster)  [unwired: 7 in, 1 out]
                  }
                  frame "ReadItem_DLM5058" {
                    n228 = call "fgv_DL950_q.vi"("cmd"=create-rw-close."write", "error in"=w292, "data"=start."read_items") -> ("error out"=w291:errorcluster)  [unwired: 7 in, 1 out]
                  }
                  frame "Trigger_single" {
                    n229 = call "fgv_DL950_q.vi"("cmd"=create-rw-close."write", "error in"=w296, "data"=start."T_single") -> ("error out"=w295:errorcluster)  [unwired: 7 in, 1 out]
                  }
                  frame "Query_DLM5058" {
                    n230 = call "fgv_DL950_q.vi"("cmd"=create-rw-close."write", "error in"=w301, "data"=start."query") -> ("error out"=w300:errorcluster)  [unwired: 7 in, 1 out]
                    n231 = global write "Global 1.vi" "String"("String") -> ()
                  }
                }
              }
              event Value Change {
                n232 = event-data() -> ("CtlRef"=w307:refnum<vi>)  [unwired: 1 in, 2 out]
                n233 = property class="Clust"(reference=w307) -> ("Label.Text"=w306:string)  [unwired: 1 in, 2 out]
                n234 = case shown="\"DL950_config\"" w306 {
                  tunnel: "DSP1500 Config" -> [_ _ _ w313]
                  tunnel: "DSP Config LV" -> [_ _ _ w312]
                  frame "거짓", Default {
                  }
                  frame "DL950_config" {
                    n235 = call "fgv_DL950_config.vi"("cmd"=rw."write", "config"="DL950_config") -> ()  [unwired: 8 in, 2 out]
                  }
                  frame "BP4610 config" {
                    n236 = call "fgv_4610_config.vi"("cmd"=rw."write", "BP4610 Config"="BP4610 Config") -> ()  [unwired: 8 in, 2 out]
                  }
                  frame "DSP1500 Config" {
                    n237 = call "fgv_DSP_config.vi"("cmd"=rw."write", "DSP Config LV IN"=w312, "DSP Config HV IN"=w313) -> ()  [unwired: 6 in, 3 out]
                  }
                }
              }
              event "Input Pwr", "Open BP4610", "Close BP4610", "Apply BP4610": Value Change {
                n238 = event-data() -> ("CtlRef"=w317:refnum<vi>)  [unwired: 1 in]
                n239 = local read "BP4610 Config"() -> (w315:T11)
                n240 = property class="Bool"(reference=w317) -> ("Label.Text"=w316:string)  [unwired: 1 in, 2 out]
                n241 = case shown="\"Input Pwr\"" w316 {
                  tunnel: w315 -> [_ _ w322 w329 w333 w339]
                  frame "False", Default {
                  }
                  frame "Update BP4610" {
                  }
                  frame "Input Pwr" {
                    (unwired) FALSE
                    n242 = call "fgv_4610_config.vi"("cmd"=rw."write", "BP4610 Config"=w322) -> ("error out"=w318:errorcluster)  [unwired: 8 in, 1 out]
                    n243 = Select(t=BP4610_cmd."output on" ("action"), s="Input Pwr", f=BP4610_cmd."output off" ("action")) -> (s? t:f=w319:T46)
                    n244 = call "fgv_4610_visa.vi"("cmd"=w319, "error in"=w318) -> ("error out"=w320:errorcluster)  [unwired: 9 in]
                    n245 = case shown="True" FALSE {
                      tunnel: w320 -> [_ _]
                      frame False {
                      }
                      frame True {
                      }
                    }
                  }
                  frame "Close BP4610" {
                    n246 = call "fgv_4610_config.vi"("cmd"=rw."write", "BP4610 Config"=w329) -> ("error out"=w327:errorcluster)  [unwired: 8 in, 1 out]
                    n247 = call "fgv_4610_visa.vi"("cmd"=BP4610_cmd."close", "error in"=w327) -> ()  [unwired: 9 in, 1 out]
                  }
                  frame "Open BP4610" {
                    n248 = call "fgv_4610_config.vi"("cmd"=rw."write", "BP4610 Config"=w333) -> ("error out"=w331:errorcluster)  [unwired: 8 in, 1 out]
                    n249 = call "fgv_4610_visa.vi"("cmd"=BP4610_cmd."open", "error in"=w331) -> ()  [unwired: 9 in, 1 out]
                  }
                  frame "Apply BP4610" {
                    (unwired) T11 {"VISA"="USB0::0x0D4A::0x0040::9426270::INSTR", "Limit-BP"={"Set"=enum."Current", "Voltage+[V]"=20.0, "Current+[A]"=5.0, "Voltage-[V]"=-20.0, "Current-[A]"=-5.0}, "SET BP"={"Set"=enum."Voltage", "Operation mode"=1, "Voltage[Vp-p]"=20.0, "Current[Ap-p]"=5.0, "Voltage[V]"=12.0, "Current[A]"=5.0, "Frequency[Hz]"=100.0, "Waveform"=enum."Square"}} ("BP4610 Config 2")
                    n250 = call "fgv_4610_config.vi"("cmd"=rw."write", "BP4610 Config"=w339) -> ("error out"=w335:errorcluster)  [unwired: 8 in, 1 out]
                    n251 = call "fgv_4610_visa.vi"("cmd"=BP4610_cmd."set", "error in"=w335) -> ("error out"=w336:errorcluster)  [unwired: 9 in]
                    n252 = call "fgv_4610_visa.vi"("cmd"=BP4610_cmd."limit", "error in"=w336) -> ()  [unwired: 9 in, 1 out]
                  }
                }
              }
              event "HW config": Value Change {
                n253 = event-data() -> ()  [unwired: 1 in, 1 out]
                n254 = call "sub_test-start.vi"() -> ()  [unwired: 11 in, 1 out]
              }
              event "Set_idrc", "Open DSP", "Close DSP", "Output_HV", "read_dsp", "DSP Selection", "Output_LV": Value Change {
                n255 = event-data() -> ("CtlRef"=w345:refnum<vi>)  [unwired: 1 in, 2 out]
                n256 = local read "DSP1500 Config"() -> (w343:T12)
                n257 = local read "DSP Config LV"() -> (w342:T12)
                n258 = property class="Ctl"(reference=w345) -> ("Label.Text"=w344:string)  [unwired: 1 in, 2 out]
                n259 = case shown="\"Set_idrc\"" w344 {
                  tunnel: w343 -> [_ w351 _ w357 w362 _ w368 w377]
                  tunnel: w342 -> [_ w346 _ w354 w359 _ w366 w375]
                  tunnel: "DSP Selection" -> [_ _ _ _ _ w364 _ _]
                  frame "False", Default {
                  }
                  frame "Set_idrc" {
                    n260 = call "fgv_DSP_config.vi"("cmd"=rw."write", "DSP Config LV IN"=w346, "DSP Config HV IN"=w351) -> ("error out"=w348:errorcluster)  [unwired: 6 in, 2 out]
                    n261 = call "fgv_DSP_visa.vi"("action"=DSP_action."protection", "error in"=w348) -> ("error out"=w347:errorcluster)  [unwired: 9 in]
                    n262 = call "fgv_DSP_visa.vi"("action"=DSP_action."level_m", "error in"=w347) -> ()  [unwired: 9 in, 1 out]
                  }
                  frame "read_dsp" {
                    n263 = call "fgv_DSP_visa.vi"("action"=DSP_action."read") -> ()  [unwired: 10 in, 1 out]
                  }
                  frame "Open DSP" {
                    n264 = call "fgv_DSP_config.vi"("cmd"=rw."write", "DSP Config LV IN"=w354, "DSP Config HV IN"=w357) -> ("error out"=w355:errorcluster)  [unwired: 6 in, 2 out]
                    n265 = call "fgv_DSP_visa.vi"("action"=DSP_action."cont", "error in"=w355) -> ()  [unwired: 9 in, 1 out]
                  }
                  frame "Close DSP" {
                    n266 = call "fgv_DSP_config.vi"("cmd"=rw."write", "DSP Config LV IN"=w359, "DSP Config HV IN"=w362) -> ("error out"=w360:errorcluster)  [unwired: 6 in, 2 out]
                    n267 = call "fgv_DSP_visa.vi"("action"=DSP_action."discont", "error in"=w360) -> ()  [unwired: 9 in, 1 out]
                  }
                  frame "DSP Selection" {
                    n268 = global write "Glob_Ref.vi" "DSP Selection"(w364) -> ()
                  }
                  frame "Output_HV" {
                    n269 = call "fgv_DSP_config.vi"("cmd"=rw."write", "DSP Config LV IN"=w366, "DSP Config HV IN"=w368) -> ("error out"=w365:errorcluster)  [unwired: 6 in, 2 out]
                    n270 = Select(t=DSP_action."on" ("action"), s="Output_HV", f=DSP_action."off" ("action")) -> (s? t:f=w367:T45)
                    n271 = call "fgv_DSP_visa.vi"("action"=w367, "error in"=w365) -> ()  [unwired: 9 in, 1 out]
                  }
                  frame "Output_LV" {
                    n272 = call "fgv_DSP_config.vi"("cmd"=rw."write", "DSP Config LV IN"=w375, "DSP Config HV IN"=w377) -> ("error out"=w373:errorcluster)  [unwired: 6 in, 2 out]
                    n273 = Select(t=DSP_action."on" ("action"), s="Output_LV", f=DSP_action."off" ("action")) -> (s? t:f=w376:T45)
                    n274 = call "fgv_DSP_visa.vi"("action"=w376, "error in"=w373) -> ()  [unwired: 9 in, 1 out]
                  }
                }
              }
              event "AO 12v": Value Change {
                (unwired) FALSE
                n275 = event-data() -> ()  [unwired: 1 in, 1 out]
                n276 = call "sub_hw-set.vi"("cmd"=hw-control."AO 12v") -> ()  [unwired: 10 in, 1 out]
              }
              event "RC setting": Value Change {
                n277 = event-data() -> ()  [unwired: 1 in, 1 out]
                n278 = flat-sequence {
                  frame #0 {
                    n279 = call "Evn-settings.vi"("setting type"=hwsetting."BP4610 RC") -> ()  [unwired: 11 in]
                  }
                  frame #1 {
                    n280 = call "Evn-settings.vi"("setting type"=hwsetting."DSP1500 RC") -> ()  [unwired: 11 in]
                  }
                }
              }
              event "AO 0v": Value Change {
                n281 = event-data() -> ()  [unwired: 1 in, 1 out]
                n282 = call "sub_hw-set.vi"("cmd"=hw-control."AO 0v") -> ()  [unwired: 10 in, 1 out]
              }
              event "Shutdown": Value Change {
                n283 = event-data() -> ()  [unwired: 1 in, 1 out]
                n284 = call "sub_shutdown.vi"() -> ()  [unwired: 11 in, 1 out]
              }
              event "BP4610 on": Value Change {
                n285 = event-data() -> ()  [unwired: 1 in, 1 out]
                n286 = call "sub_hw-set.vi"("cmd"=hw-control."BP4610 onoff", "onoff"=TRUE) -> ()  [unwired: 9 in, 1 out]
              }
              event "BP4610 off": Value Change {
                n287 = event-data() -> ()  [unwired: 1 in, 1 out]
                n288 = call "sub_hw-set.vi"("cmd"=hw-control."BP4610 onoff", "onoff"=FALSE) -> ()  [unwired: 9 in, 1 out]
              }
              event "relay all off": Value Change {
                n289 = event-data() -> ()  [unwired: 1 in, 1 out]
                n290 = call "sub_hw-set.vi"("cmd"=hw-control."relay all-off") -> ()  [unwired: 10 in, 1 out]
              }
              event "Clear scope graph": Value Change {
                n291 = event-data() -> ()  [unwired: 1 in, 1 out]
                n292 = call "fgv_ctrl-ref.vi"("cmd"=rw."read") -> ("output cluster 2"=w392:T33)  [unwired: 9 in, 1 out]
                n293 = Unbundle By Name(w392) -> ("DL950 wfm"=w391:refnum<vi>)
                n294 = property class="WFGraph (strict)"(reference=w391, "Value"=waveform(dbl)[] []) -> ()  [unwired: 1 in, 2 out]
              }
              event "Button": Value Change {
                n295 = event-data() -> ()  [unwired: 1 in, 6 out]
                n296 = call "fgv_ctrl-ref.vi"("cmd"=rw."read") -> ("output cluster 2"=w396:T33)  [unwired: 9 in, 1 out]
                n297 = Unbundle By Name(w396) -> ("Testconfig"=w395:refnum<vi>)
                n298 = property class="Clust (strict)"(reference=w395) -> ("Controls[]"=w400:refnum<vi>[])  [unwired: 1 in, 2 out]
                n299 = Index Array(array=w400, index="index") -> (element=w398:refnum<vi>)
                n300 = property class="Ctl"(reference=w398, "DisabledEnum"="Disabled") -> ("Label.Text"=→"Label.Text":string)  [unwired: 1 in, 2 out]
              }
              event "Manual", "Setting", "Main": Value Change {
                n301 = event-data() -> ("CtlRef"=w405:refnum<vi>)  [unwired: 1 in]
                n302 = property class="Bool"(reference=w405) -> ("Label.Text"=w404:string)  [unwired: 1 in, 2 out]
                n303 = case shown="\"Setting\"" w404 {
                  tunnel: [Tap_main2."Manual" ("Tab_menu-select") Tap_main2."Test" ("Tab_menu-select") Tap_main2."Setting" ("Tab_menu-select") Tap_main2."Manual" ("Tab_menu-select") Tap_main2."Manual" ("Tab_menu-select") Tap_main2."Manual" ("Tab_menu-select") Tap_main2."Setting" ("Tab_menu-select")] -> w403
                  tunnel: [TRUE ("manual?") _ _ _ _ _ _] -> w402
                  frame "Manual", Default {
                    n304 = call "sub_log_basic.vi"("desc"="click", "Title"="Manual button") -> ()  [unwired: 9 in, 1 out]
                  }
                  frame "Main" {
                    n305 = call "sub_log_basic.vi"("desc"="click", "Title"="Main button") -> ()  [unwired: 9 in, 1 out]
                  }
                  frame "Rload" {
                  }
                  frame "B1" {
                  }
                  frame "B2" {
                  }
                  frame "B3" {
                  }
                  frame "Setting" {
                    n306 = call "TestModeUpdate.vi"("Update?"=FALSE) -> ()  [unwired: 9 in, 2 out]
                    n307 = call "sub_log_basic.vi"("desc"="click", "Title"="Setting button") -> ()  [unwired: 9 in, 1 out]
                    n308 = local read "시험 모드"() -> (w417:T4)
                    n309 = call "setting cable.vi"("시험 모드"=w417) -> ()  [unwired: 10 in, 1 out]
                  }
                }
                n310 = global write "Global_내구.vi" "manual?"(w402) -> ()
                n311 = local write "Tab_menu-select"(w403) -> ()
              }
              event Timeout {
                n312 = event-data() -> ()  [unwired: 1 in, 1 out]
                n313 = call "fgv_rc-config.vi"("cmd"=rw."read") -> ("Testconfig out"=w422:T19)  [unwired: 9 in, 1 out]
                n314 = stacked-sequence {
                  tunnel: w422 -> [w424 _ _ _ w506 w529]
                  frame #0 {
                    n315 = call "fgv_error.vi"("cmd"=rw."read") -> ("error cluster 2"=w438:T3)  [unwired: 9 in, 1 out]
                    "HW error" <- w438
                    n316 = global read "Glob_Ref.vi" "testState"() -> (w432:T43)
                    n317 = Cluster To Array(cluster=w438) -> (array=w437:bool[])
                    n318 = Or Array Elements(Boolean array=w437) -> (logical OR=w428:bool)
                    n319 = case shown="\"Admin\", Default" w432 {
                      tunnel: w428 -> [_ w443]
                      frame "Testing" {
                      }
                      frame "Admin", Default {
                        n320 = call "fgv_UI-sub.vi"("cmd"=rw."read") -> ("output cluster 2"=w445:T36)  [unwired: 9 in, 1 out]
                        n321 = Unbundle By Name(w445) -> ("RCstart"=w444:refnum<vi>)
                        n322 = Select(t=T2."Disabled and Grayed Out" ("Disabled"), s=w443, f=T2."Enabled" ("Disabled")) -> (s? t:f=w440:T2)
                        n323 = property class="Bool"(reference=w444, "DisabledEnum"=w440) -> ()  [unwired: 1 in, 2 out]
                      }
                    }
                    n324 = Select(t="H/W 점검이 필요합니다." ("H/W Status"), s=w428, f="정상운영 중입니다." ("H/W Status")) -> (s? t:f=w429:string)
                    n325 = Select(t=u32 16711680, s=w428, f=u32 0) -> (s? t:f=w426:u32)
                    n326 = property on="HW check" class="Bool"("Blinking"=w428) -> ()  [unwired: 2 in, 2 out]
                    n327 = call "sub_alarm-led.vi"("alarm"=T28."red", "onoff"=w428) -> ("error out"=w435:errorcluster)  [unwired: 9 in]
                    n328 = Not(x=w428) -> (.not. x?=w433:bool)
                    n329 = property on="H/W Status" class="Str"("Value"=w429, "Text.TextColor"=w426) -> ()  [unwired: 2 in, 2 out]
                    n330 = call "sub_alarm-led.vi"("alarm"=T28."green", "error in"=w435, "onoff"=w433) -> ()  [unwired: 8 in, 1 out]
                    "Testconfig out" <- w424
                  }
                  frame #1 {
                    n331 = local read "Single sequence"() -> (w447:T6)
                    n332 = call "fgv_AI.vi"("Mode"=system-status."Read") -> ("mean-vals"=w449:dbl[])  [unwired: 8 in, 2 out]
                    "Means" <- w449
                    n333 = Index Array(array=w449) -> (element=→"캡충전전압[V]" →"Voltage_Charge":dbl)  [unwired: 1 in]
                    n334 = global write "Glob_Ref.vi" "Single sequence"(w447) -> ()
                  }
                  frame #2 {
                    n335 = call "fgv_AO_DAQmx-Config.vi"("cmd"=rw."read") -> ("config 2"=w470:T13)  [unwired: 9 in, 1 out]
                    n336 = global read "Glob_Ref.vi" "DSP Selection"() -> (→"DSP Selection 2":enum32{"DSP HV", "DSP LV"})
                    n337 = global read "Global 1.vi" "read_dl950 2"() -> (→"read_dl950":string)
                    n338 = Unbundle By Name(w470) -> ("Ch"=→"Ch":tag, "Max V"=→"Max V":dbl, "Min V"=→"Min V":dbl, "Rate"=→"Rate":dbl, "N pts"=→"N pts":i32, "sample mode"=→"sample mode":i32)
                    n339 = global read "Global 1.vi" "dt(ms)_finish"() -> (→"dt(ms)_finish":u32)
                    n340 = global read "Global 1.vi" "da950_array"() -> (w477:dbl[])
                    n341 = global read "Glob_Ref.vi" "Array_temp"() -> (→"Array_temp":T10)
                    n342 = global read "Global 1.vi" "950Trigger"() -> (→"950Trigger":i32)
                    n343 = global read "Global 1.vi" "dt(ms)_hw"() -> (→"dt(ms)_hw":u32)
                    n344 = global read "Global_params.vi" "trig delay"() -> (→"trig delay":u32)
                    n345 = global read "Global_params.vi" "Time Div"() -> (→"Time Div":u32)
                    n346 = global read "Global 1.vi" "T1"() -> (→"T1":dbl)
                    n347 = global read "Global 1.vi" "T2"() -> (→"T2":dbl)
                    n348 = local write "DL950 read"(w477) -> ()
                    n349 = global read "Global_params.vi" "error out task stop"() -> (→"error out task stop":errorcluster)
                    n350 = global read "Global_params.vi" "error out wait Ao"() -> (→"error out wait Ao":errorcluster)
                    n351 = global read "Global_params.vi" "Time Div_Init"() -> (→"Time Div_Init":u16)
                    n352 = global read "Global 1.vi" "data_relay"() -> (→"data_relay":bool[])
                    n353 = global read "Global_params.vi" "trig delay_ready"() -> (→"trig delay_ready":u32)
                    n354 = global read "Global_params.vi" "error out"() -> (→"error out":errorcluster)
                    n355 = global read "Global_params.vi" "OFF Time out"() -> (→"OFF Time out":u32)
                    n356 = global read "Global_params.vi" "OFF Time in"() -> (→"OFF Time in":u32)
                  }
                  frame #3 {
                    n357 = global read "Glob_Ref.vi" "Control Signal_LV"() -> (→"Control Signal_LV":T5)
                    n358 = global read "Global_params.vi" "measure_rc 동작"() -> (→"measure_rc 동작":T21)
                    n359 = global read "Glob_Ref.vi" "NumData_OLV"() -> (→"NumData_OLV":dbl)
                    n360 = call "fgv_error_rc.vi"("cmd"=init-r-w."read") -> ("Error 2"=→"Error":T23)  [unwired: 10 in]
                    n361 = call "fgv_DL950_data.vi"("cmd"=rw."read") -> ("DL950 wfm 2"=w486:T65)  [unwired: 9 in, 1 out]
                    n362 = Unbundle By Name(w486) -> ("da950_array"=→"da950_array":dbl[])
                    n363 = call "fgv_measure_reg.vi"("cmd"=rw."read") -> ("measure_reg 2"=→"measure_LV 동작":T20)  [unwired: 10 in]
                    n364 = call "fgv_measure_contR.vi"("cmd"=rw."read") -> ("measure_ContR Out"=→"measure_ContR Out":T22)  [unwired: 9 in, 1 out]
                  }
                  frame #4 {
                    n365 = Unbundle By Name(w506) -> ("Repeate (Each Ch)"=→"반복 회수(세팅)":u32, "Cycle[N]"=→"사이클 회수(세팅)":u32, "Time Div"=→"Time Div_set":u16)  [unwired: 1 out]
                    n366 = call "fgv_curr-test-info.vi"("cmd"=rw."read") -> ("현재테스트 정보 2"=w514:T62)  [unwired: 10 in]
                    n367 = global read "Global 1.vi" "작동회수"() -> (w499:i32)
                    n368 = Unbundle By Name(w514) -> ("TestType"=→"TestType":T6, "현재회수"=w510:u32, "테스트 회수"=w511:u32, "현재채널번호"=w507:u8)
                    "사이클 회수(현재)" <- w510
                    n369 = Increment(x=w499) -> (x+1=→"스위칭 채널 개 수[N]":i32)
                    n370 = Decrement(x=w510) -> (x-1=w497:u32)
                    n371 = Increment(x=w507) -> (x+1=→"채널":u8)
                    n372 = To Double Precision Float(number=w497) -> (double precision float=w505:dbl)
                    n373 = To Double Precision Float(number=w511) -> (double precision float=w504:dbl)
                    n374 = Divide(x=w505, y=w504) -> (x/y=w515:dbl)
                    n375 = Multiply(x=w515, y=100.0) -> (x*y=w516:dbl)
                    n376 = To Unsigned Byte Integer(number=w516) -> (unsigned 8bit integer=w494:u8)
                    n377 = global read "Glob_setting.vi" "result"() -> (w496:T18)
                    "result" <- w496
                    n378 = call "Timer - 1.vi"("cmd"=cmd_timer."default") -> ("update"=→"스위칭 경과 시간(초)":dbl)  [unwired: 8 in, 2 out]
                    n379 = call "fgv_AO_wave.vi"("cmd"=rw."read") -> ("signal out"=→"AO Waveform Graph":waveform(dbl))  [unwired: 9 in, 1 out]
                    n380 = call "ch act update.vi"("cmd"=cmd_ch_act."update", "현재채널번호"=w507) -> ()  [unwired: 9 in, 1 out]
                    n381 = case shown="\"OK\", Default" w496 {
                      tunnel: [u8 0 ("사이클(%)") w518 u8 100 ("사이클(%)")] -> w495
                      tunnel: w494 -> [_ w518 _]
                      frame "Init" {
                      }
                      frame "OK", Default {
                      }
                      frame "Completion" {
                      }
                    }
                    "전체 사이클(%)" <- w495
                  }
                  frame #5 {
                    w521 = 100.0 ("y")
                    n382 = global read "Global 1.vi" "Elapsed Time 미작동"() -> (w531:dbl)
                    "미작동 경과시간(초)" <- w531
                    n383 = Unbundle By Name(w529) -> ("1. 작동시간[분]"=w536:dbl, "2. 미작동시간[분]"=w535:dbl, "3. 작동시간[분]"=w534:dbl, "출력전압[V]"=→"출력전압[V]":dbl, "출력전류[A]"=→"출력전류[A]":dbl, "OVP Level"=→"OVP Level":dbl, "OCP Level"=→"OCP Level":dbl)  [unwired: 2 out]
                    n384 = global read "Global 1.vi" "Elapsed Time 작동"() -> (w526:dbl)
                    "작동시간(초)" <- w526
                    n385 = Compound Arithmetic op=ADD(w536, w535, w534) -> (w533:dbl)
                    n386 = Add(x=w526, y=w531) -> (x+y=w532:dbl)
                    n387 = Multiply(x=60.0, y=w533) -> (x*y=w528:dbl)
                    n388 = Divide(x=100.0, y=w528) -> (x/y=w524:dbl)
                    n389 = Multiply(x=w532, y=w524) -> (x*y=w522:dbl)
                    n390 = Greater Or Equal?(x=w522, y=w521) -> (x >= y?=w523:bool)
                    n391 = Select(t=w521, s=w523, f=w522) -> (s? t:f=w520:dbl)
                    n392 = To Unsigned Byte Integer(number=w520) -> (unsigned 8bit integer=→"1사이클 진행률(%)":u8)
                  }
                }
              }
              event "debug": Value Change {
                n393 = event-data() -> ()  [unwired: 1 in, 6 out]
                n394 = case shown="True" "debug" {
                  tunnel: [enum32{"Main", "debug"}."Main" ("Tab Control_debug") enum32{"Main", "debug"}."debug" ("Tab Control_debug")] -> w541
                  frame False {
                  }
                  frame True {
                  }
                }
                n395 = local write "Tab Control_debug"(w541) -> ()
              }
              event "채널선택": Value Change {
                n396 = event-data() -> ()  [unwired: 1 in, 1 out]
                n397 = Cluster To Array(cluster="채널선택") -> (array=w546:bool[])
                n398 = for {
                  tunnel: [w559] -> w550 mode=indexing if=w558
                  tunnel: w546 -> [w558] mode=indexing
                  i -> [w561]
                  n399 = Increment(x=w561) -> (x+1=w560:i32)
                  n400 = Format Into String(w560) -> (resulting string=w559:string)  [unwired: 3 in, 1 out]
                }
                n401 = Array To Spreadsheet String(delimiter (Tab)=",", array=w550, 3:"" ("format string")) -> (spreadsheet string=w548:string)
                n402 = call "sub_ch-count.vi"("ch config"=w546) -> ("ch num"=w553:u8)  [unwired: 10 in]
                n403 = call <vilib>:"Trim Whitespace.vi"("string"=w548) -> ("trimmed string"=w545:string)  [unwired: 1 in]
                n404 = call "fgv_curr-test-info.vi"("cmd"=rw."read") -> ("현재테스트 정보 2"=w555:T62)  [unwired: 10 in]
                n405 = Bundle By Name(cluster=w555, "전체채널수"=w553, "Ch selection"="채널선택") -> (w554:T62)
                n406 = call "fgv_curr-test-info.vi"("cmd"=rw."write", "현재테스트 정보"=w554) -> ()  [unwired: 9 in, 1 out]
                n407 = call "sub_log_basic.vi"("desc"=w545, "Title"="Channel Activation") -> ()  [unwired: 9 in, 1 out]
              }
              event "HW check": Value Change {
                n408 = event-data() -> ()  [unwired: 1 in, 1 out]
                n409 = call "sub_log_basic.vi"("error in"=w563, "desc"="start", "Title"="HW Check") -> ("error out"=w562:errorcluster)  [unwired: 8 in]
                n410 = call "fgv_stop_local.vi"("cmd"=init-r-stop."ini", "error in (no error)"=w562) -> ("error out"=w566:errorcluster)  [unwired: 8 in, 1 out]
                n411 = stacked-sequence {
                  tunnel: w566 -> [w571 _ _ _ _ _ _]
                  frame #0 {
                    n412 = flat-sequence {
                      tunnel: w571 -> [w572]
                      tunnel: [w572] -> w570
                      frame #0 {
                        n413 = global write "Glob_Ref.vi" "check_hw"(TRUE ("check_hw")) -> ()
                        n414 = Wait (ms)(milliseconds to wait=u32 100) -> ()  [unwired: 1 out]
                      }
                    }
                    n415 = call "fgv_AI_q.vi"("cmd"=create-rw-close."write", "error in"=w570, "data"=start."start") -> ()  [unwired: 7 in, 2 out]
                  }
                  frame #1 {
                    n416 = call "fgv_DL950_q.vi"("cmd"=create-rw-close."write", "data"=start."init") -> ("error out"=w575:errorcluster)  [unwired: 8 in, 1 out]
                    n417 = call "fgv_DL950_q.vi"("cmd"=create-rw-close."write", "error in"=w575, "data"=start."close") -> ()  [unwired: 7 in, 2 out]
                  }
                  frame #2 {
                    n418 = call "fgv_DSP_visa.vi"("action"=DSP_action."cont") -> ("error out"=w582:errorcluster)  [unwired: 10 in]
                    n419 = call "fgv_DSP_visa.vi"("action"=DSP_action."discont", "error in"=w582) -> ()  [unwired: 9 in, 1 out]
                  }
                  frame #3 {
                    n420 = call "fgv_4610_visa.vi"("cmd"=BP4610_cmd."open") -> ("error out"=w585:errorcluster)  [unwired: 10 in]
                    n421 = call "fgv_4610_visa.vi"("cmd"=BP4610_cmd."close", "error in"=w585) -> ()  [unwired: 9 in, 1 out]
                  }
                  frame #4 {
                    n422 = call "fgv_AO_daqmx.vi"("cmd"=init-w-close."open") -> ("error out"=w588:errorcluster)  [unwired: 10 in]
                    n423 = call "fgv_AO_daqmx.vi"("cmd"=init-w-close."close", "error in"=w588) -> ()  [unwired: 9 in, 1 out]
                  }
                  frame #5 {
                    n424 = call "fgv_DO-daqmx.vi"("cnt"=cnt_do."close") -> ("error out"=w589:errorcluster)  [unwired: 10 in]
                    n425 = call "fgv_DO-daqmx.vi"("cnt"=cnt_do."open", "error in"=w589) -> ("error out"=w595:errorcluster)  [unwired: 9 in]
                    n426 = for {
                      tunnel: cluster{"Relay":T49, "Boolean":bool}[] [{"Relay"=enum."R_in1", "Boolean"=FALSE}, {"Relay"=enum."R_in2", "Boolean"=FALSE}, {"Relay"=enum."R_in3", "Boolean"=FALSE}, {"Relay"=enum."R_in4", "Boolean"=FALSE}, {"Relay"=enum."R_in5", "Boolean"=FALSE}, {"Relay"=enum."R_in6", "Boolean"=FALSE}, {"Relay"=enum."R_out1", "Boolean"=FALSE}, {"Relay"=enum."R_out2", "Boolean"=FALSE}, {"Relay"=enum."R_out3", "Boolean"=FALSE}, {"Relay"=enum."R_out4", "Boolean"=FALSE}, {"Relay"=enum."R_out5", "Boolean"=FALSE}, {"Relay"=enum."R_out6", "Boolean"=FALSE}] -> [w599] mode=indexing
                      tunnel: [w597] -> w594
                      tunnel: w595 -> [w596]
                      n427 = call "fgv_DO-daqmx.vi"("cnt"=cnt_do."update", "error in"=w596, "Relay"=w599) -> ("error out"=w597:errorcluster)  [unwired: 8 in]
                    }
                    n428 = call "fgv_DO-daqmx.vi"("cnt"=cnt_do."run", "error in"=w594) -> ()  [unwired: 9 in, 1 out]
                  }
                  frame #6 {
                  }
                }
              }
              event "Apply": Value Change {
                n429 = event-data() -> ()  [unwired: 1 in, 6 out]
                n430 = stacked-sequence {
                  frame #0 {
                    n431 = Unbundle By Name("Testconfig") -> ("Cycle[N]"=w608:u32, "Repeate (Each Ch)"=w607:u32)
                    n432 = call "fgv_rc-config.vi"("cmd"=rw."write", "Testconfig"="Testconfig") -> ()  [unwired: 8 in, 2 out]
                    n433 = call "fgv_rc_breakdonw-specs.vi"("cmd"=rw."write", "BreakdownSpec"="Breakdown-Spec") -> ()  [unwired: 9 in, 1 out]
                    n434 = Bundle By Name(cluster=T41 {"Channel selection"={"1ch"=TRUE, "2ch"=TRUE, "3ch"=TRUE, "4ch"=TRUE, "5ch"=TRUE, "6ch"=TRUE}, "Test Cycle"=1, "Repeate"=1} ("Test Config Common"), "Test Cycle"=w608, "Repeate"=w607) -> (w609:T41)
                    n435 = call "fgv_curr-test-info.vi"("cmd"=rw."read") -> ("현재테스트 정보 2"=w603:T62)  [unwired: 10 in]
                    n436 = Unbundle By Name(w609) -> ("Test Cycle"=w615:u32, "Repeate"=w612:u32)  [unwired: 1 out]
                    n437 = Unbundle By Name(w603) -> ("Ch selection"=w602:T63)
                    n438 = call "fgv_judgement.vi"("cmd"=rw."write", "Test Judgement"="Test Judgement") -> ()  [unwired: 8 in, 2 out]
                    n439 = Cluster To Array(cluster=w602) -> (array=w614:bool[])
                    n440 = call "sub_ch-count.vi"("ch config"=w614) -> ("ch num"=w613:u8)  [unwired: 10 in]
                    n441 = call "fgv_curr-test-info.vi"("cmd"=rw."read") -> ("현재테스트 정보 2"=w617:T62)  [unwired: 10 in]
                    n442 = Bundle By Name(cluster=w617, "전체채널수"=w613, "Ch selection"=w602, "테스트 회수"=w615, "반복"=w612, "Path"="Log path") -> (w616:T62)
                    n443 = call "fgv_curr-test-info.vi"("cmd"=rw."write", "현재테스트 정보"=w616) -> ()  [unwired: 9 in, 1 out]
                  }
                  frame #1 {
                    n444 = call "save_testConditions.vi"("cmd"=cmd_TestParaSave."Save") -> ("error out"=w624:errorcluster)  [unwired: 10 in]
                    n445 = disable-structure shown="Enabled" {
                      disable-tunnel: w624 -> [w627 w629]
                      disable-tunnel: [w626 w629] -> w622
                      frame Disabled {
                        n446 = call "save_testConditions.vi"("error in (no error)"=w627, "cmd"=cmd_TestParaSave."Read") -> ("error out"=w626:errorcluster)  [unwired: 9 in]
                      }
                      frame Enabled {
                      }
                    }
                    n447 = call "UI_result.vi"("result"=result."Init", "error in (no error)"=w622) -> ()  [unwired: 9 in, 1 out]
                  }
                }
              }
              event Value Change {
                n448 = event-data() -> ("OldVal"=w632:T1, "NewVal"=w633:T1)  [unwired: 1 in, 4 out]
                n449 = case shown="\"6.3.2 저온 작동/방치 시험\", Default" 시험모드선택."6.3.2 저온 작동/방치 시험" ("시험모드 선택") {
                  tunnel: w633 -> [_ w637]
                  tunnel: "ES 규격시험 선택" -> [_ w636]
                  tunnel: w632 -> [w635 _]
                  frame "6.3.1 온도방치 시험", "6.3.7 고온고습 방치", "6.3.11.1 작동가진".."6.3.12 충격시험" {
                    n450 = local write "ES 규격시험 선택"(w635) -> ()
                    n451 = One Button Dialog(message="기능 업데이트 예정입니다.") -> ()  [unwired: 1 in, 1 out]
                  }
                  frame "6.3.2 저온 작동/방치 시험", Default {
                    n452 = stacked-sequence {
                      tunnel: w637 -> [_ _ _ w664 _ _]
                      tunnel: w636 -> [_ w639 w652 _ _ _]
                      frame #0 {
                        n453 = local write "Log path"(path "C:/Users/abc/Desktop/데이터저장" ("Log path")) -> ()
                      }
                      frame #1 {
                        n454 = global read "Global 1.vi" "시험 모드"() -> (w641:T4)
                        n455 = case shown="\"고전압모드 동작검사\"" w641 {
                          tunnel: [T24 {"제어단 단선 Irms[mA](이하)"=5.0, "제어단 특성 전류 Irms[mA] Max"=25.0, "제어단 특성 전류 Irms[mA] Min"=15.0, "출력단 단선 Irms[mA](이하)"=5.0, "출력단 특성 전류 Irms[mA]  Max"=13.0, "출력단 특성전류 Irms[mA]  Min"=9.0, "온도[degree]"=60.0} ("Breakdown-Spec") T24 {"제어단 단선 Irms[mA](이하)"=5.0, "제어단 특성 전류 Irms[mA] Max"=25.0, "제어단 특성 전류 Irms[mA] Min"=15.0, "출력단 단선 Irms[mA](이하)"=5.0, "출력단 특성 전류 Irms[mA]  Max"=1100.0, "출력단 특성전류 Irms[mA]  Min"=900.0, "온도[degree]"=60.0} ("Breakdown-Spec") w649] -> w642
                          tunnel: ["저전압모드 동작검사" ("시험명") "저전압모드 접촉저항" ("시험명") "고전압모드 동작검사" ("시험명")] -> w640
                          tunnel: w639 -> [_ _ w647]
                          frame "저전압모드 동작검사", Default {
                          }
                          frame "저전압모드 접촉저항" {
                          }
                          frame "고전압모드 동작검사" {
                            n456 = case shown="\"6.3.3 고온 작동/방치 시험\", Default" w647 {
                              tunnel: [T24 {"제어단 단선 Irms[mA](이하)"=5.0, "제어단 특성 전류 Irms[mA] Max"=25.0, "제어단 특성 전류 Irms[mA] Min"=15.0, "출력단 단선 Irms[mA](이하)"=5.0, "출력단 특성 전류 Irms[mA]  Max"=4000.0, "출력단 특성전류 Irms[mA]  Min"=3000.0, "온도[degree]"=60.0} ("Breakdown-Spec") T24 {"제어단 단선 Irms[mA](이하)"=5.0, "제어단 특성 전류 Irms[mA] Max"=25.0, "제어단 특성 전류 Irms[mA] Min"=15.0, "출력단 단선 Irms[mA](이하)"=5.0, "출력단 특성 전류 Irms[mA]  Max"=800.0, "출력단 특성전류 Irms[mA]  Min"=600.0, "온도[degree]"=60.0} ("Breakdown-Spec")] -> w649
                              frame "6.3.3 고온 작동/방치 시험", Default {
                              }
                              frame "6.3.9 빙결시험" {
                              }
                            }
                          }
                        }
                        n457 = local write "Breakdown-Spec"(w642) -> ()
                        n458 = local write "시험명"(w640) -> ()
                      }
                      frame #2 {
                        n459 = global read "Global 1.vi" "시험 모드"() -> (w654:T4)
                        n460 = case shown="\"저전압모드 접촉저항\"" w654 {
                          tunnel: [T25 {"전압 63%[mS] Min"=0.0, "전압 98%[mS] Min"=0.0, "전류 37%[mS] Min"=0.0, "접촉저항[mOhm] Min"=0.0, "출력전류 Irms[mA] Min"=9.0, "전압 63%[mS] Max"=0.0, "전압 98%[mS] Max"=0.0, "전류 37%[mS] Max"=0.0, "접촉저항[mOhm] Max"=0.0, "출력전류 Irms[mA] Max"=13.0} ("Test Judgement") T25 {"전압 63%[mS] Min"=0.0, "전압 98%[mS] Min"=0.0, "전류 37%[mS] Min"=0.0, "접촉저항[mOhm] Min"=600.0, "출력전류 Irms[mA] Min"=0.0, "전압 63%[mS] Max"=0.0, "전압 98%[mS] Max"=0.0, "전류 37%[mS] Max"=0.0, "접촉저항[mOhm] Max"=900.0, "출력전류 Irms[mA] Max"=0.0} ("Test Judgement") w658] -> w653
                          tunnel: w652 -> [_ _ w657]
                          frame "저전압모드 동작검사", Default {
                          }
                          frame "저전압모드 접촉저항" {
                          }
                          frame "고전압모드 동작검사" {
                            n461 = case shown="\"6.3.3 고온 작동/방치 시험\", Default" w657 {
                              tunnel: [T25 {"전압 63%[mS] Min"=34.0, "전압 98%[mS] Min"=130.0, "전류 37%[mS] Min"=34.0, "접촉저항[mOhm] Min"=200.0, "출력전류 Irms[mA] Min"=3000.0, "전압 63%[mS] Max"=40.0, "전압 98%[mS] Max"=145.0, "전류 37%[mS] Max"=40.0, "접촉저항[mOhm] Max"=400.0, "출력전류 Irms[mA] Max"=4000.0} ("Test Judgement") T25 {"전압 63%[mS] Min"=34.0, "전압 98%[mS] Min"=135.0, "전류 37%[mS] Min"=34.0, "접촉저항[mOhm] Min"=200.0, "출력전류 Irms[mA] Min"=600.0, "전압 63%[mS] Max"=40.0, "전압 98%[mS] Max"=155.0, "전류 37%[mS] Max"=40.0, "접촉저항[mOhm] Max"=400.0, "출력전류 Irms[mA] Max"=800.0} ("Test Judgement")] -> w658
                              frame "6.3.3 고온 작동/방치 시험", Default {
                              }
                              frame "6.3.9 빙결시험" {
                              }
                            }
                          }
                        }
                        n462 = local write "Test Judgement"(w653) -> ()
                      }
                      frame #3 {
                        (unwired) "작동시간(초)" ("Label.Text")
                        n463 = case shown="\"6.3.1 온도방치 시험\"" w664 {
                          tunnel: [T53."6.3.9 빙결 시험" ("Test Mode") T53."6.3.2 저온 작동/방치 시험" ("Test Mode") T53."6.3.3 고온 작동/방치 시험" ("Test Mode") T53."6.3.4 온도 싸이클 시험" ("Test Mode") T53."6.3.6 온습도 싸이클 시험" ("Test Mode") T53."6.3.6 온습도 싸이클 시험" ("Test Mode") T53."6.3.8 결로 시험" ("Test Mode") T53."6.3.9 빙결 시험" ("Test Mode")] -> _
                          tunnel: ["작동시간(초)" ("Label.Text") "작동시간(초)" ("Label.Text") "작동시간(초)" ("Label.Text") "작동시간(초)" ("Label.Text") "작동시간(초)" ("Label.Text") "작동시간(초)" ("Label.Text") "작동시간(초)" ("Label.Text") "작동시간(초)" ("Label.Text")] -> w662
                          frame "6.3.1 온도방치 시험" {
                          }
                          frame "6.3.2 저온 작동/방치 시험", Default {
                          }
                          frame "6.3.3 고온 작동/방치 시험" {
                          }
                          frame "6.3.4 온도 싸이클 시험" {
                          }
                          frame "6.3.6 온습도 싸이클 시험" {
                          }
                          frame "6.3.7 고온고습 방치" {
                          }
                          frame "6.3.8 결로 시험" {
                          }
                          frame "6.3.9 빙결시험" {
                          }
                        }
                        n464 = global read "Global 1.vi" "작동시간(초)"() -> (w663:refnum<vi>)
                        n465 = call "TestModeUpdate.vi"("Update?"=TRUE) -> ()  [unwired: 9 in, 2 out]
                        n466 = property class="DigNum (strict)"(reference=w663, "Caption.Text"=w662) -> ()  [unwired: 1 in, 2 out]
                      }
                      frame #4 {
                        n467 = local read "Testconfig"() -> (w684:T19)
                        n468 = local read "Breakdown-Spec"() -> (w683:T24)
                        n469 = Unbundle By Name(w684) -> ("Cycle[N]"=w690:u32, "Repeate (Each Ch)"=w689:u32)
                        n470 = call "fgv_rc_breakdonw-specs.vi"("cmd"=rw."write", "BreakdownSpec"=w683) -> ()  [unwired: 9 in, 1 out]
                        n471 = Bundle By Name(cluster=T41 {"Channel selection"={"1ch"=TRUE, "2ch"=TRUE, "3ch"=TRUE, "4ch"=TRUE, "5ch"=TRUE, "6ch"=TRUE}, "Test Cycle"=1, "Repeate"=1} ("Test Config Common"), "Test Cycle"=w690, "Repeate"=w689) -> (w691:T41)
                        n472 = local read "Test Judgement"() -> (w682:T25)
                        n473 = call "fgv_curr-test-info.vi"("cmd"=rw."read") -> ("현재테스트 정보 2"=w686:T62)  [unwired: 10 in]
                        n474 = Unbundle By Name(w686) -> ("Ch selection"=w685:T63)
                        n475 = Unbundle By Name(w691) -> ("Test Cycle"=w696:u32, "Repeate"=w693:u32)  [unwired: 1 out]
                        n476 = call "fgv_judgement.vi"("cmd"=rw."write", "Test Judgement"=w682) -> ()  [unwired: 8 in, 2 out]
                        n477 = Cluster To Array(cluster=w685) -> (array=w695:bool[])
                        n478 = local read "Log path"() -> (w681:path)
                        n479 = call "sub_ch-count.vi"("ch config"=w695) -> ("ch num"=w694:u8)  [unwired: 10 in]
                        n480 = call "fgv_curr-test-info.vi"("cmd"=rw."read") -> ("현재테스트 정보 2"=w698:T62)  [unwired: 10 in]
                        n481 = Bundle By Name(cluster=w698, "전체채널수"=w694, "Ch selection"=w685, "테스트 회수"=w696, "반복"=w693, "Path"=w681) -> (w697:T62)
                        n482 = call "fgv_curr-test-info.vi"("cmd"=rw."write", "현재테스트 정보"=w697) -> ()  [unwired: 9 in, 1 out]
                      }
                      frame #5 {
                        n483 = call "save_testConditions.vi"("cmd"=cmd_TestParaSave."Save") -> ("error out"=w704:errorcluster)  [unwired: 10 in]
                        n484 = call "save_testConditions.vi"("error in (no error)"=w704, "cmd"=cmd_TestParaSave."Read") -> ("error out"=w702:errorcluster)  [unwired: 9 in]
                        n485 = call "UI_result.vi"("result"=result."Init", "error in (no error)"=w702) -> ()  [unwired: 9 in, 1 out]
                      }
                    }
                  }
                }
              }
              event Value Change {
                n486 = event-data() -> ()  [unwired: 1 in, 6 out]
                n487 = call "TestModeUpdate.vi"("Update?"=TRUE) -> ()  [unwired: 9 in, 2 out]
              }
              event "시험규격": Value Change {
                n488 = event-data() -> ()  [unwired: 1 in, 6 out]
                n489 = call "Set_TestMode.vi"() -> ()  [unwired: 11 in, 1 out]
              }
              event "copy", "paste": Value Change {
                n490 = event-data() -> ("CtlRef"=w709:refnum<vi>)  [unwired: 1 in, 5 out]
                n491 = property class="Bool"(reference=w709) -> ("Label.Text"=w708:string)  [unwired: 1 in, 2 out]
                n492 = case shown="\"copy\"" w708 {
                  frame "paste", Default {
                    n493 = global read "Glob_setting.vi" "Breakdown-Spec"() -> (w712:T24)
                    n494 = global read "Glob_setting.vi" "Test Judgement"() -> (w711:T25)
                    n495 = global read "Glob_setting.vi" "Testconfig"() -> (w710:T19)
                    n496 = local write "Breakdown-Spec"(w712) -> ()
                    n497 = local write "Test Judgement"(w711) -> ()
                    n498 = local write "Testconfig"(w710) -> ()
                  }
                  frame "copy" {
                    n499 = local read "Breakdown-Spec"() -> (w715:T24)
                    n500 = local read "Test Judgement"() -> (w714:T25)
                    n501 = local read "Testconfig"() -> (w713:T19)
                    n502 = global write "Glob_setting.vi" "Breakdown-Spec"(w715) -> ()
                    n503 = global write "Glob_setting.vi" "Test Judgement"(w714) -> ()
                    n504 = global write "Glob_setting.vi" "Testconfig"(w713) -> ()
                  }
                }
              }
              event Value Change {
                n505 = event-data() -> ()  [unwired: 1 in, 6 out]
                n506 = stacked-sequence {
                  seq-local: [_ "시험 모드" _ _] -> [_ _ w719 _]
                  seq-local: [_ _ w719 _] -> [_ _ _ w724]
                  seq-local: [_ _ w718 _] -> [_ _ _ w723]
                  frame #0 {
                    n507 = call "fgv_DL950_visa.vi"("cmd"=fgv_DL950."offset cancel") -> ()  [unwired: 8 in, 3 out]
                  }
                  frame #1 {
                    n508 = global write "Global 1.vi" "시험 모드"("시험 모드") -> ()
                  }
                  frame #2 {
                    n509 = local read "Tab_menu-select"() -> (w718:T7)
                    n510 = call "TableCnt.vi"("cnt"=cmd_tablecnt."Inital") -> ()  [unwired: 9 in, 2 out]
                    n511 = call "save_testConditions.vi"("cmd"=cmd_TestParaSave."Read") -> ()  [unwired: 10 in, 1 out]
                  }
                  frame #3 {
                    n512 = case shown="\"Setting\"" w723 {
                      tunnel: w724 -> [_ w725]
                      frame "Manual", Default {
                      }
                      frame "Setting" {
                        n513 = call "setting cable.vi"("시험 모드"=w725) -> ()  [unwired: 10 in, 1 out]
                      }
                    }
                    n514 = call "UI_result.vi"("result"=result."Init") -> ()  [unwired: 10 in, 1 out]
                  }
                }
              }
              event "시험환경세팅": Value Change {
                n515 = event-data() -> ()  [unwired: 1 in, 6 out]
                n516 = global read "Global 1.vi" "시험 모드"() -> (w726:T4)
                n517 = call "setting cable.vi"("시험 모드"=w726) -> ()  [unwired: 10 in, 1 out]
              }
              event "RCstart", "Rloadstart", "B1start", "B2start", "B3start": Value Change {
                n518 = event-data() -> ()  [unwired: 1 in, 1 out]
                n519 = case shown="\"6.3.1 온도방치 시험\", \"6.3.7 고온고습 방치\", \"6.3.11.1 작동가진\"..\"6.3.12 충격시험\"" 시험모드선택."6.3.8 결로 시험" ("ES 규격시험 선택") {
                  frame "6.3.1 온도방치 시험", "6.3.7 고온고습 방치", "6.3.11.1 작동가진".."6.3.12 충격시험" {
                    n520 = property on="RCstart" class="Bool"("DisabledEnum"=T2."Disabled and Grayed Out" ("Disabled")) -> ()  [unwired: 2 in, 2 out]
                    n521 = One Button Dialog(message="기능 업데이트 예정입니다.") -> ()  [unwired: 1 in, 1 out]
                  }
                  frame "6.3.2 저온 작동/방치 시험", Default {
                    n522 = stacked-sequence {
                      frame #0 {
                        n523 = local read "Breakdown-Spec"() -> (w743:T24)
                        n524 = local read "Test Judgement"() -> (w744:T25)
                        n525 = call "fgv_rc_breakdonw-specs.vi"("cmd"=rw."write", "BreakdownSpec"=w743) -> ()  [unwired: 9 in, 1 out]
                        n526 = call "fgv_judgement.vi"("cmd"=rw."write", "Test Judgement"=w744) -> ()  [unwired: 8 in, 2 out]
                        n527 = call "fgv_UI-dev-operator.vi"("cmd"=UI_dev-operator."Testing") -> ()  [unwired: 10 in, 1 out]
                        n528 = local read "Testconfig"() -> (w742:T19)
                        n529 = call "fgv_rc-config.vi"("cmd"=rw."write", "Testconfig"=w742) -> ("Testconfig out"=w734:T19)  [unwired: 8 in, 1 out]
                        n530 = Unbundle By Name(w734) -> ("Cycle[N]"=w733:u32, "Repeate (Each Ch)"=w732:u32)
                        n531 = local read "Log path"() -> (w730:path)
                        n532 = call "fgv_curr-test-info.vi"("cmd"=rw."read") -> ("현재테스트 정보 2"=w736:T62)  [unwired: 10 in]
                        n533 = Bundle By Name(cluster=w736, "테스트 회수"=w733, "반복"=w732, "Path"=w730) -> (w735:T62)
                        n534 = call "fgv_curr-test-info.vi"("cmd"=rw."write", "현재테스트 정보"=w735) -> ()  [unwired: 9 in, 1 out]
                      }
                      frame #1 {
                        n535 = call "sub_hw-set.vi"("cmd"=hw-control."relay all-off") -> ("error out"=w755:errorcluster)  [unwired: 10 in]
                        n536 = call "sub_test-start-check.vi"("error in"=w755) -> ("error out"=w752:errorcluster)  [unwired: 10 in]
                        n537 = call "Timer.vi"("cmd"=cmd_timer."init") -> ()  [unwired: 8 in, 3 out]
                        n538 = Format Date/Time String(time format string (%c)="%Y-%m-%d \n%H:%M:%S" ("시간 포맷 문자열 (%c)")) -> (date/time string=→"시작시간":string)  [unwired: 2 in]
                        n539 = call "sub_ui-usertype.vi"("Disabled"=T2."Disabled and Grayed Out") -> ()  [unwired: 11 in]
                        n540 = call "sub_log-header-write.vi"("cmd"=log_save_type."header", "error in (no error)"=w752, "시험명"="시험명") -> ()  [unwired: 8 in, 1 out]
                        n541 = call "TableCnt.vi"("cnt"=cmd_tablecnt."Inital") -> ()  [unwired: 9 in, 2 out]
                        n542 = call "UI_result.vi"("result"=result."Init") -> ()  [unwired: 10 in, 1 out]
                        n543 = property on="RCstart" class="Bool"("DisabledEnum"=T2."Enabled" ("Disabled")) -> ()  [unwired: 2 in, 2 out]
                        n544 = call "fgv_error_rc.vi"("cmd"=init-r-w."init") -> ()  [unwired: 10 in, 1 out]
                        "종료시간" <- "" ("종료시간")
                      }
                    }
                  }
                }
              }
              event "login", "logout": Value Change {
                n545 = event-data() -> ("CtlRef"=w761:refnum<vi>)  [unwired: 1 in, 5 out]
                n546 = property class="Bool"(reference=w761) -> ("Label.Text"=w760:string)  [unwired: 1 in, 2 out]
                n547 = case shown="\"login\"" w760 {
                  tunnel: "Password" -> [_ w765]
                  frame "False", Default {
                    n548 = local write "Password"("" ("Password")) -> ()
                    n549 = call "sub_ui-usertype.vi"("Disabled"=T2."Disabled and Grayed Out") -> ()  [unwired: 11 in]
                  }
                  frame "login" {
                    n550 = Equal?(x=w765, y="admin") -> (x = y?=w768:bool)
                    n551 = Equal?(x=w765, y="yko") -> (x = y?=w764:bool)
                    n552 = Compound Arithmetic op=OR(w768, w764) -> (w767:bool)
                    n553 = case shown="True" w767 {
                      frame False {
                        n554 = call "sub_ui-usertype.vi"("Disabled"=T2."Disabled and Grayed Out") -> ()  [unwired: 11 in]
                      }
                      frame True {
                        n555 = call "sub_ui-usertype.vi"("Disabled"=T2."Enabled") -> ()  [unwired: 11 in]
                      }
                    }
                  }
                }
              }
              event "\"시험모드\" 파일이름 생성 무시(Ignore)": Value Change {
                n556 = event-data() -> ()  [unwired: 1 in, 6 out]
                n557 = global write "Glob_setting.vi" "무시(Ignore)"("\"시험모드\" 파일이름 생성 무시(Ignore)") -> ()
              }
              event "Apply AO", "Ouptut_NIAO", "AO_Level", "AO": Value Change {
                n558 = event-data() -> ("CtlRef"=w785:refnum<vi>)  [unwired: 1 in]
                n559 = local read "AO_Wave-config"() -> (w775:T14)
                n560 = call "fgv_AO_wave-config.vi"("cmd"=rw."write", "Square Wave"=w775) -> ("error out"=w773:errorcluster)  [unwired: 8 in, 1 out]
                n561 = property class="Ctl"(reference=w785) -> ("Label.Text"=w786:string)  [unwired: 1 in, 2 out]
                n562 = call "fgv_AO_daqmx.vi"("cmd"=init-w-close."open") -> ("error out"=w778:errorcluster)  [unwired: 10 in]
                n563 = call "fgv_status-display.vi"("Mode"=system-status."Clear") -> ("error out"=w781:errorcluster)  [unwired: 10 in]
                n564 = call "fgv_AO_wave-config.vi"("cmd"=rw."read", "error in (no error)"=w773) -> ("Square Wave 2"=w783:T14)  [unwired: 8 in, 1 out]
                n565 = case shown="\"AO\"" w786 {
                  tunnel: w783 -> [_ w789 w793 w804]
                  tunnel: w781 -> [_ _ _ _]
                  tunnel: "AO" -> [_ _ _ w803]
                  tunnel: w778 -> [w787 w788 w791 w795]
                  tunnel: [w787 w788 w790 w796] -> w776
                  frame "False", Default {
                  }
                  frame "Apply AO" {
                    n566 = call "Graph_AO.vi"("Square Wave"=w789) -> ()  [unwired: 10 in, 1 out]
                  }
                  frame "Ouptut_NIAO" {
                    n567 = call "signalGenerator.vi"("cnt"=type_signal."wave", "Square Wave"=w793) -> ()  [unwired: 8 in, 2 out]
                    n568 = call "sub_AO-gen.vi"("error in (no error)"=w791) -> ("error out"=w790:errorcluster)  [unwired: 10 in]
                  }
                  frame "AO" {
                    n569 = Select(t="AO_Level", s=w803, f=0.0) -> (s? t:f=w799:dbl)
                    n570 = Bundle By Name(cluster=w804, "wfm.Amp"=w799) -> (w801:T14)
                    n571 = call "signalGenerator.vi"("error in"=w795, "cnt"=type_signal."level", "Square Wave"=w801) -> ("error out"=w797:errorcluster)  [unwired: 7 in, 1 out]
                    n572 = call "sub_AO-gen.vi"("error in (no error)"=w797, "level"=TRUE) -> ("error out"=w796:errorcluster)  [unwired: 9 in]
                  }
                }
                n573 = call "fgv_AO_daqmx.vi"("cmd"=init-w-close."close", "error in"=w776) -> ()  [unwired: 9 in, 1 out]
              }
              event "single start": Value Change {
                n574 = event-data() -> ()  [unwired: 1 in, 1 out]
                n575 = flat-sequence {
                  frame #0 {
                    n576 = call "fgv_stop_local.vi"("cmd"=init-r-stop."ini") -> ()  [unwired: 9 in, 2 out]
                    n577 = call "fgv_status-display.vi"("Mode"=system-status."Clear") -> ()  [unwired: 10 in, 1 out]
                    n578 = call "sub_hw-set.vi"("cmd"=hw-control."relay all-off") -> ()  [unwired: 10 in, 1 out]
                  }
                  frame #1 {
                    n579 = call "fgv_curr-test-info.vi"("cmd"=rw."read") -> ("현재테스트 정보 2"=w811:T62)  [unwired: 10 in]
                    n580 = Bundle By Name(cluster=w811, "테스트 회수"=u32 1) -> (w809:T62)
                    n581 = Unbundle By Name(w811) -> ("Ch selection"=w817:T63)
                    n582 = call "fgv_error_rc.vi"("cmd"=init-r-w."init") -> ()  [unwired: 10 in, 1 out]
                    n583 = Cluster To Array(cluster=w817) -> (array=w816:bool[])
                    n584 = call "fgv_curr-test-info.vi"("cmd"=rw."write", "현재테스트 정보"=w809) -> ()  [unwired: 9 in, 1 out]
                    n585 = call "UI_result.vi"("result"=result."Init") -> ()  [unwired: 10 in, 1 out]
                    n586 = Boolean Array To Number(Boolean array=w816) -> (number=w815:u32)
                    n587 = Equal To 0?(x=w815) -> (x = 0?=w814:bool)
                    n588 = case shown="False" w814 {
                      frame False {
                        n589 = global write "Glob_Ref.vi" "Single sequence"("Single sequence") -> ()
                        n590 = call "sub_single-cycle-config.vi"("Single sequence"="Single sequence") -> ()  [unwired: 11 in]
                        n591 = call "fgv_single-sequence.vi"("cmd"=create-rw-close."write", "Single sequence"="Single sequence") -> ()  [unwired: 8 in, 2 out]
                      }
                      frame True {
                        n592 = One Button Dialog(message="채널이 선택되지 않았습니다.", button name ("OK")="채널을 선택해 주세요") -> ()  [unwired: 1 out]
                      }
                    }
                  }
                }
              }
              event "Read": Value Change {
                n593 = event-data() -> ()  [unwired: 1 in, 1 out]
                n594 = Tick Count (ms)() -> (millisecond timer value=w823:u32)
                n595 = stacked-sequence {
                  seq-local: [_ _ _ _ _ w835 _ _ _ _ _ _ _ _] -> [_ _ _ _ _ _ _ _ _ _ _ _ _ w858]
                  seq-local: [_ _ _ _ _ _ _ _ w843 _ _ _ _ _] -> [_ _ _ _ _ _ _ _ _ _ _ _ _ w857]
                  tunnel: w823 -> [_ _ _ _ _ _ _ _ _ _ _ _ _ w853]
                  frame #0 {
                    n596 = disable-structure shown="Disabled" {
                      frame Disabled {
                        n597 = global write "Global 1.vi" "String"(":MEASURE:CHANNEL2:DPROXIMAL:PERCENT 0,30,63\n:MEASURE:CHANNEL6:DPROXIMAL:PERCENT 37,50,100" ("String")) -> ()
                      }
                      frame Enabled {
                      }
                    }
                  }
                  frame #1 {
                    n598 = disable-structure shown="Disabled" {
                      frame Disabled {
                        n599 = call "fgv_DL950_q.vi"("cmd"=create-rw-close."write", "data"=start."query") -> ()  [unwired: 8 in, 2 out]
                        n600 = Wait (ms)(milliseconds to wait=u32 2000) -> ()  [unwired: 1 out]
                      }
                      frame Enabled {
                      }
                    }
                  }
                  frame #2 {
                    n601 = global write "Global 1.vi" "query delay"(u32 100 ("query delay")) -> ()
                    n602 = global write "Global 1.vi" "String"(":TRIGGER:POSITION?\n:TIMebase:TDIV?\n:MEASURE:CHANNEL2:RISE:VALUE?\n:MEASURE:CHANNEL6:FALL:VALUE?\n:MEASURE:TRANGE -5,5\n:MEASURE:CHANNEL5:RMS:VALUE?\n:MEASURE:CHANNEL6:RMS:VALUE?" ("String")) -> ()
                  }
                  frame #3 {
                    n603 = call "fgv_DL950_q.vi"("cmd"=create-rw-close."write", "data"=start."query") -> ()  [unwired: 8 in, 2 out]
                    n604 = Wait (ms)(milliseconds to wait=u32 100) -> ()  [unwired: 1 out]
                  }
                  frame #4 {
                    n605 = call "sub_query_donCheck.vi"() -> ()  [unwired: 3 in, 1 out]
                  }
                  frame #5 {
                    n606 = call "TrangeCalc.vi"() -> ("T2"=w837:dbl, "T1"=w838:dbl, "array"=w835:dbl[])  [unwired: 7 in, 1 out]
                    n607 = Format Into String(format string=":MEASURE:TRANGE %#_g,%#_g\n:MEASURE:CHANNEL3:MAXimum:VALUE?\n:MEASURE:CHANNEL4:MAXimum:VALUE?\n:MEASURE:CHANNEL6:RMS:VALUE?\n:MEASURE:TRANGE -4.2,0", w838, w837) -> (resulting string=w834:string)  [unwired: 2 in, 1 out]
                    n608 = global write "Global 1.vi" "query delay"(u32 100 ("query delay")) -> ()
                    n609 = global write "Global 1.vi" "String"(w834) -> ()
                  }
                  frame #6 {
                    n610 = call "fgv_DL950_q.vi"("cmd"=create-rw-close."write", "data"=start."query") -> ()  [unwired: 8 in, 2 out]
                    n611 = Wait (ms)(milliseconds to wait=u32 100) -> ()  [unwired: 1 out]
                  }
                  frame #7 {
                    n612 = call "sub_query_donCheck.vi"() -> ()  [unwired: 3 in, 1 out]
                  }
                  frame #8 {
                    n613 = call "TrangeCalc.vi"() -> ("array"=w843:dbl[])  [unwired: 7 in, 3 out]
                    n614 = global write "Global 1.vi" "String"(":MEASURE:CHANNEL2:DPROXIMAL:PERCENT 0,50,98" ("format string")) -> ()
                  }
                  frame #9 {
                    n615 = call "fgv_DL950_q.vi"("cmd"=create-rw-close."write", "data"=start."query") -> ()  [unwired: 8 in, 2 out]
                    n616 = Wait (ms)(milliseconds to wait=u32 2500) -> ()  [unwired: 1 out]
                  }
                  frame #10 {
                    n617 = global write "Global 1.vi" "query delay"(u32 100 ("query delay")) -> ()
                    n618 = global write "Global 1.vi" "String"(":MEASURE:CHANNEL2:RISE:VALUE?" ("format string")) -> ()
                  }
                  frame #11 {
                    n619 = call "fgv_DL950_q.vi"("cmd"=create-rw-close."write", "data"=start."query") -> ()  [unwired: 8 in, 2 out]
                    n620 = Wait (ms)(milliseconds to wait=u32 100) -> ()  [unwired: 1 out]
                  }
                  frame #12 {
                    n621 = call "sub_query_donCheck.vi"() -> ()  [unwired: 3 in, 1 out]
                  }
                  frame #13 {
                    n622 = Tick Count (ms)() -> (millisecond timer value=w854:u32)
                    n623 = Subtract(x=w854, y=w853) -> (x-y=→"Time":u32)
                    n624 = call "TrangeCalc.vi"() -> ("array"=w856:dbl[])  [unwired: 7 in, 3 out]
                    n625 = Build Array (concatenate)(w858, w857, w856) -> (→"DL950 read":dbl[])
                  }
                }
              }
              event Value Change {
                n626 = event-data() -> ()  [unwired: 1 in, 1 out]
                n627 = call "fgv_AO_wave-config.vi"("cmd"=rw."write", "Square Wave"="AO_Wave-config") -> ()  [unwired: 8 in, 2 out]
              }
              event Value Change {
                n628 = event-data() -> ()  [unwired: 1 in, 1 out]
                n629 = call "fgv_AO_DAQmx-Config.vi"("cmd"=rw."write", "9269 AO Config"="cDAQ 9269 AO config") -> ()  [unwired: 8 in, 2 out]
              }
              event "Read_AI", "Stop_AI": Value Change {
                n630 = event-data() -> ("CtlRef"=w864:refnum<vi>)  [unwired: 1 in]
                n631 = property class="Bool"(reference=w864) -> ("Label.Text"=w863:string)  [unwired: 1 in, 2 out]
                n632 = case shown="\"Read_AI\"" w863 {
                  frame "False", Default {
                  }
                  frame "Read_AI" {
                    n633 = flat-sequence {
                      frame #0 {
                        n634 = call "fgv_status-display.vi"("Mode"=system-status."Clear") -> ()  [unwired: 10 in, 1 out]
                      }
                      frame #1 {
                        n635 = call "fgv_stop_local.vi"("cmd"=init-r-stop."ini") -> ()  [unwired: 9 in, 2 out]
                      }
                      frame #2 {
                        n636 = call "fgv_AI_q.vi"("cmd"=create-rw-close."write", "data"=start."start") -> ()  [unwired: 8 in, 2 out]
                      }
                    }
                  }
                  frame "Stop_AI" {
                    n637 = call "fgv_stop_local.vi"("cmd"=init-r-stop."stop") -> ()  [unwired: 9 in, 2 out]
                  }
                }
              }
              event Value Change {
                n638 = event-data() -> ()  [unwired: 1 in, 1 out]
                n639 = call "fgv_9221-config.vi"("cmd"=rw."write", "cDAQ 9221 Config"="cDAQ 9221 Config") -> ()  [unwired: 8 in, 2 out]
              }
              event "DO Initialize": Value Change {
                n640 = event-data() -> ()  [unwired: 1 in, 1 out]
                n641 = stacked-sequence {
                  frame #0 {
                    n642 = call "fgv_status-display.vi"("Mode"=system-status."Clear") -> ()  [unwired: 10 in, 1 out]
                  }
                  frame #1 {
                    n643 = global write "Global 1.vi" "lines_do"("cDAQ-9467 Config") -> ()
                    n644 = call "fgv_9467_Config.vi"("cmd"=rw."write", "cDAQ-9467 Config"="cDAQ-9467 Config") -> ()  [unwired: 9 in, 1 out]
                  }
                  frame #2 {
                    n645 = call "fgv_DO-daqmx.vi"("cnt"=cnt_do."close") -> ("error out"=w881:errorcluster)  [unwired: 10 in]
                    n646 = call "fgv_DO-daqmx.vi"("cnt"=cnt_do."open", "error in"=w881) -> ("error out"=w879:errorcluster)  [unwired: 9 in]
                    n647 = for {
                      tunnel: cluster{"Relay":T49, "Boolean":bool}[] [{"Relay"=enum."R_in1", "Boolean"=FALSE}, {"Relay"=enum."R_in2", "Boolean"=FALSE}, {"Relay"=enum."R_in3", "Boolean"=FALSE}, {"Relay"=enum."R_in4", "Boolean"=FALSE}, {"Relay"=enum."R_in5", "Boolean"=FALSE}, {"Relay"=enum."R_in6", "Boolean"=FALSE}, {"Relay"=enum."R_out1", "Boolean"=FALSE}, {"Relay"=enum."R_out2", "Boolean"=FALSE}, {"Relay"=enum."R_out3", "Boolean"=FALSE}, {"Relay"=enum."R_out4", "Boolean"=FALSE}, {"Relay"=enum."R_out5", "Boolean"=FALSE}, {"Relay"=enum."R_out6", "Boolean"=FALSE}] -> [w885] mode=indexing
                      tunnel: [w883] -> w880
                      tunnel: w879 -> [w882]
                      n648 = call "fgv_DO-daqmx.vi"("cnt"=cnt_do."update", "error in"=w882, "Relay"=w885) -> ("error out"=w883:errorcluster)  [unwired: 8 in]
                    }
                    n649 = call "fgv_DO-daqmx.vi"("cnt"=cnt_do."run", "error in"=w880) -> ()  [unwired: 9 in, 1 out]
                  }
                }
              }
              event "Graph": Value Change {
                n650 = event-data() -> ()  [unwired: 1 in, 1 out]
                n651 = call "GraphView_Read.vi"() -> ()  [unwired: 11 in, 1 out]
              }
              event "저항부하", "캐패시터부하", "B-수명 1", "B-수명 2", "B-수명 3": Value Change {
                n652 = event-data() -> ("CtlRef"=w887:refnum<vi>)  [unwired: 1 in]
                n653 = property class="Bool"(reference=w887) -> ("Label.Text"=w886:string)  [unwired: 1 in, 2 out]
                n654 = case shown="\"B-수명 3\"" w886 {
                  frame "False", Default {
                  }
                  frame "저항부하" {
                    n655 = call "fgv_Main_q.vi"("cmd"=create-rw-close."write", "data"=fgv_Main_q."R") -> ()  [unwired: 8 in, 2 out]
                  }
                  frame "캐패시터부하" {
                    n656 = call "fgv_Main_q.vi"("cmd"=create-rw-close."write", "data"=fgv_Main_q."RC") -> ()  [unwired: 8 in, 2 out]
                  }
                  frame "B-수명 1" {
                    n657 = call "fgv_Main_q.vi"("cmd"=create-rw-close."write", "data"=fgv_Main_q."B1") -> ()  [unwired: 8 in, 2 out]
                  }
                  frame "B-수명 2" {
                    n658 = call "fgv_Main_q.vi"("cmd"=create-rw-close."write", "data"=fgv_Main_q."B2") -> ()  [unwired: 8 in, 2 out]
                  }
                  frame "B-수명 3" {
                    n659 = call "fgv_Main_q.vi"("cmd"=create-rw-close."write", "data"=fgv_Main_q."B3") -> ()  [unwired: 8 in, 2 out]
                  }
                }
              }
              event "PinR 2", "PinR 3", "PinR 4", "PinR 5", "PinR 6", "PoutR 1", "PoutR 2", "PoutR 3", "PoutR 4", "PoutR 5", "PoutR 6", "PinR 1", "led red", "led yellow", "led green", "led buz", "led purple", "Discharge R": Value Change {
                w899 = T48[] [enum."update", enum."run"] items=["open", "initial", "update", "run", "close"]
                n660 = event-data() -> ("CtlRef"=w901:refnum<vi>)  [unwired: 1 in]
                n661 = property class="Bool (strict)"(reference=w901) -> ("Label.Text"=w900:string)  [unwired: 1 in, 2 out]
                n662 = case shown="\"PinR 3\"" w900 {
                  tunnel: [cluster{"Relay":T49, "Boolean":bool} {"Relay"=enum."R_Load", "Boolean"=FALSE} ("Relay") w908 w915 w926 w937 w948 w959 w970 w981 w992 w1003 w1014 w1025 w1036 w1043 w1052 w1061 w1070 w1079] -> w898
                  tunnel: [_ hw-control."Relay1" ("cmd") hw-control."Relay2" ("cmd") hw-control."Relay3" ("cmd") hw-control."Relay4" ("cmd") hw-control."Relay5" ("cmd") hw-control."Relay6" ("cmd") hw-control."Relay1" ("cmd") hw-control."Relay2" ("cmd") hw-control."Relay3" ("cmd") hw-control."Relay4" ("cmd") hw-control."Relay5" ("cmd") hw-control."Relay6" ("cmd") hw-control."Discharge" ("cmd") _ _ _ _ _] -> _
                  tunnel: [_ "PinR 1" "PinR 2" "PinR 3" "PinR 4" "PinR 5" "PinR 6" "PoutR 1" "PoutR 2" "PoutR 3" "PoutR 4" "PoutR 5" "PoutR 6" "Discharge R" _ _ _ _ _] -> _
                  tunnel: [_ TRUE TRUE TRUE TRUE TRUE TRUE TRUE TRUE TRUE TRUE TRUE TRUE TRUE _ _ _ _ _] -> _
                  frame "False", Default {
                  }
                  frame "PinR 1" {
                    n663 = case shown="True" "PinR 1" {
                      tunnel: [cluster{"Relay":T49, "Boolean":bool} {"Relay"=enum."R_in1", "Boolean"=FALSE} ("Relay") cluster{"Relay":T49, "Boolean":bool} {"Relay"=enum."R_in1", "Boolean"=TRUE} ("Relay")] -> w908
                      frame False {
                      }
                      frame True {
                      }
                    }
                  }
                  frame "PinR 2" {
                    n664 = case shown="True" "PinR 2" {
                      tunnel: [w916 w920] -> w915
                      tunnel: cluster{"Relay":T49, "Boolean":bool} {"Relay"=enum."R_in2", "Boolean"=TRUE} ("Relay") -> [w917 w921]
                      frame False {
                        n665 = Bundle By Name(cluster=w917, "Boolean"=FALSE) -> (w916:cluster{"Relay":T49, "Boolean":bool})
                      }
                      frame True {
                        n666 = Bundle By Name(cluster=w921, "Boolean"=TRUE) -> (w920:cluster{"Relay":T49, "Boolean":bool})
                      }
                    }
                  }
                  frame "PinR 3" {
                    n667 = case shown="False" "PinR 3" {
                      tunnel: [w927 w931] -> w926
                      tunnel: cluster{"Relay":T49, "Boolean":bool} {"Relay"=enum."R_in3", "Boolean"=TRUE} ("Relay") -> [w928 w932]
                      frame False {
                        n668 = Bundle By Name(cluster=w928, "Boolean"=FALSE) -> (w927:cluster{"Relay":T49, "Boolean":bool})
                      }
                      frame True {
                        n669 = Bundle By Name(cluster=w932, "Boolean"=TRUE) -> (w931:cluster{"Relay":T49, "Boolean":bool})
                      }
                    }
                  }
                  frame "PinR 4" {
                    n670 = case shown="True" "PinR 4" {
                      tunnel: [w938 w942] -> w937
                      tunnel: cluster{"Relay":T49, "Boolean":bool} {"Relay"=enum."R_in4", "Boolean"=TRUE} ("Relay") -> [w939 w943]
                      frame False {
                        n671 = Bundle By Name(cluster=w939, "Boolean"=FALSE) -> (w938:cluster{"Relay":T49, "Boolean":bool})
                      }
                      frame True {
                        n672 = Bundle By Name(cluster=w943, "Boolean"=TRUE) -> (w942:cluster{"Relay":T49, "Boolean":bool})
                      }
                    }
                  }
                  frame "PinR 5" {
                    n673 = case shown="False" "PinR 5" {
                      tunnel: [w949 w953] -> w948
                      tunnel: cluster{"Relay":T49, "Boolean":bool} {"Relay"=enum."R_in5", "Boolean"=TRUE} ("Relay") -> [w950 w954]
                      frame False {
                        n674 = Bundle By Name(cluster=w950, "Boolean"=FALSE) -> (w949:cluster{"Relay":T49, "Boolean":bool})
                      }
                      frame True {
                        n675 = Bundle By Name(cluster=w954, "Boolean"=TRUE) -> (w953:cluster{"Relay":T49, "Boolean":bool})
                      }
                    }
                  }
                  frame "PinR 6" {
                    n676 = case shown="True" "PinR 6" {
                      tunnel: [w960 w964] -> w959
                      tunnel: cluster{"Relay":T49, "Boolean":bool} {"Relay"=enum."R_in6", "Boolean"=TRUE} ("Relay") -> [w961 w965]
                      frame False {
                        n677 = Bundle By Name(cluster=w961, "Boolean"=FALSE) -> (w960:cluster{"Relay":T49, "Boolean":bool})
                      }
                      frame True {
                        n678 = Bundle By Name(cluster=w965, "Boolean"=TRUE) -> (w964:cluster{"Relay":T49, "Boolean":bool})
                      }
                    }
                  }
                  frame "PoutR 1" {
                    n679 = case shown="False" "PoutR 1" {
                      tunnel: [w971 w975] -> w970
                      tunnel: cluster{"Relay":T49, "Boolean":bool} {"Relay"=enum."R_out1", "Boolean"=TRUE} ("Relay") -> [w972 w976]
                      frame False {
                        n680 = Bundle By Name(cluster=w972, "Boolean"=FALSE) -> (w971:cluster{"Relay":T49, "Boolean":bool})
                      }
                      frame True {
                        n681 = Bundle By Name(cluster=w976, "Boolean"=TRUE) -> (w975:cluster{"Relay":T49, "Boolean":bool})
                      }
                    }
                  }
                  frame "PoutR 2" {
                    n682 = case shown="False" "PoutR 2" {
                      tunnel: [w982 w986] -> w981
                      tunnel: cluster{"Relay":T49, "Boolean":bool} {"Relay"=enum."R_out2", "Boolean"=TRUE} ("Relay") -> [w983 w987]
                      frame False {
                        n683 = Bundle By Name(cluster=w983, "Boolean"=FALSE) -> (w982:cluster{"Relay":T49, "Boolean":bool})
                      }
                      frame True {
                        n684 = Bundle By Name(cluster=w987, "Boolean"=TRUE) -> (w986:cluster{"Relay":T49, "Boolean":bool})
                      }
                    }
                  }
                  frame "PoutR 3" {
                    n685 = case shown="False" "PoutR 3" {
                      tunnel: [w993 w997] -> w992
                      tunnel: cluster{"Relay":T49, "Boolean":bool} {"Relay"=enum."R_out3", "Boolean"=TRUE} ("Relay") -> [w994 w998]
                      frame False {
                        n686 = Bundle By Name(cluster=w994, "Boolean"=FALSE) -> (w993:cluster{"Relay":T49, "Boolean":bool})
                      }
                      frame True {
                        n687 = Bundle By Name(cluster=w998, "Boolean"=TRUE) -> (w997:cluster{"Relay":T49, "Boolean":bool})
                      }
                    }
                  }
                  frame "PoutR 4" {
                    n688 = case shown="False" "PoutR 4" {
                      tunnel: [w1004 w1008] -> w1003
                      tunnel: cluster{"Relay":T49, "Boolean":bool} {"Relay"=enum."R_out4", "Boolean"=TRUE} ("Relay") -> [w1005 w1009]
                      frame False {
                        n689 = Bundle By Name(cluster=w1005, "Boolean"=FALSE) -> (w1004:cluster{"Relay":T49, "Boolean":bool})
                      }
                      frame True {
                        n690 = Bundle By Name(cluster=w1009, "Boolean"=TRUE) -> (w1008:cluster{"Relay":T49, "Boolean":bool})
                      }
                    }
                  }
                  frame "PoutR 5" {
                    n691 = case shown="False" "PoutR 5" {
                      tunnel: [w1015 w1019] -> w1014
                      tunnel: cluster{"Relay":T49, "Boolean":bool} {"Relay"=enum."R_out5", "Boolean"=TRUE} ("Relay") -> [w1016 w1020]
                      frame False {
                        n692 = Bundle By Name(cluster=w1016, "Boolean"=FALSE) -> (w1015:cluster{"Relay":T49, "Boolean":bool})
                      }
                      frame True {
                        n693 = Bundle By Name(cluster=w1020, "Boolean"=TRUE) -> (w1019:cluster{"Relay":T49, "Boolean":bool})
                      }
                    }
                  }
                  frame "PoutR 6" {
                    n694 = case shown="True" "PoutR 6" {
                      tunnel: [w1026 w1030] -> w1025
                      tunnel: cluster{"Relay":T49, "Boolean":bool} {"Relay"=enum."R_out6", "Boolean"=TRUE} ("Relay") -> [w1027 w1031]
                      frame False {
                        n695 = Bundle By Name(cluster=w1027, "Boolean"=FALSE) -> (w1026:cluster{"Relay":T49, "Boolean":bool})
                      }
                      frame True {
                        n696 = Bundle By Name(cluster=w1031, "Boolean"=TRUE) -> (w1030:cluster{"Relay":T49, "Boolean":bool})
                      }
                    }
                  }
                  frame "Discharge R" {
                    n697 = case shown="True" "Discharge R" {
                      tunnel: [w1037 w1041] -> w1036
                      tunnel: cluster{"Relay":T49, "Boolean":bool} {"Relay"=enum."R_Load", "Boolean"=TRUE} ("Relay") -> [w1038 w1042]
                      frame False {
                        n698 = Bundle By Name(cluster=w1038, "Boolean"=FALSE) -> (w1037:cluster{"Relay":T49, "Boolean":bool})
                      }
                      frame True {
                        n699 = Bundle By Name(cluster=w1042, "Boolean"=TRUE) -> (w1041:cluster{"Relay":T49, "Boolean":bool})
                      }
                    }
                  }
                  frame "led red" {
                    n700 = case shown="False" "led red" {
                      tunnel: [w1046 w1050] -> w1043
                      tunnel: cluster{"Relay":T49, "Boolean":bool} {"Relay"=enum."R_red", "Boolean"=TRUE} ("Relay") -> [w1047 w1051]
                      frame False {
                        n701 = Bundle By Name(cluster=w1047, "Boolean"=FALSE) -> (w1046:cluster{"Relay":T49, "Boolean":bool})
                      }
                      frame True {
                        n702 = Bundle By Name(cluster=w1051, "Boolean"=TRUE) -> (w1050:cluster{"Relay":T49, "Boolean":bool})
                      }
                    }
                  }
                  frame "led yellow" {
                    n703 = case shown="False" "led yellow" {
                      tunnel: [w1055 w1059] -> w1052
                      tunnel: cluster{"Relay":T49, "Boolean":bool} {"Relay"=enum."R_yellow", "Boolean"=TRUE} ("Relay") -> [w1056 w1060]
                      frame False {
                        n704 = Bundle By Name(cluster=w1056, "Boolean"=FALSE) -> (w1055:cluster{"Relay":T49, "Boolean":bool})
                      }
                      frame True {
                        n705 = Bundle By Name(cluster=w1060, "Boolean"=TRUE) -> (w1059:cluster{"Relay":T49, "Boolean":bool})
                      }
                    }
                  }
                  frame "led green" {
                    n706 = case shown="False" "led green" {
                      tunnel: [w1064 w1068] -> w1061
                      tunnel: cluster{"Relay":T49, "Boolean":bool} {"Relay"=enum."R_green", "Boolean"=TRUE} ("Relay") -> [w1065 w1069]
                      frame False {
                        n707 = Bundle By Name(cluster=w1065, "Boolean"=FALSE) -> (w1064:cluster{"Relay":T49, "Boolean":bool})
                      }
                      frame True {
                        n708 = Bundle By Name(cluster=w1069, "Boolean"=TRUE) -> (w1068:cluster{"Relay":T49, "Boolean":bool})
                      }
                    }
                  }
                  frame "led buz" {
                    n709 = case shown="False" "led buz" {
                      tunnel: [w1073 w1077] -> w1070
                      tunnel: cluster{"Relay":T49, "Boolean":bool} {"Relay"=enum."R_buz", "Boolean"=TRUE} ("Relay") -> [w1074 w1078]
                      frame False {
                        n710 = Bundle By Name(cluster=w1074, "Boolean"=FALSE) -> (w1073:cluster{"Relay":T49, "Boolean":bool})
                      }
                      frame True {
                        n711 = Bundle By Name(cluster=w1078, "Boolean"=TRUE) -> (w1077:cluster{"Relay":T49, "Boolean":bool})
                      }
                    }
                  }
                  frame "led purple" {
                    n712 = case shown="True" "led purple" {
                      tunnel: [w1082 w1086] -> w1079
                      tunnel: cluster{"Relay":T49, "Boolean":bool} {"Relay"=enum."R_purple", "Boolean"=TRUE} ("Relay") -> [w1083 w1087]
                      frame False {
                        n713 = Bundle By Name(cluster=w1083, "Boolean"=FALSE) -> (w1082:cluster{"Relay":T49, "Boolean":bool})
                      }
                      frame True {
                        n714 = Bundle By Name(cluster=w1087, "Boolean"=TRUE) -> (w1086:cluster{"Relay":T49, "Boolean":bool})
                      }
                    }
                  }
                }
                n715 = for {
                  tunnel: w899 -> [w903] mode=indexing
                  tunnel: w898 -> [w902]
                  n716 = call "fgv_DO-daqmx.vi"("cnt"=w903, "Relay"=w902) -> ()  [unwired: 9 in, 1 out]
                }
                n717 = global write "Global 1.vi" "Relay"(w898) -> ()
              }
            }
            n718 = Or(x=w206, y=w208) -> (x .or. y?=w207:bool)
          }
        }
        frame #15 {
          n719 = call "sub_log_basic.vi"("Title"="Shut down") -> ()  [unwired: 10 in, 1 out]
          n720 = call "sub_DO-all-off-raw-DAQmx.vi"() -> ()  [unwired: 12 in]
          n721 = call "sub_load-val.vi"("cmd"=enum16{"load", "save"}."save") -> ("error out"=w1092:errorcluster)  [unwired: 9 in, 1 out]
          n722 = call "fgv-data.vi"("cmd"=create-rw-close."close") -> ()  [unwired: 9 in, 2 out]
          n723 = call "fgv_params_save-load_manual.vi"("cmd"=T37."LastRUN Save", "error in"=w1092) -> ()  [unwired: 7 in, 3 out]
          n724 = call "fgv_DO-daqmx.vi"("cnt"=cnt_do."close") -> ()  [unwired: 10 in, 1 out]
        }
        frame #16 {
          n725 = global read "Glob_Ref.vi" "simulation"() -> (w1094:bool)
          n726 = case shown="True" w1094 {
            frame False {
            }
            frame True {
              n727 = control-ref of="This VI"() -> (w1096:refnum<vi>)
              n728 = property class="VI"(reference=w1096, "FP.State"=T58."Closed" ("Front Panel Window:State")) -> ()  [unwired: 1 in, 2 out]
            }
          }
        }
      }
    }
    frame True {
      n729 = global read "Glob_Ref.vi" "simulation"() -> (w1097:bool)
      n730 = case shown="True" w1097 {
        frame False {
        }
        frame True {
          n731 = control-ref of="This VI"() -> (w1099:refnum<vi>)
          n732 = property class="VI"(reference=w1099, "FP.State"=T58."Closed" ("Front Panel Window:State")) -> ()  [unwired: 1 in, 2 out]
        }
      }
    }
  }
